vi "runStudy2_2USRP_1ChNCS_3.vi"() -> (2 "Resp Amp":dbl[](graph), 3 "Heart Amp":dbl[](graph), 4 "# queue 2":i32)   [LabVIEW 2016]
uses:
  <instrlib>/niUSRP/niUSRP Timestamp.ctl
  <vilib>/Utility/miscctls.llb/LVDateTimeRec.ctl
  <vilib>/sound2/lvsound2.llb/Sound File Position.ctl
  <vilib>/Analysis/3filter.llb/Filter Passband Type.ctl
  <vilib>/sound2/lvsound2.llb/Sampling Mode.ctl
  <instrlib>/niUSRP/niUSRP Configure Time Start Trigger.vi
  <vilib>/Platform/browser.llb/Open URL in Default Browser (string).vi
  <instrlib>/niUSRP/niUSRP Write Tx Data (CDB).vi
  <instrlib>/niUSRP/niUSRP Fetch Rx Data (CDB).vi
  <vilib>/Analysis/3filter.llb/Butterworth Filter (DBL).vi
  <vilib>/sound2/lvsound2.llb/Sound File Info (path).vi
  <vilib>/sound2/lvsound2.llb/Sound File Read Open.vi
  <vilib>/sound2/lvsound2.llb/Sound File Read (DBL).vi
  <vilib>/sound2/lvsound2.llb/Sound Output Write (DBL).vi
  <vilib>/Analysis/3filter.llb/Butterworth Filter (CDB).vi
  <vilib>/measure/NI_MABase.lvlib
  <vilib>/Analysis/NI_AALBase.lvlib
  <vilib>/Analysis/NI_AALPro.lvlib
panel:
  in  "SDR1\nInitPhase":i32
  in  "Flush Rx2":bool
  out "String 3":string
  out "element":dbl[][](array[numeric])
  out "appended array":dbl[][](array[numeric])
  in  "SDR2 Carrier \nfrequency (Hz)":dbl=1900000000.0
  out "String 2":string
  out "size(s)":i32[](array[numeric])
  in  "Tab Control 7":enum32{"Amp2 @50kHz", "Ph2 @50kHz"}(tab)
  out "Amp2 @50 kHz":dbl[](graph)
  out "Ph2 @50 kHz":dbl[](graph)
  in  "Tab Control 6":enum32{"Amp1 @500Hz", "Ph1 @500Hz"}(tab)
  out "Amp1 @500Hz":dbl[](graph)
  out "Ph1 @500Hz":dbl[](graph)
  out "String":string
  out "#queue 3":i32
  out "#queue 2":i32
  out "# Rx2DS_Queue":i32
  in  "FlushSDR2":bool
  out "error out 2":errorcluster
  in  "Tab Control 8":enum32{"Rx1", "Rx2"}(tab)
  out "IQ Graph":dbl[][](graph)
  out "IQ Graph 2":dbl[][](graph)
  in  "Tab Control 5":enum32{"Amp2 @500Hz", "Ph2 @500Hz"}(tab)
  out "Amp2 @500Hz":dbl[](graph)
  out "Ph2 @500Hz":dbl[](graph)
  in  "Tab Control 4":enum32{"Tx1", "Tx2"}(tab)
  out "Tx1 Waveform Graph":waveform(dbl)[](graph)
  out "Tx2 Waveform graph":waveform(dbl)[](graph)
  in  "Stop 2":bool
  out "Tx2 Waveform":cdb[](array[numeric])
  out "Read:Tx2 IQ Rate":dbl=5000000.0
  out "Read:Rx2 IQ Rate":dbl=5000000.0
  in  "Device2 Name":refnum<k15>="B200mini"
  in  "Tx2 Gain":dbl=26.0 format="%#_6f"
  in  "Rx2 Gain":dbl=20.0 format="%#_6f"
  in  "Routine 3,4":T1=2 items=["Absolute"=0, "Relative"=2]
  in  "(2b) Attn Test":T1=2 items=["Absolute"=0, "Relative"=2]
  in  "Routine 5":T1=2 items=["Absolute"=0, "Relative"=2]
  in  "OpenHTML":bool=TRUE
  in  "Play sound":u16(ring) items=["No sound", "Demo normal breathing", "Demo deep breathing", "Demo fast shallow breathing", "Demo breath hold", "Demo cough", "Demo abdomen movement", "Calibration", "Routine 1", "(2a) Calm music", "(2b) Stress test", "Routine 3/4", "Routine 5"]
  in  "Demo cough":T1=2 items=["Absolute"=0, "Relative"=2]
  in  "Demo breath-hold":T1=2 items=["Absolute"=0, "Relative"=2]
  in  "Demo abdomen":T1=2 items=["Absolute"=0, "Relative"=2]
  in  "Demo fast shallow":T1=2 items=["Absolute"=0, "Relative"=2]
  in  "Play/Stop":bool
  in  "Demo normal":T1=2 items=["Absolute"=0, "Relative"=2]
  in  "Demo deep":T1=2 items=["Absolute"=0, "Relative"=2]
  out "Next Task":string
  out "Calib 5":bool caption="Time has Elapsed"
  out "Calib 4":bool caption="Time has Elapsed"
  out "Calib 3":bool caption="Time has Elapsed"
  in  "Calibration":T1=2 items=["Absolute"=0, "Relative"=2]
  out "Calib 1":bool caption="Time has Elapsed"
  out "Current Task time":dbl(slide) scale=0.0..120.0
  in  "(2a) Calm Music":T1=2 items=["Absolute"=0, "Relative"=2]
  out "#2b":bool caption="Time has Elapsed"
  in  "Routine 1":T1=2 items=["Absolute"=0, "Relative"=2]
  in  "number of samples/ch":i32=5000
  out "#5":bool caption="Time has Elapsed"
  out "#2a":bool caption="Time has Elapsed"
  out "#4":bool caption="Time has Elapsed"
  out "#3":bool caption="Time has Elapsed"
  in  "Comments":string
  in  "Tab Control 3":enum32{"Amp Heart", "Ph Heart"}(tab)
  in  "fh 1":dbl=26.0 format="%0.2f"
  in  "fl 1":dbl=0.7 format="%0.4f"
  out "Heart Ph":dbl[](graph)
  in  "fl 3":dbl=0.7 format="%0.4f"
  in  "fh 3":dbl=26.0 format="%0.2f"
  in  "Tab Control 2":enum32{"Amp1 @50kHz", "Ph1 @50kHz"}(tab)
  out "Amp1 @50 kHz":dbl[](graph)
  out "Ph1 @50 kHz":dbl[](graph)
  in  "Tab Control":enum32{"Amp Resp", "Ph Resp"}(tab)
  in  "fl 2":dbl=15.0 format="%0.4f"
  out "Resp Ph":dbl[](graph)
  in  "fl 4":dbl=15.0 format="%0.4f"
  out "ArraySz":i32[](array[numeric])
  in  "Stop Test":bool
  out "#1":bool caption="Time has Elapsed"
  out "Elapsed Time (s)":dbl
  in  "Routine":u16(ring) items=["Not Running", "Test Run", "Routine1", "Routine2a", "Routine2b", "Routine3", "Routine4", "Routine5", "Calib1", "calib3", "Calib4", "Calib5"]
  out "Read:Tx IQ Rate":dbl=5000000.0
  out "Read:Rx IQ Rate":dbl=5000000.0
  out "date time rec":T2
  out "Total Routine Time":dbl(slide) scale=0.0..420.0
  out "Current Task":string
  in  "Case Number":string="0"
  out "CaseNum":i32=1
  out "Save":bool
  out "Flush":bool
  out "Buffer":bool
  out "Output":i32=1
  out "Ch2 Amplitude":dbl=0.5 step=0.05 format="%#.6g"
  out "Ch1 Amplitude":dbl=0.5 step=0.05 format="%#.6g"
  out "Dis Sampling Rate":dbl=500.0 format="%#_6p"
  in  "DownSamplingRatio 2":i32=100
  out "Sampling Rate":dbl=50000.0 format="%#_6p"
  out "aapp":dbl[][](array[numeric])
  out "IterationNum":i32=1009
  in  "DownSamplingRatio":i32=40
  out "# elements in queue":i32
  out "BW/2":dbl=1000.0
  out "# queue 1":i32
  in  "Dis1":bool=TRUE
  out "Tx1 Waveform":cdb[](array[numeric])
  in  "SDR1 Carrier\nfrequency [Hz]":dbl=1820000000.0 format="%#_6p"
  out "error out":errorcluster
  in  "Start Trigger Time":T3={"whole seconds"=1, "fractional seconds"=0.0}
  in  "Stop":bool
  in  "Channel 2\nTone Amplitude":dbl=0.5 step=0.05 format="%#.6g"
  in  "SDR2\nTone Frequency":dbl=51000.0 format="%#_6p"
  in  "Channel 1\nTone Amplitude":dbl=0.5 step=0.05 format="%#.6g"
  in  "SDR1 \nTone Frequency":dbl=51000.0 format="%#_6p"
  in  "Waveform Size":dbl=20000.0
  in  "Device1 Name":refnum<k15>="MyB200"
  in  "Tx1 Gain":dbl=25.0 format="%#_6f"
  in  "Tx IQ Rate":dbl=2000000.0 format="%#_6p"
  in  "Rx1 Gain 1":dbl=26.0 format="%#_6f"
  in  "Rx IQ Rate":dbl=2000000.0 format="%#_6p"
  # "User Instructions"
  # "User Information"
  # "Routine Selection"
  # "Demo \nSounds"
  # "First Tx-Rx: filtered to get heartbeat signal"
  # "Second Tx-Rx: filtered to get respiration signal"
  # "SDR1"
  # "SDR2"
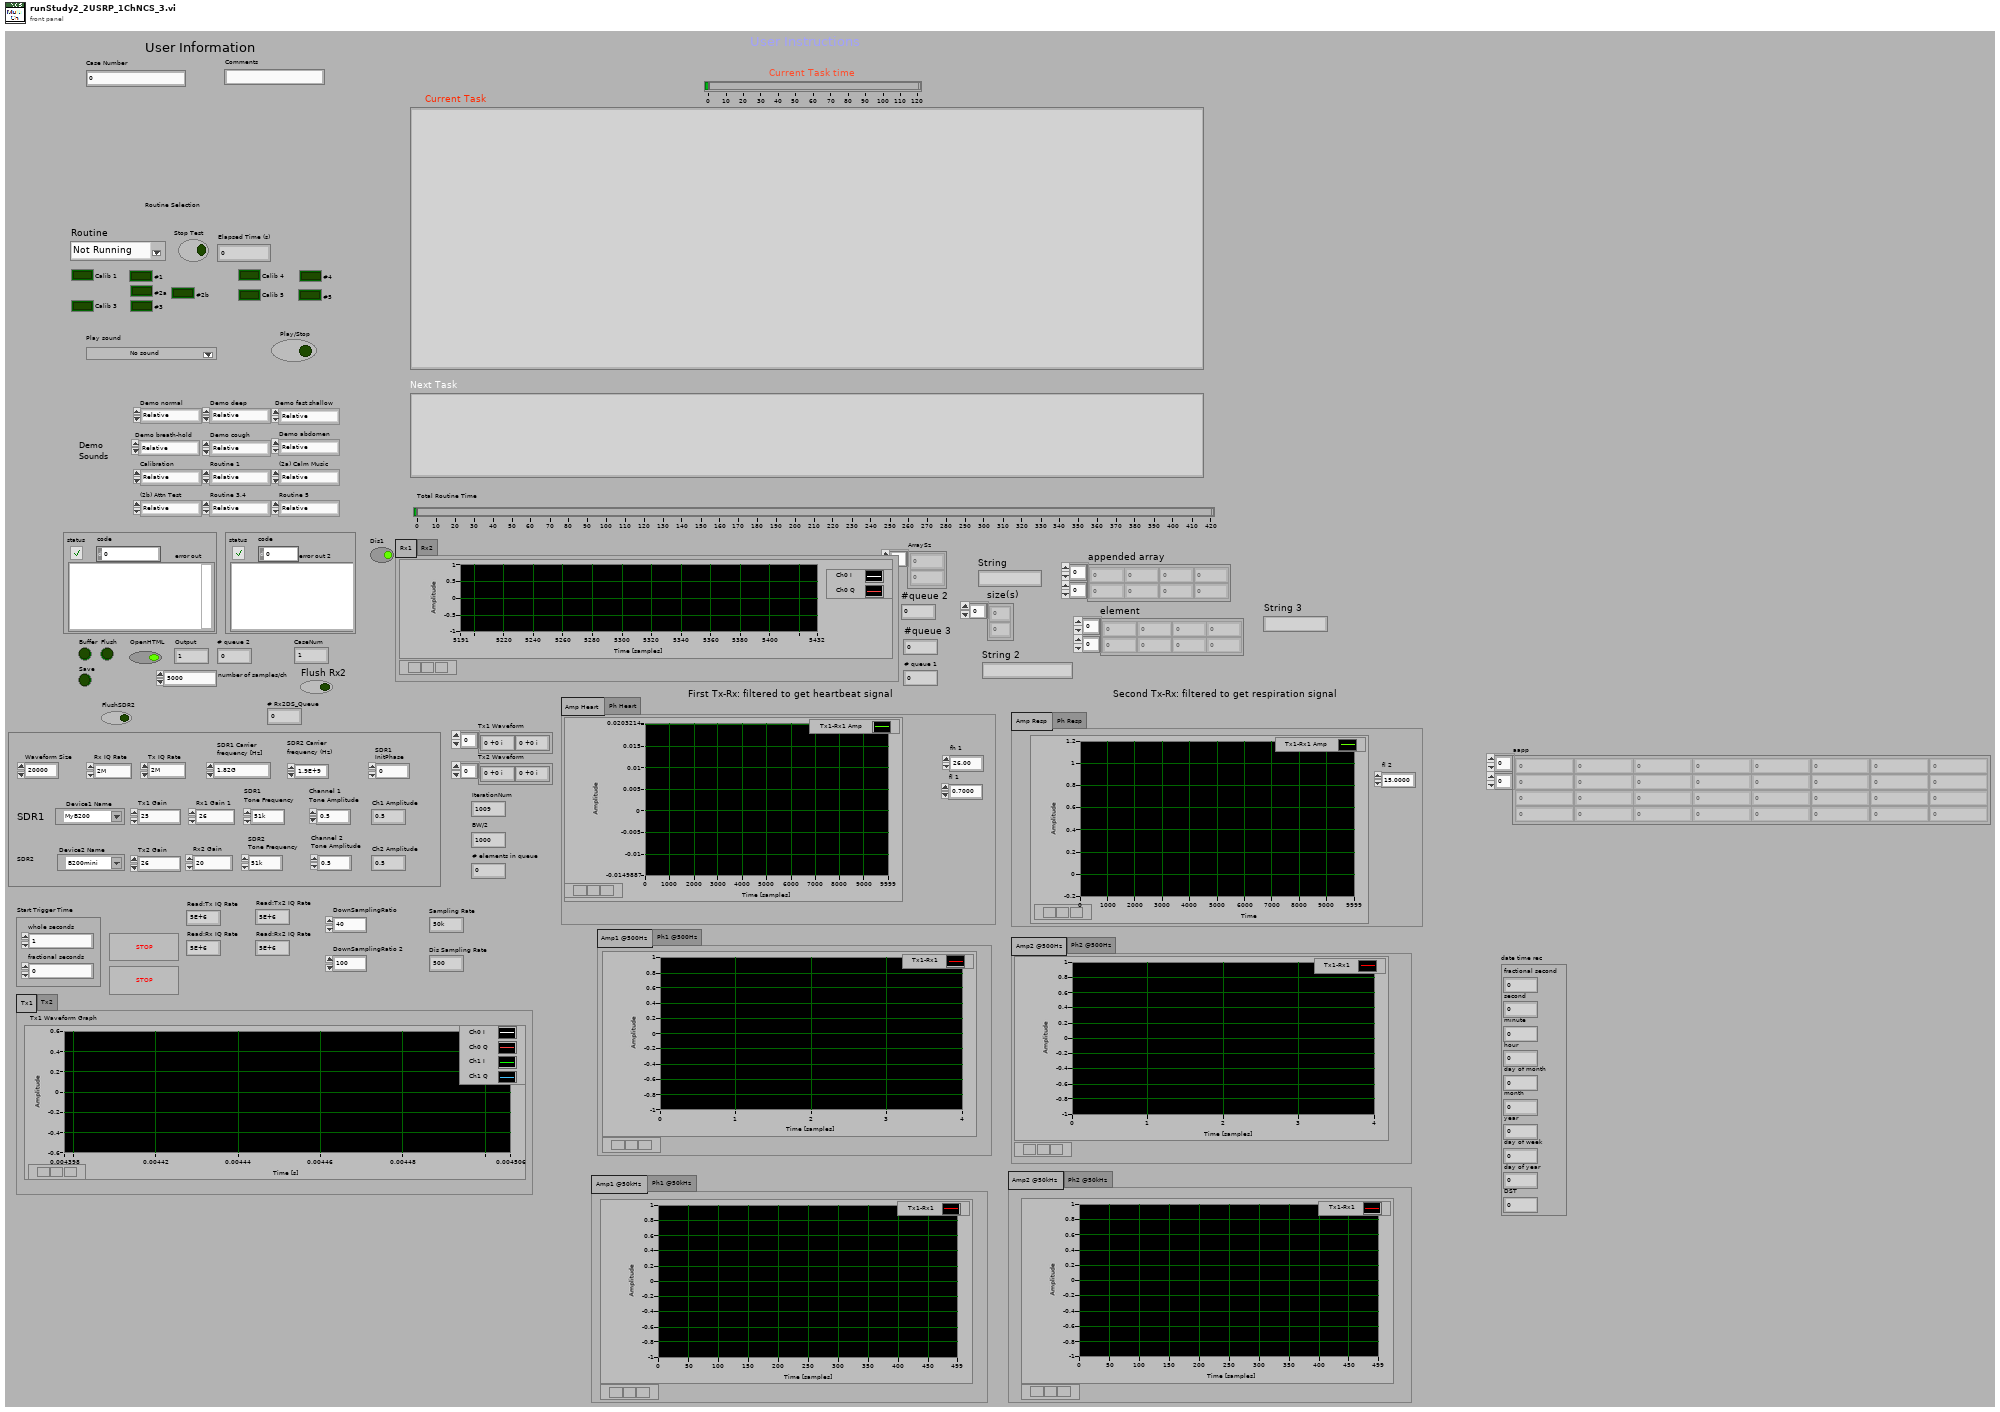
[diagram p1: front panel]
types:
  T1 = typedef "Sound File Position.ctl" = u16
  T2 = typedef "LVDateTimeRec.ctl" = cluster{"fractional second":dbl, "second":i32, "minute":i32, "hour":i32, "day of month":i32, "month":i32, "year":i32, "day of week":i32, "day of year":i32, "DST":i32}
  T3 = typedef "niUSRP Timestamp.ctl" = cluster{"whole seconds":u64, "fractional seconds":dbl}
  T4 = enum16{"Default", "Test", "Routine 1", "Routine 2a", "Routine 2b", "Routine 3", "Routine 4", "Routine 5", "Calib1", "Calib3", "Calib4", "Calib5"}
  T5 = typedef "Sampling Mode.ctl" = i32
  T6 = typedef "Sound Data Format.ctl" = cluster{"sample rate (S/s)":dbl, "number of channels":i32, "bits per sample":i32}
  T7 = typedef "Sound File Refnum.ctl" = refnum<file>
  T8 = typedef "Sound Output Task ID.ctl" = u32
  T9 = typedef "NI_AALBase.lvlib/Filter Passband Type.ctl" = enum32{"Lowpass", "Highpass", "Bandpass", "Bandstop"}
  T10 = enum16{"Default", "Test", "Routine 1", "Routine 2", "Routine 3"}
  T11 = enum16{"Default", "Test", "Routine 1", "Routine 2a", "Routine 2b", "Routine 3a", "Routine 3b", "Routine 4", "Routine 5", "Routine 6", "Routine 7", "Calib1", "Calib3", "Calib4", "Calib5", "Calib7"}
  T12 = enum16{"open", "open or create", "create or replace", "create", "open (read-only)"}
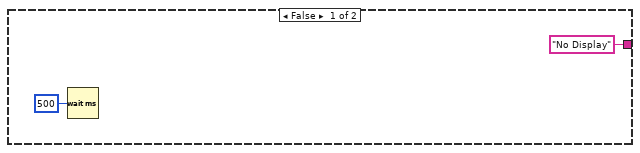
[diagram p2: hidden frame]
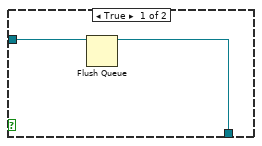
[diagram p3: hidden frame]
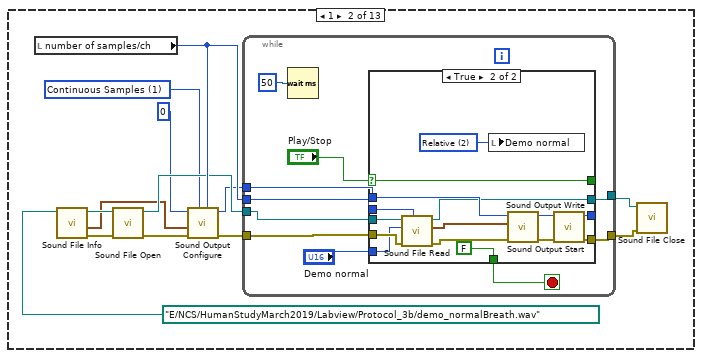
[diagram p5: hidden frame]
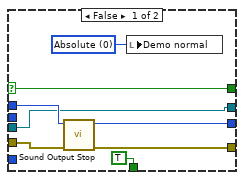
[diagram p6: hidden frame]
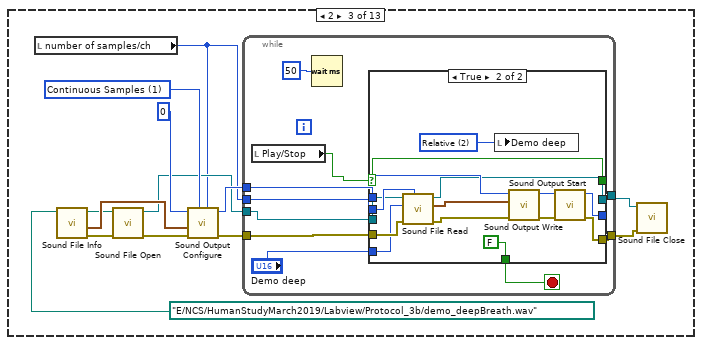
[diagram p7: hidden frame]
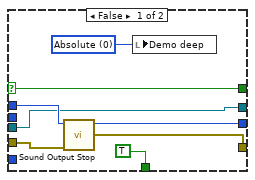
[diagram p8: hidden frame]
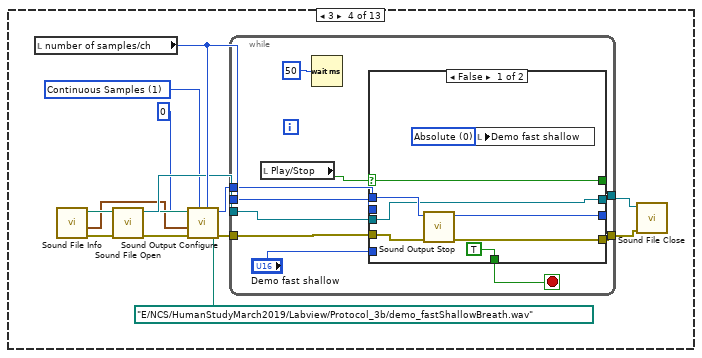
[diagram p9: hidden frame]
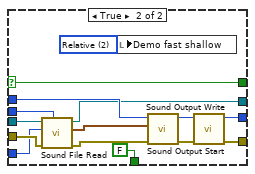
[diagram p10: hidden frame]
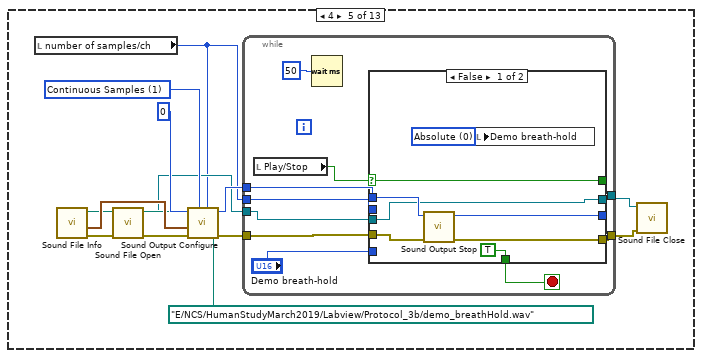
[diagram p11: hidden frame]
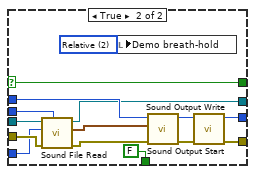
[diagram p12: hidden frame]
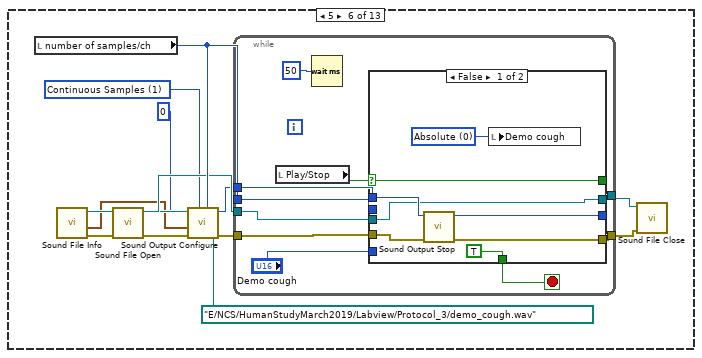
[diagram p13: hidden frame]
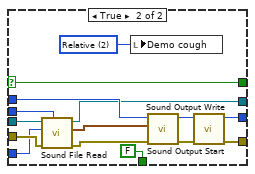
[diagram p14: hidden frame]
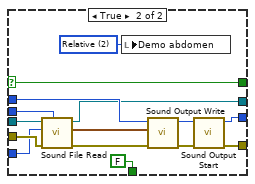
[diagram p15: hidden frame]
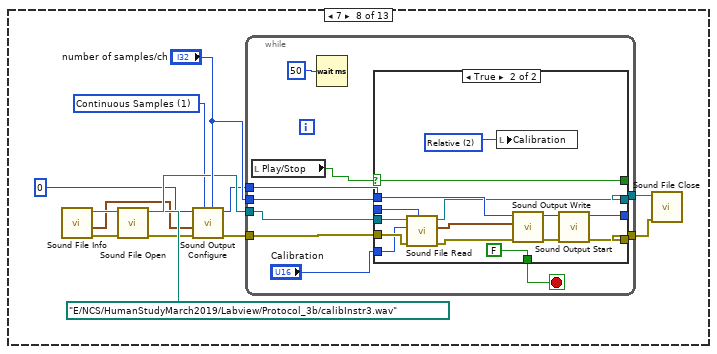
[diagram p16: hidden frame]
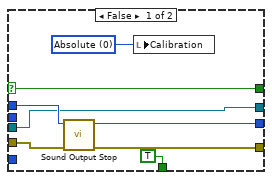
[diagram p17: hidden frame]
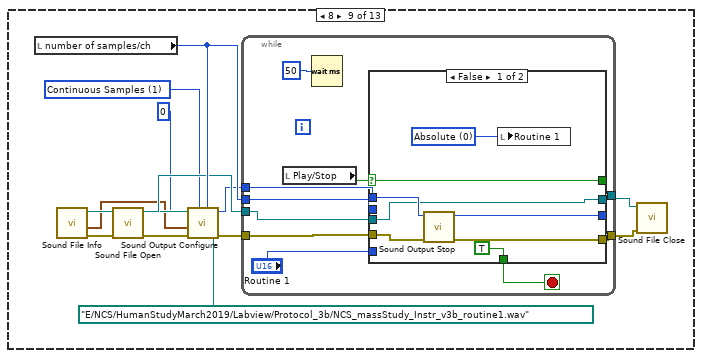
[diagram p18: hidden frame]
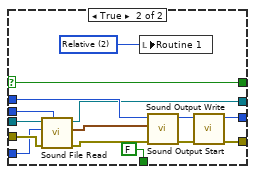
[diagram p19: hidden frame]
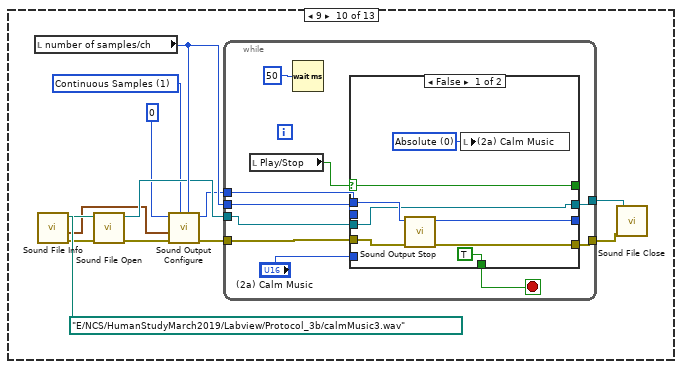
[diagram p20: hidden frame]
diagram:
  w29 = 1 items=["Now", "Next Timebase Edge"] ("apply timestamp")
  w37 = "RX2"  # Rx2 active antenna
  w95 = 0.0 ("element")
  w96 = 2000 ("dimension size")
  w103 = 4 ("dimension size")
  w130 = "RX2"  # Rx1 active antenna
  w164 = 1 items=["Now", "Next Timebase Edge"] ("apply timestamp")
  w78 = "TX1"  # Tx active antenna
  w85 = "0"  # Enabled Channels
  # "Tx2 Chain"
  # "Rx2 chain"
  # "Set the attributes \nspecific to channel 0."
  # "Set the attributes \nused by all Rx channels"
  # "Set the attributes \nspecific to Rx channel 0."
  # "Tx1 Chain"
  # "Rx1 chain"
  # "DownSamplingRatio"
  # "Set the attributes \nspecific to channel 0."
  # "Set the attributes \nused by both Rx channels"
  # "Set the attributes \nspecific to Rx channel 0."
  n1 = while {
    stop <- FALSE stop-if-true
    n2 = local read "Output"() -> (w174:i32)
    n3 = case shown="1" w174 {
      tunnel: [w179 "Channel 1\nTone Amplitude"] -> w176
      tunnel: [w179 "Channel 2\nTone Amplitude"] -> w175
      frame 0, Default {
        w179 = 0.0 ("Channel 1\nTone Amplitude")
      }
      frame 1 {
      }
    }
    "Ch1 Amplitude" <- w176
    "Ch2 Amplitude" <- w175
    n4 = Wait (ms)(milliseconds to wait=u32 50) -> ()  [unwired: 1 out]
  }
  n5 = local read "Device2 Name"() -> (w60:refnum<k15>)
  n6 = local read "Device1 Name"() -> (w169:refnum<k15>)
  n7 = call <instrlib>:"niUSRP Open Rx Session.vi"("device names"="Device2 Name") -> ("session handle out"=w59:refnum<k15>, "error out"=w58:errorcluster)  [unwired: 13 in]
  n8 = property class="niUSRP"(reference=w59, error in=w58, "Enabled Channels"=w85) -> (reference out=w57:refnum<k15>, error out=w56:errorcluster)
  n9 = call <instrlib>:"niUSRP Open Rx Session.vi"("device names"="Device1 Name") -> ("session handle out"=w163:refnum<k15>, "error out"=w162:errorcluster)  [unwired: 13 in]
  n10 = property class="niUSRP"(reference=w163, error in=w162, "Enabled Channels"=w85) -> (reference out=w161:refnum<k15>, error out=w160:errorcluster)
  n11 = call-poly <instrlib>:"niUSRP Configure Trigger.vi"("session handle"=w57, "start trigger time"="Start Trigger Time", "error in (no error)"=w56) -> ("session handle out"=w53:refnum<k15>, "error out"=w52:errorcluster)  [unwired: 11 in]
  n12 = call-poly <instrlib>:"niUSRP Configure Trigger.vi"("session handle"=w161, "start trigger time"="Start Trigger Time", "error in (no error)"=w160) -> ("session handle out"=w157:refnum<k15>, "error out"=w156:errorcluster)  [unwired: 11 in]
  n13 = property class="niUSRP"(reference=w53, error in=w52, "IQ Rate"="Rx IQ Rate") -> (reference out=w50:refnum<k15>, error out=w51:errorcluster)
  n14 = property class="niUSRP"(reference=w157, error in=w156, "IQ Rate"="Rx IQ Rate") -> (reference out=w154:refnum<k15>, error out=w155:errorcluster)
  n15 = property class="niUSRP" props=["Model"](reference=w50, error in=w51) -> (reference out=w48:refnum<k15>, error out=w49:errorcluster)  [unwired: 1 out]
  n16 = property class="niUSRP" props=["Model"](reference=w154, error in=w155) -> (reference out=w152:refnum<k15>, error out=w153:errorcluster)  [unwired: 1 out]
  n17 = property class="niUSRP"(reference=w48, error in=w49, "Carrier Frequency"="SDR2 Carrier \nfrequency (Hz)") -> (reference out=w42:refnum<k15>, error out=w41:errorcluster, "IQ Rate"=→"Read:Rx2 IQ Rate":dbl)
  n18 = property class="niUSRP"(reference=w152, error in=w153, "Carrier Frequency"="SDR1 Carrier\nfrequency [Hz]") -> (reference out=w135:refnum<k15>, error out=w134:errorcluster, "IQ Rate"=→"Read:Rx IQ Rate":dbl)
  n19 = property class="niUSRP"(reference=w42, error in=w41, "Active Channel"="0", "Gain"="Rx2 Gain", "Active Antenna"=w37) -> (reference out=w25:refnum<k15>, error out=w26:errorcluster)
  n20 = call <instrlib>:"niUSRP Open Tx Session.vi"("device names"=w60, "error in (no error)"=w26) -> ("session handle out"=w55:refnum<k15>, "error out"=w54:errorcluster)  [unwired: 12 in]
  n21 = property class="niUSRP"(reference=w55, error in=w54, "Enabled Channels"=w85) -> (reference out=w46:refnum<k15>, error out=w45:errorcluster)
  n22 = property class="niUSRP" props=["IQ Rate", "IQ Rate"](reference=w46, error in=w45, "IQ Rate"="Tx IQ Rate") -> (reference out=w35:refnum<k15>, error out=w34:errorcluster)  [unwired: 1 out]
  n23 = property class="niUSRP"(reference=w35, error in=w34, "Carrier Frequency"="SDR2 Carrier \nfrequency (Hz)") -> (reference out=w39:refnum<k15>, error out=w38:errorcluster, "IQ Rate"=w10:dbl)
  "Read:Tx2 IQ Rate" <- w10
  n24 = property class="niUSRP"(reference=w39, error in=w38, "Active Channel"="0", "Gain"="Tx2 Gain", "Active Antenna"=w78) -> (reference out=w33:refnum<k15>, error out=w32:errorcluster)
  n25 = property class="niUSRP"(reference=w135, error in=w134, "Active Channel"="0", "Gain"="Rx1 Gain 1", "Active Antenna"=w130) -> (reference out=w81:refnum<k15>, error out=w80:errorcluster)
  n26 = call <instrlib>:"niUSRP Open Tx Session.vi"("device names"=w169, "error in (no error)"=w80) -> ("session handle out"=w159:refnum<k15>, "error out"=w158:errorcluster)  [unwired: 12 in]
  n27 = property class="niUSRP"(reference=w159, error in=w158, "Enabled Channels"=w85) -> (reference out=w150:refnum<k15>, error out=w149:errorcluster)
  n28 = property class="niUSRP"(reference=w150, error in=w149, "IQ Rate"="Tx IQ Rate") -> (reference out=w87:refnum<k15>, error out=w86:errorcluster, "IQ Rate"=w148:dbl)
  n29 = property class="niUSRP"(reference=w87, error in=w86, "Carrier Frequency"="SDR1 Carrier\nfrequency [Hz]") -> (reference out=w132:refnum<k15>, error out=w131:errorcluster, "IQ Rate"=→"Read:Tx IQ Rate":dbl)
  n30 = property class="niUSRP"(reference=w132, error in=w131, "Active Channel"="0", "Gain"="Tx1 Gain", "Active Antenna"=w78) -> (reference out=w82:refnum<k15>, error out=w83:errorcluster)
  n31 = call <instrlib>:"niUSRP Commit.vi"("session handle"=w33, "error in (no error)"=w32) -> ("session handle out"=w7:refnum<k15>, "error out"=w24:errorcluster)  [unwired: 12 in]
  n32 = call <instrlib>:"niUSRP Commit.vi"("session handle"=w82, "error in (no error)"=w83) -> ("session handle out"=w171:refnum<k15>, "error out"=w172:errorcluster)  [unwired: 12 in]
  n33 = Merge Errors(w26, w24) -> (w27:errorcluster)
  n34 = call <instrlib>:"niUSRP Set Time.vi"("session handle"=w25, "apply timestamp"=w29, "timestamp"=T3 {"whole seconds"=0, "fractional seconds"=0.0}, "error in (no error)"=w27) -> ("session handle out"=w31:refnum<k15>, "error out"=w30:errorcluster)  [unwired: 10 in]
  n35 = call <instrlib>:"niUSRP Initiate.vi"("session handle"=w31, "error in (no error)"=w30) -> ("session handle out"=w11:refnum<k15>, "error out"=w1:errorcluster)  [unwired: 12 in]
  n36 = Merge Errors(w80, w172) -> (w100:errorcluster)
  n37 = local read "Waveform Size"() -> (w12:dbl)
  n38 = Initialize Array(cdb 0.0+0.0i ("element"), w12) -> (w14:cdb[])
  n39 = call <instrlib>:"niUSRP Set Time.vi"("session handle"=w81, "apply timestamp"=w164, "timestamp"=T3 {"whole seconds"=0, "fractional seconds"=0.0}, "error in (no error)"=w100) -> ("session handle out"=w166:refnum<k15>, "error out"=w165:errorcluster)  [unwired: 10 in]
  n40 = Obtain Queue(max queue size (-1, unlimited)=-1, name (unnamed)="Rx2Queue", element data type=w14) -> (queue out=w71:refnum<queue>)  [unwired: 2 in, 2 out]
  n41 = local read "Waveform Size"() -> (w90:dbl)
  n42 = call <instrlib>:"niUSRP Initiate.vi"("session handle"=w166, "error in (no error)"=w165) -> ("session handle out"=w173:refnum<k15>, "error out"=w88:errorcluster)  [unwired: 12 in]
  n43 = while {
    tunnel: w148 -> [w192]
    tunnel: w88 -> [w187]
    stop <- FALSE stop-if-true
    # "Generate I and Q waveforms."
    n44 = Wait (ms)(milliseconds to wait=u32 100) -> ()  [unwired: 1 out]
    n45 = local read "Ch1 Amplitude"() -> (w186:dbl)
    n46 = Bundle By Name(cluster=cluster{"Fs":dbl, "#s":dbl} {"Fs"=1000.0, "#s"=1000.0} ("sampling info"), "Fs"=w192, "#s"="Waveform Size") -> (w193:cluster{"Fs":dbl, "#s":dbl})
    n47 = Add(x=90.0 ("phase"), y="SDR1\nInitPhase") -> (x+y=w183:dbl)
    n48 = call <vilib>:"Sine Waveform.vi"("sampling info"=w193, "error in (no error)"=w187, "phase"=w183, "amplitude"=w186, "frequency"="SDR1 \nTone Frequency") -> ("error out"=w190:errorcluster, "signal out"=w197:waveform(dbl))  [unwired: 5 in]
    n49 = call <vilib>:"Sine Waveform.vi"("sampling info"=w193, "error in (no error)"=w187, "phase"="SDR1\nInitPhase", "amplitude"=w186, "frequency"="SDR1 \nTone Frequency") -> ("error out"=w191:errorcluster, "signal out"=w198:waveform(dbl))  [unwired: 5 in]
    n50 = Merge Errors(w190, w191) -> ()  [unwired: 1 out]
    n51 = Build Array(w197, w198) -> (→"Tx1 Waveform Graph":waveform(dbl)[])
    n52 = Unbundle By Name(w197) -> ("Y"=w196:dbl[])
    n53 = Unbundle By Name(w198) -> ("Y"=w195:dbl[])
    n54 = Re/Im To Complex(1:w195, 2:w196) -> (0:→"Tx1 Waveform":cdb[])
  }
  n55 = while {
    tunnel: w71 -> [w204]
    stop <- FALSE stop-if-true
    n56 = local read "Dis1"() -> (w203:bool)
    n57 = Wait (ms)(milliseconds to wait=u32 5) -> ()  [unwired: 1 out]
    n58 = case shown="True" w203 {
      tunnel: w204 -> [_ w211]
      tunnel: ["No Display" "Displaying Rx2 "] -> w202
      frame False {
        n59 = Wait (ms)(milliseconds to wait=u32 500) -> ()  [unwired: 1 out]
      }
      frame True {
        n60 = Preview Queue Element(queue=w211) -> (element=w213:cdb[])  [unwired: 2 in, 3 out]
        n61 = for {
          N: 1 -> [_]
          tunnel: w213 -> [w219]
          shift-right: [w216] -> w212
          shift-left: dbl[][] [] -> [w215]
          n62 = Complex To Re/Im(x + iy=w219) -> (x=w218:dbl[], y=w217:dbl[])
          n63 = Build Array (concatenate)(w215, w218, w217) -> (w216:dbl[][])
        }
        "IQ Graph 2" <- w212
      }
    }
    "String" <- w202
  }
  n64 = while {
    tunnel: w11 -> [w231]
    tunnel: w1 -> [w230]
    tunnel: [w226] -> w21
    tunnel: [w229] -> w18
    shift-right: [w222] -> _
    shift-left: w71 -> [w223]
    stop <- w225 stop-if-true
    # "Rx2"
    n65 = local read "Waveform Size"() -> (w224:dbl)
    n66 = call-poly <instrlib>:"niUSRP Fetch Rx Data (poly).vi"("session handle"=w231, "number of samples"=w224, "error in (no error)"=w230) -> ("session handle out"=w229:refnum<k15>, "data"=w220:cdb[], "timestamp"=w221:T3, "error out"=w226:errorcluster)  [unwired: 9 in]
    n67 = call <instrlib>:"niUSRP USRP Timestamp to LV Timestamp.vi"("USRP Timestamp"=w221) -> ()  [unwired: 13 in, 2 out]
    n68 = Enqueue Element(queue=w223, element=w220) -> (queue out=w222:refnum<queue>)  [unwired: 2 in, 2 out]
    n69 = Unbundle By Name(w226) -> ("status"=w228:bool)
    n70 = Or(x=w228, y="Stop 2") -> (x .or. y?=w225:bool)
  }
  n71 = while {
    tunnel: w10 -> [w241]
    tunnel: w1 -> [w232]
    stop <- FALSE stop-if-true
    # "Generate I and Q waveforms."
    n72 = local read "Waveform Size"() -> (w233:dbl)
    n73 = Wait (ms)(milliseconds to wait=u32 100) -> ()  [unwired: 1 out]
    n74 = Bundle By Name(cluster=cluster{"Fs":dbl, "#s":dbl} {"Fs"=1000.0, "#s"=1000.0} ("sampling info"), "Fs"=w241, "#s"=w233) -> (w242:cluster{"Fs":dbl, "#s":dbl})
    n75 = local read "Ch2 Amplitude"() -> (w236:dbl)
    n76 = call <vilib>:"Sine Waveform.vi"("sampling info"=w242, "error in (no error)"=w232, "phase"=90.0, "amplitude"=w236, "frequency"="SDR2\nTone Frequency") -> ("error out"=w239:errorcluster, "signal out"=w247:waveform(dbl))  [unwired: 5 in]
    n77 = call <vilib>:"Sine Waveform.vi"("sampling info"=w242, "error in (no error)"=w232, "amplitude"=w236, "frequency"="SDR2\nTone Frequency") -> ("error out"=w240:errorcluster, "signal out"=w248:waveform(dbl))  [unwired: 6 in]
    n78 = Merge Errors(w239, w240) -> ()  [unwired: 1 out]
    n79 = Build Array(w247, w248) -> (→"Tx2 Waveform graph":waveform(dbl)[])
    n80 = Unbundle By Name(w247) -> ("Y"=w246:dbl[])
    n81 = Unbundle By Name(w248) -> ("Y"=w245:dbl[])
    n82 = Re/Im To Complex(1:w245, 2:w246) -> (0:→"Tx2 Waveform":cdb[])
  }
  n83 = Initialize Array(cdb 0.0+0.0i ("element"), w90) -> (w127:cdb[])
  n84 = Obtain Queue(max queue size (-1, unlimited)=-1, name (unnamed)="Rx1Queue", element data type=w127) -> (queue out=w91:refnum<queue>)  [unwired: 2 in, 2 out]
  n85 = while {
    tunnel: w173 -> [w261]
    tunnel: w88 -> [w260]
    tunnel: [w256] -> w144
    tunnel: [w259] -> w141
    shift-right: [w252] -> _
    shift-left: w91 -> [w253]
    stop <- w255 stop-if-true
    # "Rx"
    n86 = local read "Waveform Size"() -> (w254:dbl)
    n87 = call-poly <instrlib>:"niUSRP Fetch Rx Data (poly).vi"("session handle"=w261, "number of samples"=w254, "error in (no error)"=w260) -> ("session handle out"=w259:refnum<k15>, "data"=w250:cdb[], "timestamp"=w251:T3, "error out"=w256:errorcluster)  [unwired: 9 in]
    n88 = call <instrlib>:"niUSRP USRP Timestamp to LV Timestamp.vi"("USRP Timestamp"=w251) -> ()  [unwired: 13 in, 2 out]
    n89 = Enqueue Element(queue=w253, element=w250) -> (queue out=w252:refnum<queue>)  [unwired: 2 in, 2 out]
    n90 = Unbundle By Name(w256) -> ("status"=w258:bool)
    n91 = Or(x=w258, y="Stop") -> (x .or. y?=w255:bool)
  }
  n92 = while {
    tunnel: w91 -> [w263]
    stop <- FALSE stop-if-true
    n93 = Wait (ms)(milliseconds to wait=u32 5) -> ()  [unwired: 1 out]
    n94 = case shown="True" "Dis1" {
      tunnel: w263 -> [_ w268]
      frame False {
        n95 = Wait (ms)(milliseconds to wait=u32 500) -> ()  [unwired: 1 out]
      }
      frame True {
        n96 = Preview Queue Element(queue=w268) -> (element=w270:cdb[])  [unwired: 2 in, 3 out]
        n97 = for {
          N: 1 -> [_]
          tunnel: w270 -> [w276]
          shift-right: [w273] -> w269
          shift-left: dbl[][] [] -> [w272]
          n98 = Complex To Re/Im(x + iy=w276) -> (x=w275:dbl[], y=w274:dbl[])
          n99 = Build Array (concatenate)(w272, w275, w274) -> (w273:dbl[][])
        }
        "IQ Graph" <- w269
      }
    }
  }
  n100 = while {
    tunnel: w171 -> [w284]
    tunnel: w88 -> [w283]
    tunnel: [w281] -> w146
    tunnel: [w279] -> w139
    stop <- w280 stop-if-true
    # "Tx on SDR1"
    n101 = local read "Tx1 Waveform"() -> (w277:cdb[])
    n102 = local read "Stop"() -> (w278:bool)
    n103 = call-poly <instrlib>:"niUSRP Write Tx Data (poly).vi"("session handle"=w284, "data"=w277, "end of data?"=w278, "error in (no error)"=w283) -> ("session handle out"=w279:refnum<k15>, "error out"=w281:errorcluster)  [unwired: 10 in]
    n104 = Unbundle By Name(w281) -> ("status"=w282:bool)
    n105 = Compound Arithmetic op=OR(w282, w278) -> (w280:bool)
  }
  n106 = while {
    tunnel: w7 -> [w292]
    tunnel: w1 -> [w291]
    tunnel: [w289] -> w5
    tunnel: [w287] -> w6
    stop <- w288 stop-if-true
    # "Tx on SDR2"
    n107 = local read "Tx2 Waveform"() -> (w285:cdb[])
    n108 = local read "Stop 2"() -> (w286:bool)
    n109 = call-poly <instrlib>:"niUSRP Write Tx Data (poly).vi"("session handle"=w292, "data"=w285, "end of data?"=w286, "error in (no error)"=w291) -> ("session handle out"=w287:refnum<k15>, "error out"=w289:errorcluster)  [unwired: 10 in]
    n110 = Unbundle By Name(w289) -> ("status"=w290:bool)
    n111 = Compound Arithmetic op=OR(w290, w286) -> (w288:bool)
  }
  n112 = flat-sequence {
    tunnel: [w294] -> w20
    tunnel: w21 -> [w294]
    tunnel: [w293] -> w19
    tunnel: w18 -> [w293]
    frame #0 {
      n113 = local write "Stop 2"(TRUE ("STOP")) -> ()
    }
  }
  n114 = call <instrlib>:"niUSRP Abort.vi"("session handle"=w19, "error in (no error)"=w20) -> ("session handle out"=w23:refnum<k15>, "error out"=w22:errorcluster)  [unwired: 12 in]
  n115 = flat-sequence {
    tunnel: [w297] -> w145
    tunnel: w146 -> [w297]
    tunnel: [w296] -> w140
    tunnel: w139 -> [w296]
    frame #0 {
      n116 = local write "Stop"(TRUE ("STOP")) -> ()
    }
  }
  n117 = call <instrlib>:"niUSRP Close Session.vi"("session handle"=w23, "error in (no error)"=w22) -> ("error out"=w17:errorcluster)  [unwired: 13 in]
  n118 = flat-sequence {
    tunnel: [w300] -> w143
    tunnel: w144 -> [w300]
    tunnel: [w299] -> w142
    tunnel: w141 -> [w299]
    frame #0 {
      n119 = local write "Stop"(TRUE ("STOP")) -> ()
    }
  }
  n120 = flat-sequence {
    tunnel: w17 -> [w304]
    tunnel: w2 -> [w303]
    tunnel: [w302] -> w75
    frame #0 {
      n121 = Merge Errors(w304, w303) -> (w302:errorcluster)
      n122 = local write "Stop 2"(FALSE ("STOP")) -> ()
    }
  }
  n123 = flat-sequence {
    tunnel: [w307] -> w3
    tunnel: w5 -> [w307]
    tunnel: [w306] -> w4
    tunnel: w6 -> [w306]
    frame #0 {
      n124 = local write "Stop 2"(TRUE ("STOP")) -> ()
    }
  }
  n125 = call <instrlib>:"niUSRP Abort.vi"("session handle"=w142, "error in (no error)"=w143) -> ("session handle out"=w168:refnum<k15>, "error out"=w167:errorcluster)  [unwired: 12 in]
  n126 = call <instrlib>:"niUSRP Close Session.vi"("session handle"=w168, "error in (no error)"=w167) -> ("error out"=w138:errorcluster)  [unwired: 13 in]
  n127 = while {
    stop <- FALSE stop-if-true
    n128 = Wait (ms)(milliseconds to wait=u32 50) -> ()  [unwired: 1 out]
    n129 = case shown="6" "Play sound" {
      frame 0, Default {
      }
      frame 1 {
        w312 = T5 1 items=["Finite Samples", "Continuous Samples"] ("sample mode")
        n130 = local read "number of samples/ch"() -> (w324:i32)
        n131 = call-poly <vilib>:"Sound File Info.vi"("path"=path "E:/NCS/HumanStudyMarch2019/Labview/Protocol_3b/demo_normalBreath.wav") -> ("error out"=w316:errorcluster, "sound format"=w315:T6, "path out"=w317:path)  [unwired: 7 in, 1 out]
        n132 = call-poly <vilib>:"Sound File Open.vi"("error in (no error)"=w316, "path"=w317) -> ("error out"=w313:errorcluster, "sound file refnum"=w321:T7)  [unwired: 8 in]
        n133 = call <vilib>:"Sound Output Configure.vi"("number of samples/ch"=w324, "sample mode"=w312, "error in (no error)"=w313, "sound format"=w315, "device ID"=u32 0) -> ("error out"=w322:errorcluster, "task ID"=w320:T8)  [unwired: 5 in]
        n134 = while {
          tunnel: w320 -> [w334]
          tunnel: [w333] -> w319
          tunnel: w321 -> [w328]
          tunnel: w322 -> [w327]
          tunnel: w324 -> [w329]
          tunnel: [w332] -> w323
          stop <- w325 stop-if-true
          n135 = Wait (ms)(milliseconds to wait=u32 50) -> ()  [unwired: 1 out]
          n136 = case shown="True" "Play/Stop" {
            selector: "Play/Stop" -> [w339 w357]
            tunnel: w334 -> [w342 w354]
            tunnel: [w340 w356] -> w333
            tunnel: [w341 w355] -> _
            tunnel: [w339 w357] -> _
            tunnel: [w337 w351] -> w332
            tunnel: w329 -> [_ w348]
            tunnel: w328 -> [w337 w347]
            tunnel: w327 -> [w338 w346]
            tunnel: "Demo normal" -> [_ w345]
            tunnel: [TRUE FALSE] -> w325
            frame False {
              w336 = T1 0 items=["Absolute"=0, "Relative"=2] ("position mode")
              n137 = call <vilib>:"Sound Output Stop.vi"("error in (no error)"=w338, "task ID"=w342) -> ("error out"=w340:errorcluster, "task ID out"=w341:T8)  [unwired: 8 in]
              n138 = local write "Demo normal"(w336) -> ()
            }
            frame True {
              w344 = T1 2 items=["Absolute"=0, "Relative"=2] ("position mode")
              n139 = call-poly <vilib>:"Sound File Read.vi"("number of samples/ch (-1: all)"=w348, "error in (no error)"=w346, "position mode"=w345, "sound file refnum"=w347) -> ("error out"=w350:errorcluster, "data"=w349:waveform(dbl)[], "sound file refnum out"=w351:T7)  [unwired: 3 in, 2 out]
              n140 = local write "Demo normal"(w344) -> ()
              n141 = call-poly <vilib>:"Sound Output Write.vi"("error in (no error)"=w350, "data"=w349, "task ID"=w354) -> ("error out"=w352:errorcluster, "task ID out"=w353:T8)  [unwired: 7 in]
              n142 = call <vilib>:"Sound Output Start.vi"("error in (no error)"=w352, "task ID"=w353) -> ("error out"=w356:errorcluster, "task ID out"=w355:T8)  [unwired: 8 in]
            }
          }
        }
        n143 = call <vilib>:"Sound File Close.vi"("error in (no error)"=w319, "sound file refnum"=w323) -> ()  [unwired: 9 in, 1 out]
      }
      frame 2 {
        w370 = T5 1 items=["Finite Samples", "Continuous Samples"] ("sample mode")
        n144 = local read "number of samples/ch"() -> (w359:i32)
        n145 = call-poly <vilib>:"Sound File Info.vi"("path"=path "E:/NCS/HumanStudyMarch2019/Labview/Protocol_3b/demo_deepBreath.wav") -> ("error out"=w366:errorcluster, "sound format"=w367:T6, "path out"=w365:path)  [unwired: 7 in, 1 out]
        n146 = call-poly <vilib>:"Sound File Open.vi"("error in (no error)"=w366, "path"=w365) -> ("error out"=w369:errorcluster, "sound file refnum"=w362:T7)  [unwired: 8 in]
        n147 = call <vilib>:"Sound Output Configure.vi"("number of samples/ch"=w359, "sample mode"=w370, "error in (no error)"=w369, "sound format"=w367, "device ID"=u32 0) -> ("error out"=w361:errorcluster, "task ID"=w363:T8)  [unwired: 5 in]
        n148 = while {
          tunnel: w363 -> [w380]
          tunnel: [w379] -> w364
          tunnel: w362 -> [w375]
          tunnel: w361 -> [w374]
          tunnel: w359 -> [w376]
          tunnel: [w378] -> w360
          stop <- w372 stop-if-true
          n149 = local read "Play/Stop"() -> (w371:bool)
          n150 = Wait (ms)(milliseconds to wait=u32 50) -> ()  [unwired: 1 out]
          n151 = case shown="True" w371 {
            selector: w371 -> [w385 w403]
            tunnel: w380 -> [w388 w400]
            tunnel: [w386 w402] -> w379
            tunnel: [w387 w401] -> _
            tunnel: [w385 w403] -> _
            tunnel: [w383 w397] -> w378
            tunnel: w376 -> [_ w394]
            tunnel: w375 -> [w383 w393]
            tunnel: w374 -> [w384 w392]
            tunnel: "Demo deep" -> [_ w391]
            tunnel: [TRUE FALSE] -> w372
            frame False {
              w382 = T1 0 items=["Absolute"=0, "Relative"=2] ("position mode")
              n152 = call <vilib>:"Sound Output Stop.vi"("error in (no error)"=w384, "task ID"=w388) -> ("error out"=w386:errorcluster, "task ID out"=w387:T8)  [unwired: 8 in]
              n153 = local write "Demo deep"(w382) -> ()
            }
            frame True {
              w390 = T1 2 items=["Absolute"=0, "Relative"=2] ("position mode")
              n154 = call-poly <vilib>:"Sound File Read.vi"("number of samples/ch (-1: all)"=w394, "error in (no error)"=w392, "position mode"=w391, "sound file refnum"=w393) -> ("error out"=w396:errorcluster, "data"=w395:waveform(dbl)[], "sound file refnum out"=w397:T7)  [unwired: 3 in, 2 out]
              n155 = local write "Demo deep"(w390) -> ()
              n156 = call-poly <vilib>:"Sound Output Write.vi"("error in (no error)"=w396, "data"=w395, "task ID"=w400) -> ("error out"=w398:errorcluster, "task ID out"=w399:T8)  [unwired: 7 in]
              n157 = call <vilib>:"Sound Output Start.vi"("error in (no error)"=w398, "task ID"=w399) -> ("error out"=w402:errorcluster, "task ID out"=w401:T8)  [unwired: 8 in]
            }
          }
        }
        n158 = call <vilib>:"Sound File Close.vi"("error in (no error)"=w364, "sound file refnum"=w360) -> ()  [unwired: 9 in, 1 out]
      }
      frame 3 {
        w404 = T5 1 items=["Finite Samples", "Continuous Samples"] ("sample mode")
        n159 = local read "number of samples/ch"() -> (w416:i32)
        n160 = call-poly <vilib>:"Sound File Info.vi"("path"=path "E:/NCS/HumanStudyMarch2019/Labview/Protocol_3b/demo_fastShallowBreath.wav") -> ("error out"=w408:errorcluster, "sound format"=w407:T6, "path out"=w409:path)  [unwired: 7 in, 1 out]
        n161 = call-poly <vilib>:"Sound File Open.vi"("error in (no error)"=w408, "path"=w409) -> ("error out"=w405:errorcluster, "sound file refnum"=w413:T7)  [unwired: 8 in]
        n162 = call <vilib>:"Sound Output Configure.vi"("number of samples/ch"=w416, "sample mode"=w404, "error in (no error)"=w405, "sound format"=w407, "device ID"=u32 0) -> ("error out"=w414:errorcluster, "task ID"=w412:T8)  [unwired: 5 in]
        n163 = while {
          tunnel: w412 -> [w426]
          tunnel: [w425] -> w411
          tunnel: w413 -> [w421]
          tunnel: w414 -> [w420]
          tunnel: w416 -> [w422]
          tunnel: [w424] -> w415
          stop <- w418 stop-if-true
          n164 = local read "Play/Stop"() -> (w417:bool)
          n165 = Wait (ms)(milliseconds to wait=u32 50) -> ()  [unwired: 1 out]
          n166 = case shown="False" w417 {
            selector: w417 -> [w431 w449]
            tunnel: w426 -> [w434 w446]
            tunnel: [w432 w448] -> w425
            tunnel: [w433 w447] -> _
            tunnel: [w431 w449] -> _
            tunnel: [w429 w443] -> w424
            tunnel: w422 -> [_ w440]
            tunnel: w421 -> [w429 w439]
            tunnel: w420 -> [w430 w438]
            tunnel: "Demo fast shallow" -> [_ w437]
            tunnel: [TRUE FALSE] -> w418
            frame False {
              w428 = T1 0 items=["Absolute"=0, "Relative"=2] ("position mode")
              n167 = call <vilib>:"Sound Output Stop.vi"("error in (no error)"=w430, "task ID"=w434) -> ("error out"=w432:errorcluster, "task ID out"=w433:T8)  [unwired: 8 in]
              n168 = local write "Demo fast shallow"(w428) -> ()
            }
            frame True {
              w436 = T1 2 items=["Absolute"=0, "Relative"=2] ("position mode")
              n169 = call-poly <vilib>:"Sound File Read.vi"("number of samples/ch (-1: all)"=w440, "error in (no error)"=w438, "position mode"=w437, "sound file refnum"=w439) -> ("error out"=w442:errorcluster, "data"=w441:waveform(dbl)[], "sound file refnum out"=w443:T7)  [unwired: 3 in, 2 out]
              n170 = local write "Demo fast shallow"(w436) -> ()
              n171 = call-poly <vilib>:"Sound Output Write.vi"("error in (no error)"=w442, "data"=w441, "task ID"=w446) -> ("error out"=w444:errorcluster, "task ID out"=w445:T8)  [unwired: 7 in]
              n172 = call <vilib>:"Sound Output Start.vi"("error in (no error)"=w444, "task ID"=w445) -> ("error out"=w448:errorcluster, "task ID out"=w447:T8)  [unwired: 8 in]
            }
          }
        }
        n173 = call <vilib>:"Sound File Close.vi"("error in (no error)"=w411, "sound file refnum"=w415) -> ()  [unwired: 9 in, 1 out]
      }
      frame 4 {
        w462 = T5 1 items=["Finite Samples", "Continuous Samples"] ("sample mode")
        n174 = local read "number of samples/ch"() -> (w450:i32)
        n175 = call-poly <vilib>:"Sound File Info.vi"("path"=path "E:/NCS/HumanStudyMarch2019/Labview/Protocol_3b/demo_breathHold.wav") -> ("error out"=w458:errorcluster, "sound format"=w459:T6, "path out"=w457:path)  [unwired: 7 in, 1 out]
        n176 = call-poly <vilib>:"Sound File Open.vi"("error in (no error)"=w458, "path"=w457) -> ("error out"=w461:errorcluster, "sound file refnum"=w453:T7)  [unwired: 8 in]
        n177 = call <vilib>:"Sound Output Configure.vi"("number of samples/ch"=w450, "sample mode"=w462, "error in (no error)"=w461, "sound format"=w459, "device ID"=u32 0) -> ("error out"=w452:errorcluster, "task ID"=w454:T8)  [unwired: 5 in]
        n178 = while {
          tunnel: w454 -> [w472]
          tunnel: [w471] -> w455
          tunnel: w453 -> [w467]
          tunnel: w452 -> [w466]
          tunnel: w450 -> [w468]
          tunnel: [w470] -> w451
          stop <- w464 stop-if-true
          n179 = local read "Play/Stop"() -> (w463:bool)
          n180 = Wait (ms)(milliseconds to wait=u32 50) -> ()  [unwired: 1 out]
          n181 = case shown="False" w463 {
            selector: w463 -> [w477 w495]
            tunnel: w472 -> [w480 w492]
            tunnel: [w478 w494] -> w471
            tunnel: [w479 w493] -> _
            tunnel: [w477 w495] -> _
            tunnel: [w475 w489] -> w470
            tunnel: w468 -> [_ w486]
            tunnel: w467 -> [w475 w485]
            tunnel: w466 -> [w476 w484]
            tunnel: "Demo breath-hold" -> [_ w483]
            tunnel: [TRUE FALSE] -> w464
            frame False {
              w474 = T1 0 items=["Absolute"=0, "Relative"=2] ("position mode")
              n182 = call <vilib>:"Sound Output Stop.vi"("error in (no error)"=w476, "task ID"=w480) -> ("error out"=w478:errorcluster, "task ID out"=w479:T8)  [unwired: 8 in]
              n183 = local write "Demo breath-hold"(w474) -> ()
            }
            frame True {
              w482 = T1 2 items=["Absolute"=0, "Relative"=2] ("position mode")
              n184 = call-poly <vilib>:"Sound File Read.vi"("number of samples/ch (-1: all)"=w486, "error in (no error)"=w484, "position mode"=w483, "sound file refnum"=w485) -> ("error out"=w488:errorcluster, "data"=w487:waveform(dbl)[], "sound file refnum out"=w489:T7)  [unwired: 3 in, 2 out]
              n185 = local write "Demo breath-hold"(w482) -> ()
              n186 = call-poly <vilib>:"Sound Output Write.vi"("error in (no error)"=w488, "data"=w487, "task ID"=w492) -> ("error out"=w490:errorcluster, "task ID out"=w491:T8)  [unwired: 7 in]
              n187 = call <vilib>:"Sound Output Start.vi"("error in (no error)"=w490, "task ID"=w491) -> ("error out"=w494:errorcluster, "task ID out"=w493:T8)  [unwired: 8 in]
            }
          }
        }
        n188 = call <vilib>:"Sound File Close.vi"("error in (no error)"=w455, "sound file refnum"=w451) -> ()  [unwired: 9 in, 1 out]
      }
      frame 5 {
        w496 = T5 1 items=["Finite Samples", "Continuous Samples"] ("sample mode")
        n189 = local read "number of samples/ch"() -> (w508:i32)
        n190 = call-poly <vilib>:"Sound File Info.vi"("path"=path "E:/NCS/HumanStudyMarch2019/Labview/Protocol_3/demo_cough.wav") -> ("error out"=w500:errorcluster, "sound format"=w499:T6, "path out"=w501:path)  [unwired: 7 in, 1 out]
        n191 = call-poly <vilib>:"Sound File Open.vi"("error in (no error)"=w500, "path"=w501) -> ("error out"=w497:errorcluster, "sound file refnum"=w505:T7)  [unwired: 8 in]
        n192 = call <vilib>:"Sound Output Configure.vi"("number of samples/ch"=w508, "sample mode"=w496, "error in (no error)"=w497, "sound format"=w499, "device ID"=u32 0) -> ("error out"=w506:errorcluster, "task ID"=w504:T8)  [unwired: 5 in]
        n193 = while {
          tunnel: w504 -> [w518]
          tunnel: [w517] -> w503
          tunnel: w505 -> [w513]
          tunnel: w506 -> [w512]
          tunnel: w508 -> [w514]
          tunnel: [w516] -> w507
          stop <- w510 stop-if-true
          n194 = local read "Play/Stop"() -> (w509:bool)
          n195 = Wait (ms)(milliseconds to wait=u32 50) -> ()  [unwired: 1 out]
          n196 = case shown="False" w509 {
            selector: w509 -> [w523 w541]
            tunnel: w518 -> [w526 w538]
            tunnel: [w524 w540] -> w517
            tunnel: [w525 w539] -> _
            tunnel: [w523 w541] -> _
            tunnel: [w521 w535] -> w516
            tunnel: w514 -> [_ w532]
            tunnel: w513 -> [w521 w531]
            tunnel: w512 -> [w522 w530]
            tunnel: "Demo cough" -> [_ w529]
            tunnel: [TRUE FALSE] -> w510
            frame False {
              w520 = T1 0 items=["Absolute"=0, "Relative"=2] ("position mode")
              n197 = call <vilib>:"Sound Output Stop.vi"("error in (no error)"=w522, "task ID"=w526) -> ("error out"=w524:errorcluster, "task ID out"=w525:T8)  [unwired: 8 in]
              n198 = local write "Demo cough"(w520) -> ()
            }
            frame True {
              w528 = T1 2 items=["Absolute"=0, "Relative"=2] ("position mode")
              n199 = call-poly <vilib>:"Sound File Read.vi"("number of samples/ch (-1: all)"=w532, "error in (no error)"=w530, "position mode"=w529, "sound file refnum"=w531) -> ("error out"=w534:errorcluster, "data"=w533:waveform(dbl)[], "sound file refnum out"=w535:T7)  [unwired: 3 in, 2 out]
              n200 = local write "Demo cough"(w528) -> ()
              n201 = call-poly <vilib>:"Sound Output Write.vi"("error in (no error)"=w534, "data"=w533, "task ID"=w538) -> ("error out"=w536:errorcluster, "task ID out"=w537:T8)  [unwired: 7 in]
              n202 = call <vilib>:"Sound Output Start.vi"("error in (no error)"=w536, "task ID"=w537) -> ("error out"=w540:errorcluster, "task ID out"=w539:T8)  [unwired: 8 in]
            }
          }
        }
        n203 = call <vilib>:"Sound File Close.vi"("error in (no error)"=w503, "sound file refnum"=w507) -> ()  [unwired: 9 in, 1 out]
      }
      frame 6 {
        w554 = T5 1 items=["Finite Samples", "Continuous Samples"] ("sample mode")
        n204 = local read "number of samples/ch"() -> (w542:i32)
        n205 = call-poly <vilib>:"Sound File Info.vi"("path"=path "E:/NCS/HumanStudyMarch2019/Labview/Protocol_3b/demo_abdBreathing.wav") -> ("error out"=w550:errorcluster, "sound format"=w551:T6, "path out"=w549:path)  [unwired: 7 in, 1 out]
        n206 = call-poly <vilib>:"Sound File Open.vi"("error in (no error)"=w550, "path"=w549) -> ("error out"=w553:errorcluster, "sound file refnum"=w545:T7)  [unwired: 8 in]
        n207 = call <vilib>:"Sound Output Configure.vi"("number of samples/ch"=w542, "sample mode"=w554, "error in (no error)"=w553, "sound format"=w551, "device ID"=u32 0) -> ("error out"=w544:errorcluster, "task ID"=w546:T8)  [unwired: 5 in]
        n208 = while {
          tunnel: w546 -> [w564]
          tunnel: [w563] -> w547
          tunnel: w545 -> [w559]
          tunnel: w544 -> [w558]
          tunnel: w542 -> [w560]
          tunnel: [w562] -> w543
          stop <- w555 stop-if-true
          n209 = local read "Play/Stop"() -> (w556:bool)
          n210 = Wait (ms)(milliseconds to wait=u32 50) -> ()  [unwired: 1 out]
          n211 = case shown="False" w556 {
            selector: w556 -> [w569 w587]
            tunnel: w564 -> [w572 w584]
            tunnel: [w570 w586] -> w563
            tunnel: [w571 w585] -> _
            tunnel: [w569 w587] -> _
            tunnel: [w567 w581] -> w562
            tunnel: w560 -> [_ w578]
            tunnel: w559 -> [w567 w577]
            tunnel: w558 -> [w568 w576]
            tunnel: "Demo abdomen" -> [_ w575]
            tunnel: [TRUE FALSE] -> w555
            frame False {
              w566 = T1 0 items=["Absolute"=0, "Relative"=2] ("position mode")
              n212 = call <vilib>:"Sound Output Stop.vi"("error in (no error)"=w568, "task ID"=w572) -> ("error out"=w570:errorcluster, "task ID out"=w571:T8)  [unwired: 8 in]
              n213 = local write "Demo abdomen"(w566) -> ()
            }
            frame True {
              w574 = T1 2 items=["Absolute"=0, "Relative"=2] ("position mode")
              n214 = call-poly <vilib>:"Sound File Read.vi"("number of samples/ch (-1: all)"=w578, "error in (no error)"=w576, "position mode"=w575, "sound file refnum"=w577) -> ("error out"=w580:errorcluster, "data"=w579:waveform(dbl)[], "sound file refnum out"=w581:T7)  [unwired: 3 in, 2 out]
              n215 = local write "Demo abdomen"(w574) -> ()
              n216 = call-poly <vilib>:"Sound Output Write.vi"("error in (no error)"=w580, "data"=w579, "task ID"=w584) -> ("error out"=w582:errorcluster, "task ID out"=w583:T8)  [unwired: 7 in]
              n217 = call <vilib>:"Sound Output Start.vi"("error in (no error)"=w582, "task ID"=w583) -> ("error out"=w586:errorcluster, "task ID out"=w585:T8)  [unwired: 8 in]
            }
          }
        }
        n218 = call <vilib>:"Sound File Close.vi"("error in (no error)"=w547, "sound file refnum"=w543) -> ()  [unwired: 9 in, 1 out]
      }
      frame 7 {
        w588 = T5 1 items=["Finite Samples", "Continuous Samples"] ("sample mode")
        n219 = call-poly <vilib>:"Sound File Info.vi"("path"=path "E:/NCS/HumanStudyMarch2019/Labview/Protocol_3b/calibInstr3.wav") -> ("error out"=w592:errorcluster, "sound format"=w591:T6, "path out"=w593:path)  [unwired: 7 in, 1 out]
        n220 = call-poly <vilib>:"Sound File Open.vi"("error in (no error)"=w592, "path"=w593) -> ("error out"=w589:errorcluster, "sound file refnum"=w597:T7)  [unwired: 8 in]
        n221 = call <vilib>:"Sound Output Configure.vi"("number of samples/ch"="number of samples/ch", "sample mode"=w588, "error in (no error)"=w589, "sound format"=w591, "device ID"=u32 0) -> ("error out"=w598:errorcluster, "task ID"=w596:T8)  [unwired: 5 in]
        n222 = while {
          tunnel: w596 -> [w610]
          tunnel: [w609] -> w595
          tunnel: w597 -> [w605]
          tunnel: w598 -> [w604]
          tunnel: "number of samples/ch" -> [w606]
          tunnel: [w608] -> w599
          stop <- w601 stop-if-true
          n223 = local read "Play/Stop"() -> (w602:bool)
          n224 = Wait (ms)(milliseconds to wait=u32 50) -> ()  [unwired: 1 out]
          n225 = case shown="True" w602 {
            selector: w602 -> [w615 w633]
            tunnel: w610 -> [w618 w630]
            tunnel: [w616 w632] -> w609
            tunnel: [w617 w631] -> _
            tunnel: [w615 w633] -> _
            tunnel: [w613 w627] -> w608
            tunnel: w606 -> [_ w624]
            tunnel: w605 -> [w613 w623]
            tunnel: w604 -> [w614 w622]
            tunnel: "Calibration" -> [_ w621]
            tunnel: [TRUE FALSE] -> w601
            frame False {
              w612 = T1 0 items=["Absolute"=0, "Relative"=2] ("position mode")
              n226 = call <vilib>:"Sound Output Stop.vi"("error in (no error)"=w614, "task ID"=w618) -> ("error out"=w616:errorcluster, "task ID out"=w617:T8)  [unwired: 8 in]
              n227 = local write "Calibration"(w612) -> ()
            }
            frame True {
              w620 = T1 2 items=["Absolute"=0, "Relative"=2] ("position mode")
              n228 = call-poly <vilib>:"Sound File Read.vi"("number of samples/ch (-1: all)"=w624, "error in (no error)"=w622, "position mode"=w621, "sound file refnum"=w623) -> ("error out"=w626:errorcluster, "data"=w625:waveform(dbl)[], "sound file refnum out"=w627:T7)  [unwired: 3 in, 2 out]
              n229 = local write "Calibration"(w620) -> ()
              n230 = call-poly <vilib>:"Sound Output Write.vi"("error in (no error)"=w626, "data"=w625, "task ID"=w630) -> ("error out"=w628:errorcluster, "task ID out"=w629:T8)  [unwired: 7 in]
              n231 = call <vilib>:"Sound Output Start.vi"("error in (no error)"=w628, "task ID"=w629) -> ("error out"=w632:errorcluster, "task ID out"=w631:T8)  [unwired: 8 in]
            }
          }
        }
        n232 = call <vilib>:"Sound File Close.vi"("error in (no error)"=w595, "sound file refnum"=w599) -> ()  [unwired: 9 in, 1 out]
      }
      frame 8 {
        w634 = T5 1 items=["Finite Samples", "Continuous Samples"] ("sample mode")
        n233 = local read "number of samples/ch"() -> (w646:i32)
        n234 = call-poly <vilib>:"Sound File Info.vi"("path"=path "E:/NCS/HumanStudyMarch2019/Labview/Protocol_3b/NCS_massStudy_Instr_v3b_routine1.wav") -> ("error out"=w638:errorcluster, "sound format"=w637:T6, "path out"=w639:path)  [unwired: 7 in, 1 out]
        n235 = call-poly <vilib>:"Sound File Open.vi"("error in (no error)"=w638, "path"=w639) -> ("error out"=w635:errorcluster, "sound file refnum"=w643:T7)  [unwired: 8 in]
        n236 = call <vilib>:"Sound Output Configure.vi"("number of samples/ch"=w646, "sample mode"=w634, "error in (no error)"=w635, "sound format"=w637, "device ID"=u32 0) -> ("error out"=w644:errorcluster, "task ID"=w642:T8)  [unwired: 5 in]
        n237 = while {
          tunnel: w642 -> [w656]
          tunnel: [w655] -> w641
          tunnel: w643 -> [w651]
          tunnel: w644 -> [w650]
          tunnel: w646 -> [w652]
          tunnel: [w654] -> w645
          stop <- w647 stop-if-true
          n238 = local read "Play/Stop"() -> (w648:bool)
          n239 = Wait (ms)(milliseconds to wait=u32 50) -> ()  [unwired: 1 out]
          n240 = case shown="False" w648 {
            selector: w648 -> [w661 w679]
            tunnel: w656 -> [w664 w676]
            tunnel: [w662 w678] -> w655
            tunnel: [w663 w677] -> _
            tunnel: [w661 w679] -> _
            tunnel: [w659 w673] -> w654
            tunnel: w652 -> [_ w670]
            tunnel: w651 -> [w659 w669]
            tunnel: w650 -> [w660 w668]
            tunnel: "Routine 1" -> [_ w667]
            tunnel: [TRUE FALSE] -> w647
            frame False {
              w658 = T1 0 items=["Absolute"=0, "Relative"=2] ("position mode")
              n241 = call <vilib>:"Sound Output Stop.vi"("error in (no error)"=w660, "task ID"=w664) -> ("error out"=w662:errorcluster, "task ID out"=w663:T8)  [unwired: 8 in]
              n242 = local write "Routine 1"(w658) -> ()
            }
            frame True {
              w666 = T1 2 items=["Absolute"=0, "Relative"=2] ("position mode")
              n243 = call-poly <vilib>:"Sound File Read.vi"("number of samples/ch (-1: all)"=w670, "error in (no error)"=w668, "position mode"=w667, "sound file refnum"=w669) -> ("error out"=w672:errorcluster, "data"=w671:waveform(dbl)[], "sound file refnum out"=w673:T7)  [unwired: 3 in, 2 out]
              n244 = local write "Routine 1"(w666) -> ()
              n245 = call-poly <vilib>:"Sound Output Write.vi"("error in (no error)"=w672, "data"=w671, "task ID"=w676) -> ("error out"=w674:errorcluster, "task ID out"=w675:T8)  [unwired: 7 in]
              n246 = call <vilib>:"Sound Output Start.vi"("error in (no error)"=w674, "task ID"=w675) -> ("error out"=w678:errorcluster, "task ID out"=w677:T8)  [unwired: 8 in]
            }
          }
        }
        n247 = call <vilib>:"Sound File Close.vi"("error in (no error)"=w641, "sound file refnum"=w645) -> ()  [unwired: 9 in, 1 out]
      }
      frame 9 {
        w680 = T5 1 items=["Finite Samples", "Continuous Samples"] ("sample mode")
        n248 = local read "number of samples/ch"() -> (w692:i32)
        n249 = call-poly <vilib>:"Sound File Info.vi"("path"=path "E:/NCS/HumanStudyMarch2019/Labview/Protocol_3b/calmMusic3.wav") -> ("error out"=w684:errorcluster, "sound format"=w683:T6, "path out"=w685:path)  [unwired: 7 in, 1 out]
        n250 = call-poly <vilib>:"Sound File Open.vi"("error in (no error)"=w684, "path"=w685) -> ("error out"=w681:errorcluster, "sound file refnum"=w689:T7)  [unwired: 8 in]
        n251 = call <vilib>:"Sound Output Configure.vi"("number of samples/ch"=w692, "sample mode"=w680, "error in (no error)"=w681, "sound format"=w683, "device ID"=u32 0) -> ("error out"=w690:errorcluster, "task ID"=w688:T8)  [unwired: 5 in]
        n252 = while {
          tunnel: w688 -> [w702]
          tunnel: [w701] -> w687
          tunnel: w689 -> [w697]
          tunnel: w690 -> [w696]
          tunnel: w692 -> [w698]
          tunnel: [w700] -> w691
          stop <- w693 stop-if-true
          n253 = local read "Play/Stop"() -> (w694:bool)
          n254 = Wait (ms)(milliseconds to wait=u32 50) -> ()  [unwired: 1 out]
          n255 = case shown="False" w694 {
            selector: w694 -> [w707 w725]
            tunnel: w702 -> [w710 w722]
            tunnel: [w708 w724] -> w701
            tunnel: [w709 w723] -> _
            tunnel: [w707 w725] -> _
            tunnel: [w705 w719] -> w700
            tunnel: w698 -> [_ w716]
            tunnel: w697 -> [w705 w715]
            tunnel: w696 -> [w706 w714]
            tunnel: "(2a) Calm Music" -> [_ w713]
            tunnel: [TRUE FALSE] -> w693
            frame False {
              w704 = T1 0 items=["Absolute"=0, "Relative"=2] ("position mode")
              n256 = call <vilib>:"Sound Output Stop.vi"("error in (no error)"=w706, "task ID"=w710) -> ("error out"=w708:errorcluster, "task ID out"=w709:T8)  [unwired: 8 in]
              n257 = local write "(2a) Calm Music"(w704) -> ()
            }
            frame True {
              w712 = T1 2 items=["Absolute"=0, "Relative"=2] ("position mode")
              n258 = call-poly <vilib>:"Sound File Read.vi"("number of samples/ch (-1: all)"=w716, "error in (no error)"=w714, "position mode"=w713, "sound file refnum"=w715) -> ("error out"=w718:errorcluster, "data"=w717:waveform(dbl)[], "sound file refnum out"=w719:T7)  [unwired: 3 in, 2 out]
              n259 = local write "(2a) Calm Music"(w712) -> ()
              n260 = call-poly <vilib>:"Sound Output Write.vi"("error in (no error)"=w718, "data"=w717, "task ID"=w722) -> ("error out"=w720:errorcluster, "task ID out"=w721:T8)  [unwired: 7 in]
              n261 = call <vilib>:"Sound Output Start.vi"("error in (no error)"=w720, "task ID"=w721) -> ("error out"=w724:errorcluster, "task ID out"=w723:T8)  [unwired: 8 in]
            }
          }
        }
        n262 = call <vilib>:"Sound File Close.vi"("error in (no error)"=w687, "sound file refnum"=w691) -> ()  [unwired: 9 in, 1 out]
      }
      frame 10 {
        w738 = T5 1 items=["Finite Samples", "Continuous Samples"] ("sample mode")
        n263 = local read "number of samples/ch"() -> (w726:i32)
        n264 = call-poly <vilib>:"Sound File Info.vi"("path"=path "E:/NCS/HumanStudyMarch2019/Labview/Protocol_3b/attentionTestInstr.wav") -> ("error out"=w734:errorcluster, "sound format"=w735:T6, "path out"=w733:path)  [unwired: 7 in, 1 out]
        n265 = call-poly <vilib>:"Sound File Open.vi"("error in (no error)"=w734, "path"=w733) -> ("error out"=w737:errorcluster, "sound file refnum"=w729:T7)  [unwired: 8 in]
        n266 = call <vilib>:"Sound Output Configure.vi"("number of samples/ch"=w726, "sample mode"=w738, "error in (no error)"=w737, "sound format"=w735, "device ID"=u32 0) -> ("error out"=w728:errorcluster, "task ID"=w730:T8)  [unwired: 5 in]
        n267 = while {
          tunnel: w730 -> [w748]
          tunnel: [w747] -> w731
          tunnel: w729 -> [w743]
          tunnel: w728 -> [w742]
          tunnel: w726 -> [w744]
          tunnel: [w746] -> w727
          stop <- w739 stop-if-true
          n268 = local read "Play/Stop"() -> (w740:bool)
          n269 = Wait (ms)(milliseconds to wait=u32 50) -> ()  [unwired: 1 out]
          n270 = case shown="False" w740 {
            selector: w740 -> [w753 w771]
            tunnel: w748 -> [w756 w768]
            tunnel: [w754 w770] -> w747
            tunnel: [w755 w769] -> _
            tunnel: [w753 w771] -> _
            tunnel: [w751 w765] -> w746
            tunnel: w744 -> [_ w762]
            tunnel: w743 -> [w751 w761]
            tunnel: w742 -> [w752 w760]
            tunnel: "(2b) Attn Test" -> [_ w759]
            tunnel: [TRUE FALSE] -> w739
            frame False {
              w750 = T1 0 items=["Absolute"=0, "Relative"=2] ("position mode")
              n271 = call <vilib>:"Sound Output Stop.vi"("error in (no error)"=w752, "task ID"=w756) -> ("error out"=w754:errorcluster, "task ID out"=w755:T8)  [unwired: 8 in]
              n272 = local write "(2b) Attn Test"(w750) -> ()
            }
            frame True {
              w758 = T1 2 items=["Absolute"=0, "Relative"=2] ("position mode")
              n273 = call-poly <vilib>:"Sound File Read.vi"("number of samples/ch (-1: all)"=w762, "error in (no error)"=w760, "position mode"=w759, "sound file refnum"=w761) -> ("error out"=w764:errorcluster, "data"=w763:waveform(dbl)[], "sound file refnum out"=w765:T7)  [unwired: 3 in, 2 out]
              n274 = local write "(2b) Attn Test"(w758) -> ()
              n275 = call-poly <vilib>:"Sound Output Write.vi"("error in (no error)"=w764, "data"=w763, "task ID"=w768) -> ("error out"=w766:errorcluster, "task ID out"=w767:T8)  [unwired: 7 in]
              n276 = call <vilib>:"Sound Output Start.vi"("error in (no error)"=w766, "task ID"=w767) -> ("error out"=w770:errorcluster, "task ID out"=w769:T8)  [unwired: 8 in]
            }
          }
        }
        n277 = call <vilib>:"Sound File Close.vi"("error in (no error)"=w731, "sound file refnum"=w727) -> ()  [unwired: 9 in, 1 out]
      }
      frame 11 {
        w784 = T5 1 items=["Finite Samples", "Continuous Samples"] ("sample mode")
        n278 = local read "number of samples/ch"() -> (w772:i32)
        n279 = call-poly <vilib>:"Sound File Info.vi"("path"=path "E:/NCS/HumanStudyMarch2019/Labview/Protocol_3b/NCS_massStudy_Instr_v3_routine3_4.wav") -> ("error out"=w780:errorcluster, "sound format"=w781:T6, "path out"=w779:path)  [unwired: 7 in, 1 out]
        n280 = call-poly <vilib>:"Sound File Open.vi"("error in (no error)"=w780, "path"=w779) -> ("error out"=w783:errorcluster, "sound file refnum"=w775:T7)  [unwired: 8 in]
        n281 = call <vilib>:"Sound Output Configure.vi"("number of samples/ch"=w772, "sample mode"=w784, "error in (no error)"=w783, "sound format"=w781, "device ID"=u32 0) -> ("error out"=w774:errorcluster, "task ID"=w776:T8)  [unwired: 5 in]
        n282 = while {
          tunnel: w776 -> [w794]
          tunnel: [w793] -> w777
          tunnel: w775 -> [w789]
          tunnel: w774 -> [w788]
          tunnel: w772 -> [w790]
          tunnel: [w792] -> w773
          stop <- w785 stop-if-true
          n283 = local read "Play/Stop"() -> (w786:bool)
          n284 = Wait (ms)(milliseconds to wait=u32 50) -> ()  [unwired: 1 out]
          n285 = case shown="False" w786 {
            selector: w786 -> [w799 w817]
            tunnel: w794 -> [w802 w814]
            tunnel: [w800 w816] -> w793
            tunnel: [w801 w815] -> _
            tunnel: [w799 w817] -> _
            tunnel: [w797 w811] -> w792
            tunnel: w790 -> [_ w808]
            tunnel: w789 -> [w797 w807]
            tunnel: w788 -> [w798 w806]
            tunnel: "Routine 3,4" -> [_ w805]
            tunnel: [TRUE FALSE] -> w785
            frame False {
              w796 = T1 0 items=["Absolute"=0, "Relative"=2] ("position mode")
              n286 = call <vilib>:"Sound Output Stop.vi"("error in (no error)"=w798, "task ID"=w802) -> ("error out"=w800:errorcluster, "task ID out"=w801:T8)  [unwired: 8 in]
              n287 = local write "Routine 3,4"(w796) -> ()
            }
            frame True {
              w804 = T1 2 items=["Absolute"=0, "Relative"=2] ("position mode")
              n288 = call-poly <vilib>:"Sound File Read.vi"("number of samples/ch (-1: all)"=w808, "error in (no error)"=w806, "position mode"=w805, "sound file refnum"=w807) -> ("error out"=w810:errorcluster, "data"=w809:waveform(dbl)[], "sound file refnum out"=w811:T7)  [unwired: 3 in, 2 out]
              n289 = local write "Routine 3,4"(w804) -> ()
              n290 = call-poly <vilib>:"Sound Output Write.vi"("error in (no error)"=w810, "data"=w809, "task ID"=w814) -> ("error out"=w812:errorcluster, "task ID out"=w813:T8)  [unwired: 7 in]
              n291 = call <vilib>:"Sound Output Start.vi"("error in (no error)"=w812, "task ID"=w813) -> ("error out"=w816:errorcluster, "task ID out"=w815:T8)  [unwired: 8 in]
            }
          }
        }
        n292 = call <vilib>:"Sound File Close.vi"("error in (no error)"=w777, "sound file refnum"=w773) -> ()  [unwired: 9 in, 1 out]
      }
      frame 12 {
        w819 = T5 1 items=["Finite Samples", "Continuous Samples"] ("sample mode")
        n293 = local read "number of samples/ch"() -> (w818:i32)
        n294 = call-poly <vilib>:"Sound File Info.vi"("path"=path "E:/NCS/HumanStudyMarch2019/Labview/Protocol_3/NCS_massStudy_Instr_v3_routine5.wav") -> ("error out"=w823:errorcluster, "sound format"=w822:T6, "path out"=w824:path)  [unwired: 7 in, 1 out]
        n295 = call-poly <vilib>:"Sound File Open.vi"("error in (no error)"=w823, "path"=w824) -> ("error out"=w820:errorcluster, "sound file refnum"=w828:T7)  [unwired: 8 in]
        n296 = call <vilib>:"Sound Output Configure.vi"("number of samples/ch"=w818, "sample mode"=w819, "error in (no error)"=w820, "sound format"=w822, "device ID"=u32 0) -> ("error out"=w829:errorcluster, "task ID"=w827:T8)  [unwired: 5 in]
        n297 = while {
          tunnel: w827 -> [w840]
          tunnel: [w839] -> w826
          tunnel: w828 -> [w835]
          tunnel: w829 -> [w834]
          tunnel: w818 -> [w836]
          tunnel: [w838] -> w830
          stop <- w831 stop-if-true
          n298 = local read "Play/Stop"() -> (w832:bool)
          n299 = Wait (ms)(milliseconds to wait=u32 50) -> ()  [unwired: 1 out]
          n300 = case shown="False" w832 {
            selector: w832 -> [w845 w863]
            tunnel: w840 -> [w848 w860]
            tunnel: [w846 w862] -> w839
            tunnel: [w847 w861] -> _
            tunnel: [w845 w863] -> _
            tunnel: [w843 w857] -> w838
            tunnel: w836 -> [_ w854]
            tunnel: w835 -> [w843 w853]
            tunnel: w834 -> [w844 w852]
            tunnel: "Routine 5" -> [_ w851]
            tunnel: [TRUE FALSE] -> w831
            frame False {
              w842 = T1 0 items=["Absolute"=0, "Relative"=2] ("position mode")
              n301 = call <vilib>:"Sound Output Stop.vi"("error in (no error)"=w844, "task ID"=w848) -> ("error out"=w846:errorcluster, "task ID out"=w847:T8)  [unwired: 8 in]
              n302 = local write "Routine 5"(w842) -> ()
            }
            frame True {
              w850 = T1 2 items=["Absolute"=0, "Relative"=2] ("position mode")
              n303 = call-poly <vilib>:"Sound File Read.vi"("number of samples/ch (-1: all)"=w854, "error in (no error)"=w852, "position mode"=w851, "sound file refnum"=w853) -> ("error out"=w856:errorcluster, "data"=w855:waveform(dbl)[], "sound file refnum out"=w857:T7)  [unwired: 3 in, 2 out]
              n304 = local write "Routine 5"(w850) -> ()
              n305 = call-poly <vilib>:"Sound Output Write.vi"("error in (no error)"=w856, "data"=w855, "task ID"=w860) -> ("error out"=w858:errorcluster, "task ID out"=w859:T8)  [unwired: 7 in]
              n306 = call <vilib>:"Sound Output Start.vi"("error in (no error)"=w858, "task ID"=w859) -> ("error out"=w862:errorcluster, "task ID out"=w861:T8)  [unwired: 8 in]
            }
          }
        }
        n307 = call <vilib>:"Sound File Close.vi"("error in (no error)"=w826, "sound file refnum"=w830) -> ()  [unwired: 9 in, 1 out]
      }
    }
  }
  n308 = call <instrlib>:"niUSRP Close Session.vi"("session handle"=w140, "error in (no error)"=w145) -> ("error out"=w137:errorcluster)  [unwired: 13 in]
  n309 = flat-sequence {
    tunnel: w138 -> [w866]
    tunnel: w137 -> [w865]
    tunnel: [w864] -> w76
    frame #0 {
      n310 = Merge Errors(w866, w865) -> (w864:errorcluster)
      n311 = local write "Stop"(FALSE ("STOP")) -> ()
    }
  }
  n312 = call <instrlib>:"niUSRP Close Session.vi"("session handle"=w4, "error in (no error)"=w3) -> ("error out"=w2:errorcluster)  [unwired: 13 in]
  n313 = local read "Rx IQ Rate"() -> (w107:dbl)
  n314 = Divide(x=2000.0, y=2.0) -> (x/y=→"BW/2":dbl)
  n315 = local read "Waveform Size"() -> (w119:dbl)
  n316 = Divide(x=w107, y="DownSamplingRatio") -> (x/y=→"Sampling Rate":dbl)
  n317 = Divide(x=w119, y="DownSamplingRatio") -> (x/y=w102:dbl)
  n318 = Initialize Array(0.0 ("element"), w103, w102) -> (w120:dbl[][])
  n319 = Initialize Array(0.0 ("element"), w103, w102) -> (w109:dbl[][])
  n320 = Obtain Queue "Display Queue"(name (unnamed)="DispQueue", element data type=w120) -> (queue out=w89:refnum<queue>)  [unwired: 3 in, 2 out]
  n321 = Obtain Queue "Saving Queue"(name (unnamed)="SaveBuffer", element data type=w109) -> (queue out=w108:refnum<queue>)  [unwired: 3 in, 2 out]
  n322 = local read "Rx IQ Rate"() -> (w72:dbl)
  n323 = local read "SDR1 \nTone Frequency"() -> (w97:dbl)
  n324 = local read "DownSamplingRatio"() -> (w65:i32)
  n325 = local read "Waveform Size"() -> (w74:dbl)
  n326 = local read "Waveform Size"() -> (w66:dbl)
  n327 = Divide(x=w66, y=w65) -> (x/y=w64:dbl)
  n328 = local read "SDR2\nTone Frequency"() -> (w73:dbl)
  n329 = Initialize Array(0.0 ("element"), 2 ("dimension size"), w64) -> (w69:dbl[][])
  n330 = Obtain Queue(max queue size (-1, unlimited)=-1, name (unnamed)="Rx2DS_Queue", element data type=w69) -> (queue out=w62:refnum<queue>)  [unwired: 2 in, 2 out]
  n331 = while {
    tunnel: w91 -> [w912]
    tunnel: w108 -> [w901]
    tunnel: w74 -> [w896]
    tunnel: w97 -> [w883]
    tunnel: w72 -> [w895]
    tunnel: w89 -> [w882]
    tunnel: w62 -> [w875]
    stop <- FALSE stop-if-true
    # "The order is changed to amp1 - amp2 - ph1 - ph2"
    # "Downsampling the NCS signal"
    # "Getting the amplitude and phase from I and Q"
    # "Rx 1 - Tx 1"
    # "Tx1 to Rx1 QueInd_0"
    # "100 times"
    n332 = call "NCS_IQ_OneTx.vi"("Coerced IQ rate"=w895, "Waveform Size"=w896, "Channel 0\nTone Frequency"=w883, "Channel 0\nTone Amplitude"=1) -> ("IQ waveform array"=w873:cdb[])  [unwired: 4 in, 2 out]
    n333 = Dequeue Element(queue=w912) -> (element=w881:cdb[])  [unwired: 2 in, 3 out]
    n334 = Get Queue Status(queue=w912) -> (# elements in queue=→"# queue 1":i32)  [unwired: 2 in, 7 out]
    n335 = local read "SDR1 \nTone Frequency"() -> (w909:dbl)
    n336 = local read "BW/2"() -> (w904:dbl)
    n337 = local read "Rx IQ Rate"() -> (w900:dbl)
    n338 = Get Queue Status(queue=w875) -> (queue out=w874:refnum<queue>, # elements in queue=→"# Rx2DS_Queue":i32)  [unwired: 2 in, 6 out]
    n339 = case shown="True" "Flush Rx2" {
      tunnel: [w919 w922] -> w871
      tunnel: [w917 w922] -> w870
      tunnel: w874 -> [w916 w927]
      tunnel: ["Dequeing Rx2" "Flushing Rx2"] -> w869
      frame False {
        n340 = Dequeue Element(queue=w916) -> (element=w915:dbl[][])  [unwired: 2 in, 3 out]
        "element" <- w915
        n341 = Index Array(array=w915, index (row)=0 ("index")) -> (element=w919:dbl[])  [unwired: 1 in]
        n342 = Index Array(array=w915, index (row)=1) -> (element=w917:dbl[])  [unwired: 1 in]
      }
      frame True {
        n343 = Flush Queue(queue=w927) -> ()  [unwired: 1 in, 3 out]
        n344 = local read "DownSamplingRatio"() -> (w924:i32)
        n345 = local read "Waveform Size"() -> (w925:dbl)
        n346 = Divide(x=w925, y=w924) -> (x/y=w923:dbl)
        n347 = Initialize Array(0.0, w923) -> (w922:dbl[])
      }
    }
    "String 3" <- w869
    n348 = Subtract(x=w909, y=w904) -> (x-y=w910:dbl)
    n349 = Add(x=w909, y=w904) -> (x+y=w911:dbl)
    n350 = Complex To Polar(r * e^(i*theta)=w873) -> (theta=w892:dbl[])  [unwired: 1 out]
    n351 = call-poly <vilib>:"Butterworth Filter.vi"("init/cont (init:F)"=TRUE, "order"=2, "filter type"=Filter_Passband_Type."Bandpass", "low cutoff freq: fl"=w910, "high cutoff freq: fh"=w911, "sampling freq: fs"=w900, "X"=w881) -> ("Filtered X"=w906:cdb[])  [unwired: 1 in, 1 out]
    n352 = Complex To Polar(r * e^(i*theta)=w906) -> (r=w903:dbl[], theta=w891:dbl[])
    n353 = Subtract(x=w891, y=w892) -> (x-y=w894:dbl[])
    n354 = call <vilib>:"Unwrap Phase.vi"("phase unit"=1 ("y"), "Phase"=w894) -> ("Unwrapped Phase"=w889:dbl[])  [unwired: 8 in, 1 out]
    n355 = local read "DownSamplingRatio"() -> (w885:i32)
    n356 = local read "Waveform Size"() -> (w899:dbl)
    n357 = Divide(x=w899, y=w885) -> (x/y=w888:dbl)
    n358 = Reshape Array(w903, w888, w885) -> (w890:dbl[][])
    n359 = Reshape Array(w889, w888, w885) -> (w887:dbl[][])
    n360 = for {
      tunnel: w890 -> [w940] mode=indexing
      tunnel: [w939] -> w902 mode=indexing
      tunnel: w887 -> [w938] mode=indexing
      tunnel: [w937] -> w886 mode=indexing
      n361 = Add Array Elements(numeric array=w940) -> (sum=w939:dbl)
      n362 = Add Array Elements(numeric array=w938) -> (sum=w937:dbl)
    }
    n363 = Divide(x=w902, y=w885) -> (x/y=w879:dbl[])
    n364 = Divide(x=w886, y=w885) -> (x/y=w878:dbl[])
    n365 = Build Array(w879, w871, w878, w870) -> (w880:dbl[][])
    n366 = disable-structure shown="Enabled" {
      disable-tunnel: w879 -> [w931 _]
      disable-tunnel: w878 -> [w930 _]
      disable-tunnel: w871 -> [w929 _]
      disable-tunnel: w870 -> [w928 _]
      frame Enabled {
        "Amp1 @50 kHz" <- w931
        "Ph1 @50 kHz" <- w930
        "Ph2 @50 kHz" <- w928
        "Amp2 @50 kHz" <- w929
      }
      frame Disabled {
      }
    }
    n367 = Array Size(array=w880) -> (size(s)=→"ArraySz":i32[])
    n368 = local read "Flush"() -> (w897:bool)
    n369 = local read "Buffer"() -> (w898:bool)
    n370 = Enqueue Element(queue=w882, element=w880) -> ()  [unwired: 2 in, 3 out]
    n371 = case shown="True" w898 {
      tunnel: w901 -> [w933 w936]
      tunnel: w880 -> [_ w935]
      tunnel: w897 -> [w932 _]
      frame False {
        n372 = case shown="False" w932 {
          tunnel: w933 -> [_ w934]
          frame False {
          }
          frame True {
            n373 = Flush Queue(queue=w934) -> ()  [unwired: 1 in, 3 out]
          }
        }
      }
      frame True {
        n374 = Enqueue Element(queue=w936, element=w935) -> ()  [unwired: 2 in, 3 out]
      }
    }
  }
  n375 = while {
    tunnel: w74 -> [w956]
    tunnel: w73 -> [w954]
    tunnel: w72 -> [w953]
    tunnel: w71 -> [w947]
    shift-right: [w945] -> _
    shift-left: w62 -> [w950]
    stop <- FALSE stop-if-true
    # "Rx 2 - Tx 2"
    # "Tx2 to Rx2 QueInd_0"
    # "100 times"
    n376 = call "NCS_IQ_OneTx.vi"("Coerced IQ rate"=w953, "Waveform Size"=w956, "Channel 0\nTone Frequency"=w954, "Channel 0\nTone Amplitude"=1) -> ("IQ waveform array"=w944:cdb[])  [unwired: 4 in, 2 out]
    n377 = Get Queue Status(queue=w947) -> (# elements in queue=→"#queue 3":i32)  [unwired: 2 in, 7 out]
    n378 = Dequeue Element(queue=w947) -> (element=w979:cdb[])  [unwired: 2 in, 3 out]
    n379 = local read "SDR2\nTone Frequency"() -> (w959:dbl)
    n380 = local read "BW/2"() -> (w964:dbl)
    n381 = local read "Rx IQ Rate"() -> (w967:dbl)
    n382 = Subtract(x=w959, y=w964) -> (x-y=w958:dbl)
    n383 = Add(x=w959, y=w964) -> (x+y=w957:dbl)
    n384 = Complex To Polar(r * e^(i*theta)=w944) -> (theta=w971:dbl[])  [unwired: 1 out]
    n385 = call-poly <vilib>:"Butterworth Filter.vi"("init/cont (init:F)"=TRUE, "order"=2, "filter type"=Filter_Passband_Type."Bandpass", "low cutoff freq: fl"=w958, "high cutoff freq: fh"=w957, "sampling freq: fs"=w967, "X"=w979) -> ("Filtered X"=w962:cdb[])  [unwired: 1 in, 1 out]
    n386 = Complex To Polar(r * e^(i*theta)=w962) -> (r=w965:dbl[], theta=w972:dbl[])
    n387 = Subtract(x=w972, y=w971) -> (x-y=w969:dbl[])
    n388 = call <vilib>:"Unwrap Phase.vi"("phase unit"=1 ("y"), "Phase"=w969) -> ("Unwrapped Phase"=w974:dbl[])  [unwired: 8 in, 1 out]
    n389 = local read "DownSamplingRatio"() -> (w978:i32)
    n390 = local read "Waveform Size"() -> (w968:dbl)
    n391 = Divide(x=w968, y=w978) -> (x/y=w975:dbl)
    n392 = Reshape Array(w965, w975, w978) -> (w973:dbl[][])
    n393 = Reshape Array(w974, w975, w978) -> (w976:dbl[][])
    n394 = for {
      tunnel: w973 -> [w989] mode=indexing
      tunnel: [w988] -> w966 mode=indexing
      tunnel: w976 -> [w987] mode=indexing
      tunnel: [w986] -> w977 mode=indexing
      n395 = Add Array Elements(numeric array=w989) -> (sum=w988:dbl)
      n396 = Add Array Elements(numeric array=w987) -> (sum=w986:dbl)
    }
    n397 = Divide(x=w966, y=w978) -> (x/y=w949:dbl[])
    n398 = Divide(x=w977, y=w978) -> (x/y=w948:dbl[])
    n399 = Build Array(w949, w948) -> (w943:dbl[][])
    "appended array" <- w943
    n400 = Array Size(array=w943) -> (size(s)=→"size(s)":i32[])
    n401 = case shown="False" "FlushSDR2" {
      tunnel: w950 -> [w981 w984]
      tunnel: w943 -> [_ w985]
      tunnel: [w980 w982] -> w945
      frame True {
        n402 = Flush Queue(queue=w981) -> (queue out=w980:refnum<queue>)  [unwired: 1 in, 2 out]
      }
      frame False {
        n403 = Get Queue Status(queue=w984) -> (# elements in queue=→"#queue 2":i32)  [unwired: 2 in, 7 out]
        n404 = Enqueue Element(queue=w984, element=w985) -> (queue out=w982:refnum<queue>)  [unwired: 2 in, 2 out]
      }
    }
    "String 2" <- "Reading Rx2data"
  }
  n405 = while {
    shift-right: [w997] -> _
    shift-left: T4."Default" -> [w998]
    stop <- FALSE stop-if-true
    n406 = case shown="4" w998 {
      tunnel: ["Routine" w1015 w1038 w1123 w1148 w1185 w1272 w1360 w1446 w1515 w1584 w1653] -> w997
      tunnel: [0 1 2 3 4 5 6 7 8 9 10 11] -> w996
      tunnel: [w1002 w1013 w1032 w1117 w1142 w1176 w1263 w1349 w1437 w1506 w1575 w1644] -> w994
      tunnel: [w1005 w1020 w1028 "Relaxation phase.." "Perform the online attention test." w1174 w1262 w1350 w1436 w1505 w1574 w1643] -> w995
      tunnel: [w1003 w1021 w1033 w1120 w1145 w1181 w1268 w1356 w1442 w1511 w1580 w1649] -> w993
      tunnel: [w1002 w1013 w1029 w1117 w1142 w1175 w1261 w1351 w1435 w1504 w1573 w1642] -> w992
      tunnel: ["" "" w1026 "" "" w1173 w1260 w1348 w1434 w1503 w1572 w1641] -> w990
      frame 0, Default {
        w1005 = "Wait for instructions."  # Default
        w1002 = 0.0
        # "Waiting - intermediate state"
        n407 = Seconds To Date/Time(time stamp (now)=0.0) -> (date time rec=w1003:T2)  [unwired: 1 in]
        "Output" <- 0 ("Output")
        "Buffer" <- FALSE
        "Flush" <- FALSE ("Flush")
        "Save" <- FALSE ("Save")
      }
      frame 1 {
        w1013 = 0.0
        w1020 = "This is Test run. \nPress STOP TEST to exit and return to default."  # Default
        # "Test"
        n408 = Seconds To Date/Time(time stamp (now)=0.0) -> (date time rec=w1021:T2)  [unwired: 1 in]
        n409 = local write "Output"(1) -> ()
        n410 = local write "Buffer"(FALSE ("Buffer")) -> ()
        n411 = local write "Flush"(FALSE ("Flush")) -> ()
        n412 = local write "Save"(FALSE ("Save")) -> ()
        n413 = case shown="True" "Stop Test" {
          tunnel: [T10."Test" w1025] -> w1015
          frame False {
          }
          frame True {
            w1025 = T11."Default"
            n414 = local write "Routine"(w1025) -> ()
          }
        }
      }
      frame 2 {
        w1035 = 380.0  # Routine Time
        # "Routine 1"
        n415 = property on="Total Routine Time" class="Slide (strict)"("Scale.Maximum"=w1035) -> ()  [unwired: 2 in, 2 out]
        n416 = call "Elapsed Time5"("Time Target (s)"=w1035, "Auto Reset"=FALSE) -> ("Get Start Time (s)"=w1034:dbl, "Elapsed Time (s)"=w1032:dbl, "Time has Elapsed"=w1036:bool)  [unwired: 10 in, 5 out]
        "#1" <- w1036
        n417 = Seconds To Date/Time(time stamp (now)=w1034) -> (date time rec=w1033:T2)  [unwired: 1 in]
        n418 = Not(x=w1036) -> (.not. x?=w1039:bool)
        n419 = script code="t = [0,120,124,130,134,140,144,150,154,160,164,170,174,...\n       180,180.75,181.5,182.25,183,183.75,184.5,185.25,186,186.75,187.5,188.25,189,189.75,190.5,191.25,192,...\n       192.75,193.5,194.25,195,195.75,196.5,197.25,198,198.75,199.5,200.25,201,201.75,202.5,203.25,204,204.75,205.5,...\n       206.25,207,207.75,208.5,209.25,210,...\n        240,260,280,300,...\n        320,330,333,337,347,350,354,364,367,371,380];\n\nevent = [0,1,2,1,2,1,2,1,2,1,2,1,2,...\n               3,4,3,4,3,4,3,4,3,4,3,4,3,4,3,4,3,4,3,4,3,4,3,4,3,4,3,4,3,4,3,4,3,4,3,4,3,4,3,4,0,...\n               7,0,7,0,...\n               0,12,13,0,12,13,0,12,13,0,14];\n\nfor i = 2:length(t)\n    if ((x>=t(i-1)) &&  (x<t(i)))\n        y = event(i-1);\n        yNext = event(i);\n        dt = t(i) - t(i-1);\n        break;\n    end\nend"("x"=w1032) -> ("y"=w1027:dbl, "dt"=w1030:dbl, "yNext"=w1031:dbl)  [unwired: 1 in, 1 out]
        n420 = case shown="False" w1039 {
          tunnel: [w1098 w1110] -> w1038
          frame False {
            n421 = flat-sequence {
              tunnel: [w1106] -> w1098
              frame #0 {
                n422 = local write "Buffer"(FALSE ("Buffer")) -> ()
                n423 = local write "Play/Stop"(FALSE ("Play/Stop")) -> ()
              }
              frame #1 {
                n424 = local write "Output"(0 ("Output")) -> ()
                n425 = local write "Save"(TRUE ("Save")) -> ()
              }
              frame #2 {
                n426 = Wait (ms)(milliseconds to wait=u32 500) -> ()  [unwired: 1 out]
              }
              frame #3 {
                n427 = local write "Flush"(TRUE ("Flush")) -> ()
              }
              frame #4 {
                w1105 = u16 0 items=["No sound", "Demo deep breathing", "Demo fast shallow breathing", "Demo slow shallow breathing", "Demo breath hold", "Demo cough/ laugh", "Demo abdomen movement", "Calibration", "Routine 1", "Routine 3", "Routine 4/5/7", "Calm music"] ("Play sound")
                w1106 = u16 0 items=["Default"] ("Protocol")
                n428 = local write "Flush"(FALSE ("Flush")) -> ()
                n429 = local write "Save"(FALSE ("Save")) -> ()
                n430 = local write "Play sound"(w1105) -> ()
                n431 = local write "Routine"(w1106) -> ()
              }
            }
          }
          frame True {
            w1109 = u16 8 items=["No sound", "Demo normal breathing", "Demo deep breathing", "Demo fast shallow breathing", "Demo breath hold", "Demo cough", "Demo abdomen movement", "Calibration", "Routine 1", "(2a)Calm music", "(2b)Stress test", "Routine 3/4", "Routine 5", ""] ("Play sound")
            n432 = local write "Play sound"(w1109) -> ()
            n433 = flat-sequence {
              tunnel: [T4."Routine 1"] -> w1110
              frame #0 {
                n434 = local write "Output"(1 ("Open")) -> ()
                n435 = local write "Play/Stop"(TRUE ("Play/Stop")) -> ()
              }
              frame #1 {
                n436 = local write "Buffer"(TRUE ("Buffer")) -> ()
              }
              frame #2 {
              }
            }
          }
        }
        n437 = case shown="0, Default" w1027 {
          tunnel: ["\nPerform normal breathing. " "Inhale a slow deep breath." "\nExhale slowly." "Quick inhale.\n\n\n\nIf you cannot sustain for long, resume normal breathing." "\nQuick exhale.\n\n\nIf you cannot sustain for long, resume normal breathing." "Slow shallow inhale.\n\n\n\nIf you cannot sustain for long, resume normal breathing." "\nSlow exhale.\n\n\nIf you cannot sustain for long, resume normal breathing." "Exhale the current breath  and HOLD.\n\n\nIf you cannot sustain for long, resume normal breathing." "Perform voluntary coughing \n" "Perform voluntary laugh\n\n" "Read aloud the following text in between the lines:\n-----------------------------------------------------------------------\nFour score and seven years ago our fathers brought forth on this continent, a new nation, conceived in Liberty, and dedicated to the proposition that all men are created equal… That this nation, under God, shall have a new birth of freedom-and that government of the people, by the people, for the people, shall not perish from the earth.\n\n-----------------------------------------------------------------------\nWhen finished, take a deep breath and open mouth say \"Ah\" (like doctor checking your throat).\nPerform normal breathing until next instruction." "Exhale current breath and HOLD. Push abdomen inwards." "Relax abdomen back to normal and keep holding breath."] -> w1028
          frame 0, Default {
          }
          frame 1 {
          }
          frame 2 {
          }
          frame 3 {
          }
          frame 4 {
          }
          frame 5 {
          }
          frame 6 {
          }
          frame 7 {
          }
          frame 8 {
          }
          frame 9 {
          }
          frame 10 {
          }
          frame 12 {
          }
          frame 13 {
          }
        }
        n438 = case shown="0, Default" w1031 {
          tunnel: ["\nPerform normal breathing." "Inhale a slow deep breath." "\nExhale slowly." "Quick inhale.\n\n\n\nIf you cannot sustain for long, resume normal breathing." "\nQuick exhale.\n\n\nIf you cannot sustain for long, resume normal breathing." "Slow shallow inhale.\n\n\n\nIf you cannot sustain for long, resume normal breathing." "\nSlow exhale.\n\n\nIf you cannot sustain for long, resume normal breathing." "Exhale the current breath  and HOLD.\n\n\nIf you cannot sustain for long, resume normal breathing." "Perform voluntary coughing \n" "Perform voluntary laugh\n\n" "Read aloud the following text in between the lines:\n-----------------------------------------------------------------------\nFour score and seven years ago our fathers brought forth on this continent, a new nation, conceived in Liberty, and dedicated to the proposition that all men are created equal… That this nation, under God, shall have a new birth of freedom-and that government of the people, by the people, for the people, shall not perish from the earth.\n\n-----------------------------------------------------------------------\nWhen finished, take a deep breath and open mouth say \"Ah\" (like doctor checking your throat).\nPerform normal breathing until next instruction." "Exhale current breath and HOLD. Push abdomen inwards." "Relax abdomen back to normal and keep holding breath." "Wait for next routine!"] -> w1026
          frame 0, Default {
          }
          frame 1 {
          }
          frame 2 {
          }
          frame 3 {
          }
          frame 4 {
          }
          frame 5 {
          }
          frame 6 {
          }
          frame 7 {
          }
          frame 8 {
          }
          frame 9 {
          }
          frame 10 {
          }
          frame 12 {
          }
          frame 13 {
          }
          frame 14 {
          }
        }
        n439 = case shown="2" w1027 {
          tunnel: w1030 -> [w1043 w1045 w1047 w1049 w1051 w1053 w1055 w1057 w1059 w1061 w1063 w1065 w1067 w1070]
          tunnel: [w1042 w1044 w1046 w1048 w1050 w1052 w1054 w1056 w1058 w1060 w1062 w1064 w1066 w1069] -> w1029
          frame 1 {
            n440 = property on="Current Task time" class="Slide (strict)"("Scale.Maximum"=w1043) -> ()  [unwired: 2 in, 2 out]
            n441 = call "Elapsed Time11"("Time Target (s)"=w1043) -> ("Elapsed Time (s)"=w1042:dbl)  [unwired: 11 in, 7 out]
            n442 = property on="Current Task time" class="Slide (strict)"("Scale.Minimum"=0.0 ("Scale.Range:Minimum")) -> ()  [unwired: 2 in, 2 out]
          }
          frame 2 {
            n443 = property on="Current Task time" class="Slide (strict)"("Scale.Maximum"=w1045) -> ()  [unwired: 2 in, 2 out]
            n444 = call "Elapsed Time12"("Time Target (s)"=w1045) -> ("Elapsed Time (s)"=w1044:dbl)  [unwired: 11 in, 7 out]
          }
          frame 3 {
            n445 = property on="Current Task time" class="Slide (strict)"("Scale.Maximum"=w1047) -> ()  [unwired: 2 in, 2 out]
            n446 = call "Elapsed Time13"("Time Target (s)"=w1047) -> ("Elapsed Time (s)"=w1046:dbl)  [unwired: 11 in, 7 out]
          }
          frame 4 {
            n447 = property on="Current Task time" class="Slide (strict)"("Scale.Maximum"=w1049) -> ()  [unwired: 2 in, 2 out]
            n448 = call "Elapsed Time14"("Time Target (s)"=w1049) -> ("Elapsed Time (s)"=w1048:dbl)  [unwired: 11 in, 7 out]
          }
          frame 5 {
            n449 = property on="Current Task time" class="Slide (strict)"("Scale.Maximum"=w1051) -> ()  [unwired: 2 in, 2 out]
            n450 = call "Elapsed Time15"("Time Target (s)"=w1051) -> ("Elapsed Time (s)"=w1050:dbl)  [unwired: 11 in, 7 out]
          }
          frame 6 {
            n451 = property on="Current Task time" class="Slide (strict)"("Scale.Maximum"=w1053) -> ()  [unwired: 2 in, 2 out]
            n452 = call "Elapsed Time16"("Time Target (s)"=w1053) -> ("Elapsed Time (s)"=w1052:dbl)  [unwired: 11 in, 7 out]
          }
          frame 7 {
            n453 = property on="Current Task time" class="Slide (strict)"("Scale.Maximum"=w1055) -> ()  [unwired: 2 in, 2 out]
            n454 = call "Elapsed Time17"("Time Target (s)"=w1055) -> ("Elapsed Time (s)"=w1054:dbl)  [unwired: 11 in, 7 out]
          }
          frame 8 {
            n455 = property on="Current Task time" class="Slide (strict)"("Scale.Maximum"=w1057) -> ()  [unwired: 2 in, 2 out]
            n456 = call "Elapsed Time18"("Time Target (s)"=w1057) -> ("Elapsed Time (s)"=w1056:dbl)  [unwired: 11 in, 7 out]
          }
          frame 9 {
            n457 = property on="Current Task time" class="Slide (strict)"("Scale.Maximum"=w1059) -> ()  [unwired: 2 in, 2 out]
            n458 = call "Elapsed Time19"("Time Target (s)"=w1059) -> ("Elapsed Time (s)"=w1058:dbl)  [unwired: 11 in, 7 out]
          }
          frame 10 {
            n459 = property on="Current Task time" class="Slide (strict)"("Scale.Maximum"=w1061) -> ()  [unwired: 2 in, 2 out]
            n460 = call "Elapsed Time20"("Time Target (s)"=w1061) -> ("Elapsed Time (s)"=w1060:dbl)  [unwired: 11 in, 7 out]
          }
          frame 11 {
            n461 = property on="Current Task time" class="Slide (strict)"("Scale.Maximum"=w1063) -> ()  [unwired: 2 in, 2 out]
            n462 = call "Elapsed Time21"("Time Target (s)"=w1063) -> ("Elapsed Time (s)"=w1062:dbl)  [unwired: 11 in, 7 out]
          }
          frame 12 {
            n463 = property on="Current Task time" class="Slide (strict)"("Scale.Maximum"=w1065) -> ()  [unwired: 2 in, 2 out]
            n464 = call "Elapsed Time22"("Time Target (s)"=w1065) -> ("Elapsed Time (s)"=w1064:dbl)  [unwired: 11 in, 7 out]
          }
          frame 13 {
            n465 = property on="Current Task time" class="Slide (strict)"("Scale.Maximum"=w1067) -> ()  [unwired: 2 in, 2 out]
            n466 = call "Elapsed Time23"("Time Target (s)"=w1067) -> ("Elapsed Time (s)"=w1066:dbl)  [unwired: 11 in, 7 out]
          }
          frame 0, Default {
            n467 = property on="Current Task time" class="Slide (strict)"("Scale.Maximum"=w1070) -> ()  [unwired: 2 in, 2 out]
            n468 = call "Elapsed Time24"("Time Target (s)"=w1070) -> ("Elapsed Time (s)"=w1069:dbl)  [unwired: 11 in, 7 out]
            n469 = property on="Current Task time" class="Slide (strict)"("Scale.Minimum"=0.0 ("Scale.Range:Minimum")) -> ()  [unwired: 2 in, 2 out]
          }
        }
      }
      frame 3 {
        w1116 = 300.0  # Routine Time
        # "Routine 2a: Attention test - relaxing music"
        n470 = property on="Total Routine Time" class="Slide (strict)"("Scale.Maximum"=w1116) -> ()  [unwired: 2 in, 2 out]
        n471 = property on="Current Task time" class="Slide (strict)"("Scale.Maximum"=w1116) -> ()  [unwired: 2 in, 2 out]
        n472 = call "Elapsed Time7"("Time Target (s)"=w1116, "Auto Reset"=FALSE ("Timer Reset")) -> ("Get Start Time (s)"=w1119:dbl, "Elapsed Time (s)"=w1117:dbl, "Time has Elapsed"=w1121:bool)  [unwired: 10 in, 5 out]
        "#2a" <- w1121
        n473 = Seconds To Date/Time(time stamp (now)=w1119) -> (date time rec=w1120:T2)  [unwired: 1 in]
        n474 = Not(x=w1121) -> (.not. x?=w1124:bool)
        n475 = case shown="False" w1124 {
          tunnel: [w1126 w1135] -> w1123
          frame False {
            n476 = flat-sequence {
              tunnel: [w1132] -> w1126
              frame #0 {
                n477 = local write "Buffer"(FALSE ("Buffer")) -> ()
              }
              frame #1 {
                n478 = local write "Output"(0 ("Output")) -> ()
                n479 = local write "Save"(TRUE ("Save")) -> ()
              }
              frame #2 {
                n480 = Wait (ms)(milliseconds to wait=u32 500) -> ()  [unwired: 1 out]
              }
              frame #3 {
                n481 = local write "Flush"(TRUE ("Flush")) -> ()
              }
              frame #4 {
                w1132 = enum16{"Default"}."Default"
                n482 = local write "Flush"(FALSE ("Flush")) -> ()
                n483 = local write "Save"(FALSE ("Save")) -> ()
                n484 = local write "Routine"(w1132) -> ()
              }
            }
          }
          frame True {
            n485 = flat-sequence {
              tunnel: [T4."Routine 2a"] -> w1135
              frame #0 {
                n486 = local write "Output"(1 ("Open")) -> ()
                n487 = local write "Play/Stop"(TRUE ("PlayMusic")) -> ()
              }
              frame #1 {
                n488 = local write "Buffer"(TRUE ("Buffer")) -> ()
              }
              frame #2 {
              }
            }
          }
        }
      }
      frame 4 {
        w1141 = 400.0  # Routine Time
        # "Routine 2b: Attention test"
        n489 = property on="Total Routine Time" class="Slide (strict)"("Scale.Maximum"=w1141) -> ()  [unwired: 2 in, 2 out]
        n490 = property on="Current Task time" class="Slide (strict)"("Scale.Maximum"=w1141) -> ()  [unwired: 2 in, 2 out]
        n491 = call "Elapsed Time9"("Time Target (s)"=w1141, "Auto Reset"=FALSE ("Timer Reset")) -> ("Get Start Time (s)"=w1144:dbl, "Elapsed Time (s)"=w1142:dbl, "Time has Elapsed"=w1146:bool)  [unwired: 10 in, 5 out]
        "#2b" <- w1146
        n492 = Seconds To Date/Time(time stamp (now)=w1144) -> (date time rec=w1145:T2)  [unwired: 1 in]
        n493 = Not(x=w1146) -> (.not. x?=w1149:bool)
        n494 = case shown="True" w1149 {
          tunnel: [w1151 w1163] -> w1148
          frame False {
            n495 = flat-sequence {
              tunnel: [w1158] -> w1151
              frame #0 {
                n496 = local write "Buffer"(FALSE ("Buffer")) -> ()
                n497 = local write "Play/Stop"(FALSE ("Play/Stop")) -> ()
              }
              frame #1 {
                n498 = local write "Output"(0 ("Output")) -> ()
                n499 = local write "Save"(TRUE ("Save")) -> ()
              }
              frame #2 {
                n500 = Wait (ms)(milliseconds to wait=u32 500) -> ()  [unwired: 1 out]
              }
              frame #3 {
                n501 = local write "Flush"(TRUE ("Flush")) -> ()
              }
              frame #4 {
                w1158 = enum16{"Default"}."Default"
                n502 = local write "Flush"(FALSE ("Flush")) -> ()
                n503 = local write "Save"(FALSE ("Save")) -> ()
                n504 = local write "Routine"(w1158) -> ()
              }
            }
          }
          frame True {
            w1161 = u16 10 items=["No sound", "Demo normal breathing", "Demo deep breathing", "Demo fast shallow breathing", "Demo breath hold", "Demo cough", "Demo abdomen movement", "Calibration", "Routine 1", "(2a)Calm music", "(2b)Stress test", "Routine 3/4", "Routine 5", ""] ("Play sound")
            n505 = local write "Play sound"(w1161) -> ()
            n506 = flat-sequence {
              tunnel: "OpenHTML" -> [w1165]
              tunnel: [T4."Routine 2b"] -> w1163
              frame #0 {
                n507 = And(x=TRUE, y=w1165) -> (x .and. y?=w1167:bool)
                n508 = case shown="True" w1167 {
                  frame False {
                  }
                  frame True {
                    n509 = local write "OpenHTML"(FALSE ("OpenHTML")) -> ()
                    n510 = call-poly <vilib>:"Open URL in Default Browser.vi"("URL"="\"E:\\NCS\\HumanStudyMarch2019\\StressTest\\mackworth\\vigilanceTest.html\"") -> ()  [unwired: 5 in, 2 out]
                  }
                }
                n511 = local write "Play/Stop"(TRUE ("Play/Stop")) -> ()
                n512 = local write "Output"(1 ("Open")) -> ()
              }
              frame #1 {
                n513 = local write "Buffer"(TRUE ("Buffer")) -> ()
              }
              frame #2 {
              }
            }
          }
        }
      }
      frame 5 {
        w1182 = 320.0  # Routine Time
        # "Routine 3: Lying on bed in supine"
        n514 = property on="Total Routine Time" class="Slide (strict)"("Scale.Maximum"=w1182) -> ()  [unwired: 2 in, 2 out]
        n515 = call "Elapsed Time"("Time Target (s)"=w1182, "Auto Reset"=FALSE ("Timer Reset")) -> ("Get Start Time (s)"=w1180:dbl, "Elapsed Time (s)"=w1176:dbl, "Time has Elapsed"=w1183:bool)  [unwired: 10 in, 5 out]
        "#3" <- w1183
        n516 = Seconds To Date/Time(time stamp (now)=w1180) -> (date time rec=w1181:T2)  [unwired: 1 in]
        n517 = Not(x=w1183) -> (.not. x?=w1186:bool)
        n518 = script code="t = [0,120,124,130,134,140,144,150,154,160,164,170,174,...\n       180,180.75,181.5,182.25,183,183.75,184.5,185.25,186,186.75,187.5,188.25,189,189.75,190.5,191.25,192,...\n       192.75,193.5,194.25,195,195.75,196.5,197.25,198,198.75,199.5,200.25,201,201.75,202.5,203.25,204,204.75,205.5,...\n       206.25,207,207.75,208.5,209.25,210,...\n        240,260,280,300,...\n        320];\n\nevent = [0,1,2,1,2,1,2,1,2,1,2,1,2,...\n               3,4,3,4,3,4,3,4,3,4,3,4,3,4,3,4,3,4,3,4,3,4,3,4,3,4,3,4,3,4,3,4,3,4,3,4,3,4,3,4,0,...\n               7,0,7,0,...\n               14];\n\nfor i = 2:length(t)\n    if ((x>=t(i-1)) &&  (x<t(i)))\n        y = event(i-1);\n        yNext = event(i);\n        dt = t(i) - t(i-1);\n        break;\n    end\nend"("x"=w1176) -> ("y"=w1177:dbl, "dt"=w1178:dbl, "yNext"=w1179:dbl)  [unwired: 1 in, 1 out]
        n519 = case shown="True" w1186 {
          tunnel: [w1243 w1255] -> w1185
          frame False {
            n520 = flat-sequence {
              tunnel: [w1251] -> w1243
              frame #0 {
                n521 = local write "Buffer"(FALSE ("Buffer")) -> ()
                n522 = local write "Play/Stop"(FALSE ("PlayInstr")) -> ()
              }
              frame #1 {
                n523 = local write "Output"(0 ("Output")) -> ()
                n524 = local write "Save"(TRUE ("Save")) -> ()
              }
              frame #2 {
                n525 = Wait (ms)(milliseconds to wait=u32 500) -> ()  [unwired: 1 out]
              }
              frame #3 {
                n526 = local write "Flush"(TRUE ("Flush")) -> ()
              }
              frame #4 {
                w1250 = u16 0 items=["No sound", "Demo deep breathing", "Demo fast shallow breathing", "Demo slow shallow breathing", "Demo breath hold", "Demo cough/ laugh", "Demo abdomen movement", "Calibration", "Routine 1", "Routine 3", "Routine 4/5/7", "Calm music"] ("Play sound")
                w1251 = enum16{"Default"}."Default"
                n527 = local write "Flush"(FALSE ("Flush")) -> ()
                n528 = local write "Save"(FALSE ("Save")) -> ()
                n529 = local write "Play sound"(w1250) -> ()
                n530 = local write "Routine"(w1251) -> ()
              }
            }
          }
          frame True {
            w1254 = u16 11 items=["No sound", "Demo normal breathing", "Demo deep breathing", "Demo fast shallow breathing", "Demo breath hold", "Demo cough", "Demo abdomen movement", "Calibration", "Routine 1", "(2a)Calm music", "(2b)Stress test", "Routine 3/4", "Routine 5", ""] ("Play sound")
            n531 = local write "Play sound"(w1254) -> ()
            n532 = flat-sequence {
              tunnel: [T4."Routine 3"] -> w1255
              frame #0 {
                n533 = local write "Output"(1 ("Open")) -> ()
                n534 = local write "Play/Stop"(TRUE ("PlayInstruction")) -> ()
              }
              frame #1 {
                n535 = local write "Buffer"(TRUE ("Buffer")) -> ()
              }
              frame #2 {
              }
            }
          }
        }
        n536 = case shown="0, Default" w1177 {
          tunnel: ["\nPerform normal breathing." "Inhale a slow deep breath." "\nExhale slowly." "Quick inhale.\n\n\n\nIf you cannot sustain for long, resume normal breathing." "\nQuick exhale.\n\n\nIf you cannot sustain for long, resume normal breathing." "Slow shallow inhale.\n\n\n\nIf you cannot sustain for long, resume normal breathing." "\nSlow exhale.\n\n\nIf you cannot sustain for long, resume normal breathing." "Exhale the current breath  and HOLD.\n\n\nIf you cannot sustain for long, resume normal breathing." "Perform voluntary coughing \n" "Perform voluntary laugh\n\n" "Read aloud the following text in between the lines:\n-----------------------------------------------------------------------\nFour score and seven years ago our fathers brought forth on this continent, a new nation, conceived in Liberty, and dedicated to the proposition that all men are created equal… That this nation, under God, shall have a new birth of freedom-and that government of the people, by the people, for the people, shall not perish from the earth.\n\n-----------------------------------------------------------------------\nWhen finished, take a deep breath and open mouth say \"Ah\" (like doctor checking your throat).\nPerform normal breathing until next instruction." "Exhale current breath and HOLD. Push abdomen inwards." "Relax abdomen back to normal and keep holding breath."] -> w1174
          frame 0, Default {
          }
          frame 1 {
          }
          frame 2 {
          }
          frame 3 {
          }
          frame 4 {
          }
          frame 5 {
          }
          frame 6 {
          }
          frame 7 {
          }
          frame 8 {
          }
          frame 9 {
          }
          frame 10 {
          }
          frame 12 {
          }
          frame 13 {
          }
        }
        n537 = case shown="14" w1179 {
          tunnel: ["\nPerform normal breathing." "Inhale a slow deep breath." "\nExhale slowly." "Quick inhale.\n\n\n\nIf you cannot sustain for long, resume normal breathing." "\nQuick exhale.\n\n\nIf you cannot sustain for long, resume normal breathing." "Slow shallow inhale.\n\n\n\nIf you cannot sustain for long, resume normal breathing." "\nSlow exhale.\n\n\nIf you cannot sustain for long, resume normal breathing." "Exhale the current breath  and HOLD.\n\n\nIf you cannot sustain for long, resume normal breathing." "Perform voluntary coughing \n" "Perform voluntary laugh\n\n" "Read aloud the following text in between the lines:\n-----------------------------------------------------------------------\nFour score and seven years ago our fathers brought forth on this continent, a new nation, conceived in Liberty, and dedicated to the proposition that all men are created equal… That this nation, under God, shall have a new birth of freedom-and that government of the people, by the people, for the people, shall not perish from the earth.\n\n-----------------------------------------------------------------------\nWhen finished, take a deep breath and open mouth say \"Ah\" (like doctor checking your throat).\nPerform normal breathing until next instruction." "Exhale current breath and HOLD. Push abdomen inwards." "Relax abdomen back to normal and keep holding breath." "Wait for next routine!"] -> w1173
          frame 0, Default {
          }
          frame 1 {
          }
          frame 2 {
          }
          frame 3 {
          }
          frame 4 {
          }
          frame 5 {
          }
          frame 6 {
          }
          frame 7 {
          }
          frame 8 {
          }
          frame 9 {
          }
          frame 10 {
          }
          frame 12 {
          }
          frame 13 {
          }
          frame 14 {
          }
        }
        n538 = case shown="5" w1177 {
          tunnel: w1178 -> [w1189 w1191 w1193 w1195 w1197 w1199 w1201 w1203 w1205 w1207 w1209 w1211 w1213 w1215]
          tunnel: [w1188 w1190 w1192 w1194 w1196 w1198 w1200 w1202 w1204 w1206 w1208 w1210 w1212 w1214] -> w1175
          frame 1 {
            n539 = property on="Current Task time" class="Slide (strict)"("Scale.Maximum"=w1189) -> ()  [unwired: 2 in, 2 out]
            n540 = call "Elapsed Time34"("Time Target (s)"=w1189) -> ("Elapsed Time (s)"=w1188:dbl)  [unwired: 11 in, 7 out]
          }
          frame 2 {
            n541 = property on="Current Task time" class="Slide (strict)"("Scale.Maximum"=w1191) -> ()  [unwired: 2 in, 2 out]
            n542 = call "Elapsed Time35"("Time Target (s)"=w1191) -> ("Elapsed Time (s)"=w1190:dbl)  [unwired: 11 in, 7 out]
          }
          frame 3 {
            n543 = property on="Current Task time" class="Slide (strict)"("Scale.Maximum"=w1193) -> ()  [unwired: 2 in, 2 out]
            n544 = call "Elapsed Time36"("Time Target (s)"=w1193) -> ("Elapsed Time (s)"=w1192:dbl)  [unwired: 11 in, 7 out]
          }
          frame 4 {
            n545 = property on="Current Task time" class="Slide (strict)"("Scale.Maximum"=w1195) -> ()  [unwired: 2 in, 2 out]
            n546 = call "Elapsed Time37"("Time Target (s)"=w1195) -> ("Elapsed Time (s)"=w1194:dbl)  [unwired: 11 in, 7 out]
          }
          frame 5 {
            n547 = property on="Current Task time" class="Slide (strict)"("Scale.Maximum"=w1197) -> ()  [unwired: 2 in, 2 out]
            n548 = call "Elapsed Time38"("Time Target (s)"=w1197) -> ("Elapsed Time (s)"=w1196:dbl)  [unwired: 11 in, 7 out]
          }
          frame 6 {
            n549 = property on="Current Task time" class="Slide (strict)"("Scale.Maximum"=w1199) -> ()  [unwired: 2 in, 2 out]
            n550 = call "Elapsed Time39"("Time Target (s)"=w1199) -> ("Elapsed Time (s)"=w1198:dbl)  [unwired: 11 in, 7 out]
          }
          frame 7 {
            n551 = property on="Current Task time" class="Slide (strict)"("Scale.Maximum"=w1201) -> ()  [unwired: 2 in, 2 out]
            n552 = call "Elapsed Time40"("Time Target (s)"=w1201) -> ("Elapsed Time (s)"=w1200:dbl)  [unwired: 11 in, 7 out]
          }
          frame 8 {
            n553 = property on="Current Task time" class="Slide (strict)"("Scale.Maximum"=w1203) -> ()  [unwired: 2 in, 2 out]
            n554 = call "Elapsed Time41"("Time Target (s)"=w1203) -> ("Elapsed Time (s)"=w1202:dbl)  [unwired: 11 in, 7 out]
          }
          frame 9 {
            n555 = property on="Current Task time" class="Slide (strict)"("Scale.Maximum"=w1205) -> ()  [unwired: 2 in, 2 out]
            n556 = call "Elapsed Time42"("Time Target (s)"=w1205) -> ("Elapsed Time (s)"=w1204:dbl)  [unwired: 11 in, 7 out]
          }
          frame 10 {
            n557 = property on="Current Task time" class="Slide (strict)"("Scale.Maximum"=w1207) -> ()  [unwired: 2 in, 2 out]
            n558 = call "Elapsed Time43"("Time Target (s)"=w1207) -> ("Elapsed Time (s)"=w1206:dbl)  [unwired: 11 in, 7 out]
          }
          frame 11 {
            n559 = property on="Current Task time" class="Slide (strict)"("Scale.Maximum"=w1209) -> ()  [unwired: 2 in, 2 out]
            n560 = call "Elapsed Time44"("Time Target (s)"=w1209) -> ("Elapsed Time (s)"=w1208:dbl)  [unwired: 11 in, 7 out]
          }
          frame 12 {
            n561 = property on="Current Task time" class="Slide (strict)"("Scale.Maximum"=w1211) -> ()  [unwired: 2 in, 2 out]
            n562 = call "Elapsed Time45"("Time Target (s)"=w1211) -> ("Elapsed Time (s)"=w1210:dbl)  [unwired: 11 in, 7 out]
          }
          frame 13 {
            n563 = property on="Current Task time" class="Slide (strict)"("Scale.Maximum"=w1213) -> ()  [unwired: 2 in, 2 out]
            n564 = call "Elapsed Time122"("Time Target (s)"=w1213) -> ("Elapsed Time (s)"=w1212:dbl)  [unwired: 11 in, 7 out]
          }
          frame 0, Default {
            n565 = property on="Current Task time" class="Slide (strict)"("Scale.Maximum"=w1215) -> ()  [unwired: 2 in, 2 out]
            n566 = call "Elapsed Time123"("Time Target (s)"=w1215) -> ("Elapsed Time (s)"=w1214:dbl)  [unwired: 11 in, 7 out]
          }
        }
      }
      frame 6 {
        w1269 = 320.0  # Routine Time
        # "Routine 4: Lying on bed turned"
        n567 = property on="Total Routine Time" class="Slide (strict)"("Scale.Maximum"=w1269) -> ()  [unwired: 2 in, 2 out]
        n568 = call "Elapsed Time2"("Time Target (s)"=w1269, "Auto Reset"=FALSE ("Timer Reset")) -> ("Get Start Time (s)"=w1267:dbl, "Elapsed Time (s)"=w1263:dbl, "Time has Elapsed"=w1270:bool)  [unwired: 10 in, 5 out]
        "#4" <- w1270
        n569 = Seconds To Date/Time(time stamp (now)=w1267) -> (date time rec=w1268:T2)  [unwired: 1 in]
        n570 = Not(x=w1270) -> (.not. x?=w1273:bool)
        n571 = script code="t = [0,120,124,130,134,140,144,150,154,160,164,170,174,...\n       180,180.75,181.5,182.25,183,183.75,184.5,185.25,186,186.75,187.5,188.25,189,189.75,190.5,191.25,192,...\n       192.75,193.5,194.25,195,195.75,196.5,197.25,198,198.75,199.5,200.25,201,201.75,202.5,203.25,204,204.75,205.5,...\n       206.25,207,207.75,208.5,209.25,210,...\n        240,260,280,300,...\n        320];\n\nevent = [0,1,2,1,2,1,2,1,2,1,2,1,2,...\n               3,4,3,4,3,4,3,4,3,4,3,4,3,4,3,4,3,4,3,4,3,4,3,4,3,4,3,4,3,4,3,4,3,4,3,4,3,4,3,4,0,...\n               7,0,7,0,...\n               14];\n\nfor i = 2:length(t)\n    if ((x>=t(i-1)) &&  (x<t(i)))\n        y = event(i-1);\n        yNext = event(i);\n        dt = t(i) - t(i-1);\n        break;\n    end\nend"("x"=w1263) -> ("y"=w1264:dbl, "dt"=w1265:dbl, "yNext"=w1266:dbl)  [unwired: 1 in, 1 out]
        n572 = case shown="True" w1273 {
          tunnel: [w1330 w1342] -> w1272
          frame False {
            n573 = flat-sequence {
              tunnel: [w1338] -> w1330
              frame #0 {
                n574 = local write "Buffer"(FALSE ("Buffer")) -> ()
                n575 = local write "Play/Stop"(FALSE ("PlayInstruction")) -> ()
              }
              frame #1 {
                n576 = local write "Output"(0 ("Output")) -> ()
                n577 = local write "Save"(TRUE ("Save")) -> ()
              }
              frame #2 {
                n578 = Wait (ms)(milliseconds to wait=u32 500) -> ()  [unwired: 1 out]
              }
              frame #3 {
                n579 = local write "Flush"(TRUE ("Flush")) -> ()
              }
              frame #4 {
                w1337 = u16 0 items=["No sound", "Demo deep breathing", "Demo fast shallow breathing", "Demo slow shallow breathing", "Demo breath hold", "Demo cough/ laugh", "Demo abdomen movement", "Calibration", "Routine 1", "Routine 3", "Routine 4/5/7", "Calm music"] ("Play sound")
                w1338 = enum16{"Default"}."Default"
                n580 = local write "Flush"(FALSE ("Flush")) -> ()
                n581 = local write "Save"(FALSE ("Save")) -> ()
                n582 = local write "Play sound"(w1337) -> ()
                n583 = local write "Routine"(w1338) -> ()
              }
            }
          }
          frame True {
            w1341 = u16 11 items=["No sound", "Demo normal breathing", "Demo deep breathing", "Demo fast shallow breathing", "Demo breath hold", "Demo cough", "Demo abdomen movement", "Calibration", "Routine 1", "(2a)Calm music", "(2b)Stress test", "Routine 3/4", "Routine 5", ""] ("Play sound")
            n584 = local write "Play sound"(w1341) -> ()
            n585 = flat-sequence {
              tunnel: [T4."Routine 4"] -> w1342
              frame #0 {
                n586 = local write "Output"(1 ("Open")) -> ()
                n587 = local write "Play/Stop"(TRUE ("PlayInstruction")) -> ()
              }
              frame #1 {
                n588 = local write "Buffer"(TRUE ("Buffer")) -> ()
              }
              frame #2 {
              }
            }
          }
        }
        n589 = case shown="0, Default" w1264 {
          tunnel: ["\nPerform normal breathing." "Inhale a slow deep breath." "\nExhale slowly." "Quick inhale.\n\n\n\nIf you cannot sustain for long, resume normal breathing." "\nQuick exhale.\n\n\nIf you cannot sustain for long, resume normal breathing." "Slow shallow inhale.\n\n\n\nIf you cannot sustain for long, resume normal breathing." "\nSlow exhale.\n\n\nIf you cannot sustain for long, resume normal breathing." "Exhale the current breath  and HOLD.\n\n\nIf you cannot sustain for long, resume normal breathing." "Perform voluntary coughing \n" "Perform voluntary laugh\n\n" "Read aloud the following text in between the lines:\n-----------------------------------------------------------------------\nFour score and seven years ago our fathers brought forth on this continent, a new nation, conceived in Liberty, and dedicated to the proposition that all men are created equal… That this nation, under God, shall have a new birth of freedom-and that government of the people, by the people, for the people, shall not perish from the earth.\n\n-----------------------------------------------------------------------\nWhen finished, take a deep breath and open mouth say \"Ah\" (like doctor checking your throat).\nPerform normal breathing until next instruction." "Exhale current breath and HOLD. Push abdomen inwards." "Relax abdomen back to normal and keep holding breath."] -> w1262
          frame 0, Default {
          }
          frame 1 {
          }
          frame 2 {
          }
          frame 3 {
          }
          frame 4 {
          }
          frame 5 {
          }
          frame 6 {
          }
          frame 7 {
          }
          frame 8 {
          }
          frame 9 {
          }
          frame 10 {
          }
          frame 12 {
          }
          frame 13 {
          }
        }
        n590 = case shown="14" w1266 {
          tunnel: ["\nPerform normal breathing." "Inhale a slow deep breath." "\nExhale slowly." "Quick inhale.\n\n\n\nIf you cannot sustain for long, resume normal breathing." "\nQuick exhale.\n\n\nIf you cannot sustain for long, resume normal breathing." "Slow shallow inhale.\n\n\n\nIf you cannot sustain for long, resume normal breathing." "\nSlow exhale.\n\n\nIf you cannot sustain for long, resume normal breathing." "Exhale the current breath  and HOLD.\n\n\nIf you cannot sustain for long, resume normal breathing." "Perform voluntary coughing \n" "Perform voluntary laugh\n\n" "Read aloud the following text in between the lines:\n-----------------------------------------------------------------------\nFour score and ...\n-----------------------------------------------------------------------\nWhen finished, take a deep breath and open mouth say \"Ah\" (like doctor checking your throat).\nPerform normal breathing until next instruction." "Exhale current breath and HOLD. Push abdomen inwards." "Relax abdomen back to normal and keep holding breath." "Wait for next routine!"] -> w1260
          frame 0, Default {
          }
          frame 1 {
          }
          frame 2 {
          }
          frame 3 {
          }
          frame 4 {
          }
          frame 5 {
          }
          frame 6 {
          }
          frame 7 {
          }
          frame 8 {
          }
          frame 9 {
          }
          frame 10 {
          }
          frame 12 {
          }
          frame 13 {
          }
          frame 14 {
          }
        }
        n591 = case shown="0, Default" w1264 {
          tunnel: w1265 -> [w1276 w1278 w1280 w1282 w1284 w1286 w1288 w1290 w1292 w1294 w1296 w1298 w1300 w1302]
          tunnel: [w1275 w1277 w1279 w1281 w1283 w1285 w1287 w1289 w1291 w1293 w1295 w1297 w1299 w1301] -> w1261
          frame 1 {
            n592 = property on="Current Task time" class="Slide (strict)"("Scale.Maximum"=w1276) -> ()  [unwired: 2 in, 2 out]
            n593 = call "Elapsed Time46"("Time Target (s)"=w1276) -> ("Elapsed Time (s)"=w1275:dbl)  [unwired: 11 in, 7 out]
          }
          frame 2 {
            n594 = property on="Current Task time" class="Slide (strict)"("Scale.Maximum"=w1278) -> ()  [unwired: 2 in, 2 out]
            n595 = call "Elapsed Time47"("Time Target (s)"=w1278) -> ("Elapsed Time (s)"=w1277:dbl)  [unwired: 11 in, 7 out]
          }
          frame 3 {
            n596 = property on="Current Task time" class="Slide (strict)"("Scale.Maximum"=w1280) -> ()  [unwired: 2 in, 2 out]
            n597 = call "Elapsed Time48"("Time Target (s)"=w1280) -> ("Elapsed Time (s)"=w1279:dbl)  [unwired: 11 in, 7 out]
          }
          frame 4 {
            n598 = property on="Current Task time" class="Slide (strict)"("Scale.Maximum"=w1282) -> ()  [unwired: 2 in, 2 out]
            n599 = call "Elapsed Time49"("Time Target (s)"=w1282) -> ("Elapsed Time (s)"=w1281:dbl)  [unwired: 11 in, 7 out]
          }
          frame 5 {
            n600 = property on="Current Task time" class="Slide (strict)"("Scale.Maximum"=w1284) -> ()  [unwired: 2 in, 2 out]
            n601 = call "Elapsed Time50"("Time Target (s)"=w1284) -> ("Elapsed Time (s)"=w1283:dbl)  [unwired: 11 in, 7 out]
          }
          frame 6 {
            n602 = property on="Current Task time" class="Slide (strict)"("Scale.Maximum"=w1286) -> ()  [unwired: 2 in, 2 out]
            n603 = call "Elapsed Time51"("Time Target (s)"=w1286) -> ("Elapsed Time (s)"=w1285:dbl)  [unwired: 11 in, 7 out]
          }
          frame 7 {
            n604 = property on="Current Task time" class="Slide (strict)"("Scale.Maximum"=w1288) -> ()  [unwired: 2 in, 2 out]
            n605 = call "Elapsed Time52"("Time Target (s)"=w1288) -> ("Elapsed Time (s)"=w1287:dbl)  [unwired: 11 in, 7 out]
          }
          frame 8 {
            n606 = property on="Current Task time" class="Slide (strict)"("Scale.Maximum"=w1290) -> ()  [unwired: 2 in, 2 out]
            n607 = call "Elapsed Time53"("Time Target (s)"=w1290) -> ("Elapsed Time (s)"=w1289:dbl)  [unwired: 11 in, 7 out]
          }
          frame 9 {
            n608 = property on="Current Task time" class="Slide (strict)"("Scale.Maximum"=w1292) -> ()  [unwired: 2 in, 2 out]
            n609 = call "Elapsed Time54"("Time Target (s)"=w1292) -> ("Elapsed Time (s)"=w1291:dbl)  [unwired: 11 in, 7 out]
          }
          frame 10 {
            n610 = property on="Current Task time" class="Slide (strict)"("Scale.Maximum"=w1294) -> ()  [unwired: 2 in, 2 out]
            n611 = call "Elapsed Time55"("Time Target (s)"=w1294) -> ("Elapsed Time (s)"=w1293:dbl)  [unwired: 11 in, 7 out]
          }
          frame 11 {
            n612 = property on="Current Task time" class="Slide (strict)"("Scale.Maximum"=w1296) -> ()  [unwired: 2 in, 2 out]
            n613 = call "Elapsed Time56"("Time Target (s)"=w1296) -> ("Elapsed Time (s)"=w1295:dbl)  [unwired: 11 in, 7 out]
          }
          frame 12 {
            n614 = property on="Current Task time" class="Slide (strict)"("Scale.Maximum"=w1298) -> ()  [unwired: 2 in, 2 out]
            n615 = call "Elapsed Time57"("Time Target (s)"=w1298) -> ("Elapsed Time (s)"=w1297:dbl)  [unwired: 11 in, 7 out]
          }
          frame 13 {
            n616 = property on="Current Task time" class="Slide (strict)"("Scale.Maximum"=w1300) -> ()  [unwired: 2 in, 2 out]
            n617 = call "Elapsed Time124"("Time Target (s)"=w1300) -> ("Elapsed Time (s)"=w1299:dbl)  [unwired: 11 in, 7 out]
          }
          frame 0, Default {
            n618 = property on="Current Task time" class="Slide (strict)"("Scale.Maximum"=w1302) -> ()  [unwired: 2 in, 2 out]
            n619 = call "Elapsed Time125"("Time Target (s)"=w1302) -> ("Elapsed Time (s)"=w1301:dbl)  [unwired: 11 in, 7 out]
          }
        }
      }
      frame 7 {
        w1357 = 240.0  # Routine Time
        # "Routine 5: In car seat"
        n620 = property on="Total Routine Time" class="Slide (strict)"("Scale.Maximum"=w1357) -> ()  [unwired: 2 in, 2 out]
        n621 = call "Elapsed Time8"("Time Target (s)"=w1357, "Reset"=FALSE) -> ("Get Start Time (s)"=w1355:dbl, "Elapsed Time (s)"=w1349:dbl, "Time has Elapsed"=w1358:bool)  [unwired: 10 in, 5 out]
        "#5" <- w1358
        n622 = Seconds To Date/Time(time stamp (now)=w1355) -> (date time rec=w1356:T2)  [unwired: 1 in]
        n623 = Not(x=w1358) -> (.not. x?=w1361:bool)
        n624 = script code="t = [0,120,124,130,134,140,144,150,154,160,164,170,174,...\n       180,180.75,181.5,182.25,183,183.75,184.5,185.25,186,186.75,187.5,188.25,189,189.75,190.5,191.25,192,...\n       192.75,193.5,194.25,195,195.75,196.5,197.25,198,198.75,199.5,200.25,201,201.75,202.5,203.25,204,204.75,205.5,...\n       206.25,207,207.75,208.5,209.25,210,...\n        240];\n\nevent = [0,1,2,1,2,1,2,1,2,1,2,1,2,...\n               3,4,3,4,3,4,3,4,3,4,3,4,3,4,3,4,3,4,3,4,3,4,3,4,3,4,3,4,3,4,3,4,3,4,3,4,3,4,3,4,0,...\n               14];\n\nfor i = 2:length(t)\n    if ((x>=t(i-1)) &&  (x<t(i)))\n        y = event(i-1);\n        yNext = event(i);\n        dt = t(i) - t(i-1);\n        break;\n    end\nend"("x"=w1349) -> ("y"=w1352:dbl, "dt"=w1353:dbl, "yNext"=w1354:dbl)  [unwired: 1 in, 1 out]
        n625 = case shown="True" w1361 {
          tunnel: [w1417 w1429] -> w1360
          frame False {
            n626 = flat-sequence {
              tunnel: [w1425] -> w1417
              frame #0 {
                n627 = local write "Buffer"(FALSE ("Buffer")) -> ()
                n628 = local write "Play/Stop"(FALSE ("PlayInstr")) -> ()
              }
              frame #1 {
                n629 = local write "Output"(0 ("Output")) -> ()
                n630 = local write "Save"(TRUE ("Save")) -> ()
              }
              frame #2 {
                n631 = Wait (ms)(milliseconds to wait=u32 500) -> ()  [unwired: 1 out]
              }
              frame #3 {
                n632 = local write "Flush"(TRUE ("Flush")) -> ()
              }
              frame #4 {
                w1424 = u16 0 items=["No sound", "Demo deep breathing", "Demo fast shallow breathing", "Demo slow shallow breathing", "Demo breath hold", "Demo cough/ laugh", "Demo abdomen movement", "Calibration", "Routine 1", "Routine 3", "Routine 4/5/7", "Calm music"] ("Play sound")
                w1425 = enum16{"Default"}."Default"
                n633 = local write "Flush"(FALSE ("Flush")) -> ()
                n634 = local write "Save"(FALSE ("Save")) -> ()
                n635 = local write "Play sound"(w1424) -> ()
                n636 = local write "Routine"(w1425) -> ()
              }
            }
          }
          frame True {
            w1428 = u16 12 items=["No sound", "Demo normal breathing", "Demo deep breathing", "Demo fast shallow breathing", "Demo breath hold", "Demo cough", "Demo abdomen movement", "Calibration", "Routine 1", "(2a)Calm music", "(2b)Stress test", "Routine 3/4", "Routine 5"] ("Play sound")
            n637 = local write "Play sound"(w1428) -> ()
            n638 = flat-sequence {
              tunnel: [T4."Routine 5"] -> w1429
              frame #0 {
                n639 = local write "Output"(1 ("Open")) -> ()
                n640 = local write "Play/Stop"(TRUE ("PlayInstr")) -> ()
              }
              frame #1 {
                n641 = local write "Buffer"(TRUE ("Buffer")) -> ()
              }
              frame #2 {
              }
            }
          }
        }
        n642 = case shown="0, Default" w1352 {
          tunnel: ["\nPerform normal breathing." "Inhale a slow deep breath." "\nExhale slowly." "Quick inhale.\n\n\n\nIf you cannot sustain for long, resume normal breathing." "\nQuick exhale.\n\n\nIf you cannot sustain for long, resume normal breathing." "Slow shallow inhale.\n\n\n\nIf you cannot sustain for long, resume normal breathing." "\nSlow exhale.\n\n\nIf you cannot sustain for long, resume normal breathing." "Exhale the current breath  and HOLD.\n\n\nIf you cannot sustain for long, resume normal breathing." "Perform voluntary coughing \n" "Perform voluntary laugh\n\n" "Read aloud the following text in between the lines:\n-----------------------------------------------------------------------\nFour score and seven years ago our fathers brought forth on this continent, a new nation, conceived in Liberty, and dedicated to the proposition that all men are created equal… That this nation, under God, shall have a new birth of freedom-and that government of the people, by the people, for the people, shall not perish from the earth.\n\n-----------------------------------------------------------------------\nWhen finished, take a deep breath and open mouth say \"Ah\" (like doctor checking your throat).\nPerform normal breathing until next instruction." "Exhale current breath and HOLD. Push abdomen inwards." "Relax abdomen back to normal and keep holding breath."] -> w1350
          frame 0, Default {
          }
          frame 1 {
          }
          frame 2 {
          }
          frame 3 {
          }
          frame 4 {
          }
          frame 5 {
          }
          frame 6 {
          }
          frame 7 {
          }
          frame 8 {
          }
          frame 9 {
          }
          frame 10 {
          }
          frame 12 {
          }
          frame 13 {
          }
        }
        n643 = case shown="0, Default" w1354 {
          tunnel: ["\nPerform normal breathing." "Inhale a slow deep breath." "\nExhale slowly." "Quick inhale.\n\n\n\nIf you cannot sustain for long, resume normal breathing." "\nQuick exhale.\n\n\nIf you cannot sustain for long, resume normal breathing." "Slow shallow inhale.\n\n\n\nIf you cannot sustain for long, resume normal breathing." "\nSlow exhale.\n\n\nIf you cannot sustain for long, resume normal breathing." "Exhale the current breath  and HOLD.\n\n\nIf you cannot sustain for long, resume normal breathing." "Perform voluntary coughing \n" "Perform voluntary laugh\n\n" "Read aloud the following text in between the lines:\n-----------------------------------------------------------------------\nFour score and ...\n-----------------------------------------------------------------------\nWhen finished, take a deep breath and open mouth say \"Ah\" (like doctor checking your throat).\nPerform normal breathing until next instruction." "Exhale current breath and HOLD. Push abdomen inwards." "Relax abdomen back to normal and keep holding breath." "Study Completed!"] -> w1348
          frame 0, Default {
          }
          frame 1 {
          }
          frame 2 {
          }
          frame 3 {
          }
          frame 4 {
          }
          frame 5 {
          }
          frame 6 {
          }
          frame 7 {
          }
          frame 8 {
          }
          frame 9 {
          }
          frame 10 {
          }
          frame 12 {
          }
          frame 13 {
          }
          frame 14 {
          }
        }
        n644 = case shown="0, Default" w1352 {
          tunnel: w1353 -> [w1363 w1365 w1367 w1369 w1371 w1373 w1375 w1377 w1379 w1381 w1383 w1385 w1387 w1389]
          tunnel: [w1362 w1364 w1366 w1368 w1370 w1372 w1374 w1376 w1378 w1380 w1382 w1384 w1386 w1388] -> w1351
          frame 1 {
            n645 = property on="Current Task time" class="Slide (strict)"("Scale.Maximum"=w1363) -> ()  [unwired: 2 in, 2 out]
            n646 = call "Elapsed Time58"("Time Target (s)"=w1363) -> ("Elapsed Time (s)"=w1362:dbl)  [unwired: 11 in, 7 out]
          }
          frame 2 {
            n647 = property on="Current Task time" class="Slide (strict)"("Scale.Maximum"=w1365) -> ()  [unwired: 2 in, 2 out]
            n648 = call "Elapsed Time59"("Time Target (s)"=w1365) -> ("Elapsed Time (s)"=w1364:dbl)  [unwired: 11 in, 7 out]
          }
          frame 3 {
            n649 = property on="Current Task time" class="Slide (strict)"("Scale.Maximum"=w1367) -> ()  [unwired: 2 in, 2 out]
            n650 = call "Elapsed Time60"("Time Target (s)"=w1367) -> ("Elapsed Time (s)"=w1366:dbl)  [unwired: 11 in, 7 out]
          }
          frame 4 {
            n651 = property on="Current Task time" class="Slide (strict)"("Scale.Maximum"=w1369) -> ()  [unwired: 2 in, 2 out]
            n652 = call "Elapsed Time61"("Time Target (s)"=w1369) -> ("Elapsed Time (s)"=w1368:dbl)  [unwired: 11 in, 7 out]
          }
          frame 5 {
            n653 = property on="Current Task time" class="Slide (strict)"("Scale.Maximum"=w1371) -> ()  [unwired: 2 in, 2 out]
            n654 = call "Elapsed Time62"("Time Target (s)"=w1371) -> ("Elapsed Time (s)"=w1370:dbl)  [unwired: 11 in, 7 out]
          }
          frame 6 {
            n655 = property on="Current Task time" class="Slide (strict)"("Scale.Maximum"=w1373) -> ()  [unwired: 2 in, 2 out]
            n656 = call "Elapsed Time63"("Time Target (s)"=w1373) -> ("Elapsed Time (s)"=w1372:dbl)  [unwired: 11 in, 7 out]
          }
          frame 7 {
            n657 = property on="Current Task time" class="Slide (strict)"("Scale.Maximum"=w1375) -> ()  [unwired: 2 in, 2 out]
            n658 = call "Elapsed Time64"("Time Target (s)"=w1375) -> ("Elapsed Time (s)"=w1374:dbl)  [unwired: 11 in, 7 out]
          }
          frame 8 {
            n659 = property on="Current Task time" class="Slide (strict)"("Scale.Maximum"=w1377) -> ()  [unwired: 2 in, 2 out]
            n660 = call "Elapsed Time65"("Time Target (s)"=w1377) -> ("Elapsed Time (s)"=w1376:dbl)  [unwired: 11 in, 7 out]
          }
          frame 9 {
            n661 = property on="Current Task time" class="Slide (strict)"("Scale.Maximum"=w1379) -> ()  [unwired: 2 in, 2 out]
            n662 = call "Elapsed Time66"("Time Target (s)"=w1379) -> ("Elapsed Time (s)"=w1378:dbl)  [unwired: 11 in, 7 out]
          }
          frame 10 {
            n663 = property on="Current Task time" class="Slide (strict)"("Scale.Maximum"=w1381) -> ()  [unwired: 2 in, 2 out]
            n664 = call "Elapsed Time67"("Time Target (s)"=w1381) -> ("Elapsed Time (s)"=w1380:dbl)  [unwired: 11 in, 7 out]
          }
          frame 11 {
            n665 = property on="Current Task time" class="Slide (strict)"("Scale.Maximum"=w1383) -> ()  [unwired: 2 in, 2 out]
            n666 = call "Elapsed Time68"("Time Target (s)"=w1383) -> ("Elapsed Time (s)"=w1382:dbl)  [unwired: 11 in, 7 out]
          }
          frame 12 {
            n667 = property on="Current Task time" class="Slide (strict)"("Scale.Maximum"=w1385) -> ()  [unwired: 2 in, 2 out]
            n668 = call "Elapsed Time69"("Time Target (s)"=w1385) -> ("Elapsed Time (s)"=w1384:dbl)  [unwired: 11 in, 7 out]
          }
          frame 13 {
            n669 = property on="Current Task time" class="Slide (strict)"("Scale.Maximum"=w1387) -> ()  [unwired: 2 in, 2 out]
            n670 = call "Elapsed Time126"("Time Target (s)"=w1387) -> ("Elapsed Time (s)"=w1386:dbl)  [unwired: 11 in, 7 out]
          }
          frame 0, Default {
            n671 = property on="Current Task time" class="Slide (strict)"("Scale.Maximum"=w1389) -> ()  [unwired: 2 in, 2 out]
            n672 = call "Elapsed Time127"("Time Target (s)"=w1389) -> ("Elapsed Time (s)"=w1388:dbl)  [unwired: 11 in, 7 out]
          }
        }
      }
      frame 8 {
        w1443 = 35.0  # Routine Time
        # "Calibration Routine 1"
        n673 = property on="Total Routine Time" class="Slide (strict)"("Scale.Maximum"=w1443) -> ()  [unwired: 2 in, 2 out]
        n674 = call "Elapsed Time71"("Time Target (s)"=w1443, "Auto Reset"=FALSE ("Timer Reset")) -> ("Get Start Time (s)"=w1441:dbl, "Elapsed Time (s)"=w1437:dbl, "Time has Elapsed"=w1444:bool)  [unwired: 10 in, 5 out]
        "Calib 1" <- w1444
        n675 = Seconds To Date/Time(time stamp (now)=w1441) -> (date time rec=w1442:T2)  [unwired: 1 in]
        n676 = Not(x=w1444) -> (.not. x?=w1447:bool)
        n677 = script code="t = [0,20,23,27.5,30.5,35];\n\nevent = [0,1,2,1,2,14];\n\nfor i = 2:length(t)\n    if ((x>=t(i-1)) &&  (x<t(i)))\n        y = event(i-1);\n        yNext = event(i);\n        dt = t(i) - t(i-1);\n        break;\n    end\nend"("x"=w1437) -> ("y"=w1438:dbl, "dt"=w1439:dbl, "yNext"=w1440:dbl)  [unwired: 1 in, 1 out]
        n678 = case shown="True" w1447 {
          tunnel: [w1486 w1498] -> w1446
          frame False {
            n679 = flat-sequence {
              tunnel: [w1494] -> w1486
              frame #0 {
                n680 = local write "Buffer"(FALSE ("Buffer")) -> ()
                n681 = local write "Play/Stop"(FALSE ("Play\nCalibration")) -> ()
              }
              frame #1 {
                n682 = local write "Output"(0 ("Output")) -> ()
                n683 = local write "Save"(TRUE ("Save")) -> ()
              }
              frame #2 {
                n684 = Wait (ms)(milliseconds to wait=u32 500) -> ()  [unwired: 1 out]
              }
              frame #3 {
                n685 = local write "Flush"(TRUE ("Flush")) -> ()
              }
              frame #4 {
                w1493 = u16 0 items=["No sound", "Demo deep breathing", "Demo fast shallow breathing", "Demo slow shallow breathing", "Demo breath hold", "Demo cough/ laugh", "Demo abdomen movement", "Calibration", "Routine 1", "Routine 3", "Routine 4/5/7", "Calm music"] ("Play sound")
                w1494 = enum16{"Default"}."Default"
                n686 = local write "Flush"(FALSE ("Flush")) -> ()
                n687 = local write "Save"(FALSE ("Save")) -> ()
                n688 = local write "Routine"(w1494) -> ()
                n689 = local write "Play sound"(w1493) -> ()
              }
            }
          }
          frame True {
            w1497 = u16 7 items=["No sound", "Demo normal breathing", "Demo deep breathing", "Demo fast shallow breathing", "Demo breath hold", "Demo cough", "Demo abdomen movement", "Calibration", "Routine 1", "(2a)Calm music", "(2b)Stress test", "Routine 3/4", "Routine 5", ""] ("Play sound")
            n690 = local write "Play sound"(w1497) -> ()
            n691 = flat-sequence {
              tunnel: [T4."Calib1"] -> w1498
              frame #0 {
                n692 = local write "Play/Stop"(TRUE ("Play\nCalibration")) -> ()
                n693 = local write "Output"(1 ("Open")) -> ()
              }
              frame #1 {
                n694 = local write "Buffer"(TRUE ("Buffer")) -> ()
              }
              frame #2 {
              }
            }
          }
        }
        n695 = case shown="0, Default" w1438 {
          tunnel: ["\nPerform normal breathing." "Inhale a slow deep breath." "\nExhale slowly." "Quick inhale.\n\n\n\nIf you cannot sustain for long, resume normal breathing." "\nQuick exhale.\n\n\nIf you cannot sustain for long, resume normal breathing." "Slow shallow inhale.\n\n\n\nIf you cannot sustain for long, resume normal breathing." "\nSlow exhale.\n\n\nIf you cannot sustain for long, resume normal breathing." "Exhale the current breath  and HOLD.\n\n\nIf you cannot sustain for long, resume normal breathing." "Perform voluntary coughing \n" "Perform voluntary laugh\n\n" "Read aloud the following text in between the lines:\n-----------------------------------------------------------------------\nFour score and seven years ago our fathers brought forth on this continent, a new nation, conceived in Liberty, and dedicated to the proposition that all men are created equal… That this nation, under God, shall have a new birth of freedom-and that government of the people, by the people, for the people, shall not perish from the earth.\n\n-----------------------------------------------------------------------\nWhen finished, take a deep breath and open mouth say \"Ah\" (like doctor checking your throat).\nPerform normal breathing until next instruction." "Exhale current breath and HOLD. Push abdomen inwards." "Relax abdomen back to normal and keep holding breath."] -> w1436
          frame 0, Default {
          }
          frame 1 {
          }
          frame 2 {
          }
          frame 3 {
          }
          frame 4 {
          }
          frame 5 {
          }
          frame 6 {
          }
          frame 7 {
          }
          frame 8 {
          }
          frame 9 {
          }
          frame 10 {
          }
          frame 12 {
          }
          frame 13 {
          }
        }
        n696 = case shown="14" w1440 {
          tunnel: ["\nPerform normal breathing." "Inhale a slow deep breath." "\nExhale slowly." "Quick inhale.\n\n\n\nIf you cannot sustain for long, resume normal breathing." "\nQuick exhale.\n\n\nIf you cannot sustain for long, resume normal breathing." "Slow shallow inhale.\n\n\n\nIf you cannot sustain for long, resume normal breathing." "\nSlow exhale.\n\n\nIf you cannot sustain for long, resume normal breathing." "Exhale the current breath  and HOLD.\n\n\nIf you cannot sustain for long, resume normal breathing." "Perform voluntary coughing \n" "Perform voluntary laugh\n\n" "Read aloud the following text in between the lines:\n-----------------------------------------------------------------------\nFour score and ...\n-----------------------------------------------------------------------\nWhen finished, take a deep breath and open mouth say \"Ah\" (like doctor checking your throat).\nPerform normal breathing until next instruction." "Exhale current breath and HOLD. Push abdomen inwards." "Relax abdomen back to normal and keep holding breath." "Wait for next routine. Please do not move."] -> w1434
          frame 0, Default {
          }
          frame 1 {
          }
          frame 2 {
          }
          frame 3 {
          }
          frame 4 {
          }
          frame 5 {
          }
          frame 6 {
          }
          frame 7 {
          }
          frame 8 {
          }
          frame 9 {
          }
          frame 10 {
          }
          frame 12 {
          }
          frame 13 {
          }
          frame 14 {
          }
        }
        n697 = case shown="0, Default" w1438 {
          tunnel: w1439 -> [w1450 w1452 w1454 w1456 w1458]
          tunnel: [w1449 w1451 w1453 w1455 w1457] -> w1435
          frame 1 {
            n698 = property on="Current Task time" class="Slide (strict)"("Scale.Maximum"=w1450) -> ()  [unwired: 2 in, 2 out]
            n699 = call "Elapsed Time72"("Time Target (s)"=w1450) -> ("Elapsed Time (s)"=w1449:dbl)  [unwired: 11 in, 7 out]
          }
          frame 2 {
            n700 = property on="Current Task time" class="Slide (strict)"("Scale.Maximum"=w1452) -> ()  [unwired: 2 in, 2 out]
            n701 = call "Elapsed Time73"("Time Target (s)"=w1452) -> ("Elapsed Time (s)"=w1451:dbl)  [unwired: 11 in, 7 out]
          }
          frame 3 {
            n702 = property on="Current Task time" class="Slide (strict)"("Scale.Maximum"=w1454) -> ()  [unwired: 2 in, 2 out]
            n703 = call "Elapsed Time74"("Time Target (s)"=w1454) -> ("Elapsed Time (s)"=w1453:dbl)  [unwired: 11 in, 7 out]
          }
          frame 4 {
            n704 = property on="Current Task time" class="Slide (strict)"("Scale.Maximum"=w1456) -> ()  [unwired: 2 in, 2 out]
            n705 = call "Elapsed Time75"("Time Target (s)"=w1456) -> ("Elapsed Time (s)"=w1455:dbl)  [unwired: 11 in, 7 out]
          }
          frame 0, Default {
            n706 = property on="Current Task time" class="Slide (strict)"("Scale.Maximum"=w1458) -> ()  [unwired: 2 in, 2 out]
            n707 = call "Elapsed Time134"("Time Target (s)"=w1458) -> ("Elapsed Time (s)"=w1457:dbl)  [unwired: 11 in, 7 out]
          }
        }
      }
      frame 9 {
        w1512 = 35.0  # Routine Time
        # "Calibration Routine 3"
        n708 = property on="Total Routine Time" class="Slide (strict)"("Scale.Maximum"=w1512) -> ()  [unwired: 2 in, 2 out]
        n709 = call "Elapsed Time76"("Time Target (s)"=w1512, "Auto Reset"=FALSE ("Timer Reset")) -> ("Get Start Time (s)"=w1510:dbl, "Elapsed Time (s)"=w1506:dbl, "Time has Elapsed"=w1513:bool)  [unwired: 10 in, 5 out]
        "Calib 3" <- w1513
        n710 = Seconds To Date/Time(time stamp (now)=w1510) -> (date time rec=w1511:T2)  [unwired: 1 in]
        n711 = Not(x=w1513) -> (.not. x?=w1516:bool)
        n712 = script code="t = [0,20,23,27.5,30.5,35];\n\nevent = [0,1,2,1,2,14];\n\nfor i = 2:length(t)\n    if ((x>=t(i-1)) &&  (x<t(i)))\n        y = event(i-1);\n        yNext = event(i);\n        dt = t(i) - t(i-1);\n        break;\n    end\nend"("x"=w1506) -> ("y"=w1507:dbl, "dt"=w1508:dbl, "yNext"=w1509:dbl)  [unwired: 1 in, 1 out]
        n713 = case shown="True" w1516 {
          tunnel: [w1555 w1567] -> w1515
          frame False {
            n714 = flat-sequence {
              tunnel: [w1563] -> w1555
              frame #0 {
                n715 = local write "Buffer"(FALSE ("Buffer")) -> ()
                n716 = local write "Play/Stop"(FALSE ("Play\nCalibration")) -> ()
              }
              frame #1 {
                n717 = local write "Output"(0 ("Output")) -> ()
                n718 = local write "Save"(TRUE ("Save")) -> ()
              }
              frame #2 {
                n719 = Wait (ms)(milliseconds to wait=u32 500) -> ()  [unwired: 1 out]
              }
              frame #3 {
                n720 = local write "Flush"(TRUE ("Flush")) -> ()
              }
              frame #4 {
                w1562 = u16 0 items=["No sound", "Demo deep breathing", "Demo fast shallow breathing", "Demo slow shallow breathing", "Demo breath hold", "Demo cough/ laugh", "Demo abdomen movement", "Calibration", "Routine 1", "Routine 3", "Routine 4/5/7", "Calm music"] ("Play sound")
                w1563 = enum16{"Default"}."Default"
                n721 = local write "Flush"(FALSE ("Flush")) -> ()
                n722 = local write "Save"(FALSE ("Save")) -> ()
                n723 = local write "Routine"(w1563) -> ()
                n724 = local write "Play sound"(w1562) -> ()
              }
            }
          }
          frame True {
            w1566 = u16 7 items=["No sound", "Demo normal breathing", "Demo deep breathing", "Demo fast shallow breathing", "Demo breath hold", "Demo cough", "Demo abdomen movement", "Calibration", "Routine 1", "(2a)Calm music", "(2b)Stress test", "Routine 3/4", "Routine 5", ""] ("Play sound")
            n725 = local write "Play sound"(w1566) -> ()
            n726 = flat-sequence {
              tunnel: [T4."Calib3"] -> w1567
              frame #0 {
                n727 = local write "Output"(1 ("Open")) -> ()
                n728 = local write "Play/Stop"(TRUE ("Play\nCalibration")) -> ()
              }
              frame #1 {
                n729 = local write "Buffer"(TRUE ("Buffer")) -> ()
              }
              frame #2 {
              }
            }
          }
        }
        n730 = case shown="0, Default" w1507 {
          tunnel: ["\nPerform normal breathing." "Inhale a slow deep breath." "\nExhale slowly." "Quick inhale.\n\n\n\nIf you cannot sustain for long, resume normal breathing." "\nQuick exhale.\n\n\nIf you cannot sustain for long, resume normal breathing." "Slow shallow inhale.\n\n\n\nIf you cannot sustain for long, resume normal breathing." "\nSlow exhale.\n\n\nIf you cannot sustain for long, resume normal breathing." "Exhale the current breath  and HOLD.\n\n\nIf you cannot sustain for long, resume normal breathing." "Perform voluntary coughing \n" "Perform voluntary laugh\n\n" "Read aloud the following text in between the lines:\n-----------------------------------------------------------------------\nFour score and seven years ago our fathers brought forth on this continent, a new nation, conceived in Liberty, and dedicated to the proposition that all men are created equal… That this nation, under God, shall have a new birth of freedom-and that government of the people, by the people, for the people, shall not perish from the earth.\n\n-----------------------------------------------------------------------\nWhen finished, take a deep breath and open mouth say \"Ah\" (like doctor checking your throat).\nPerform normal breathing until next instruction." "Exhale current breath and HOLD. Push abdomen inwards." "Relax abdomen back to normal and keep holding breath."] -> w1505
          frame 0, Default {
          }
          frame 1 {
          }
          frame 2 {
          }
          frame 3 {
          }
          frame 4 {
          }
          frame 5 {
          }
          frame 6 {
          }
          frame 7 {
          }
          frame 8 {
          }
          frame 9 {
          }
          frame 10 {
          }
          frame 12 {
          }
          frame 13 {
          }
        }
        n731 = case shown="14" w1509 {
          tunnel: ["\nPerform normal breathing." "Inhale a slow deep breath." "\nExhale slowly." "Quick inhale.\n\n\n\nIf you cannot sustain for long, resume normal breathing." "\nQuick exhale.\n\n\nIf you cannot sustain for long, resume normal breathing." "Slow shallow inhale.\n\n\n\nIf you cannot sustain for long, resume normal breathing." "\nSlow exhale.\n\n\nIf you cannot sustain for long, resume normal breathing." "Exhale the current breath  and HOLD.\n\n\nIf you cannot sustain for long, resume normal breathing." "Perform voluntary coughing \n" "Perform voluntary laugh\n\n" "Read aloud the following text in between the lines:\n-----------------------------------------------------------------------\nFour score and ...\n-----------------------------------------------------------------------\nWhen finished, take a deep breath and open mouth say \"Ah\" (like doctor checking your throat).\nPerform normal breathing until next instruction." "Exhale current breath and HOLD. Push abdomen inwards." "Relax abdomen back to normal and keep holding breath." "Wait for next routine. Please do not move."] -> w1503
          frame 0, Default {
          }
          frame 1 {
          }
          frame 2 {
          }
          frame 3 {
          }
          frame 4 {
          }
          frame 5 {
          }
          frame 6 {
          }
          frame 7 {
          }
          frame 8 {
          }
          frame 9 {
          }
          frame 10 {
          }
          frame 12 {
          }
          frame 13 {
          }
          frame 14 {
          }
        }
        n732 = case shown="0, Default" w1507 {
          tunnel: w1508 -> [w1519 w1521 w1523 w1525 w1527]
          tunnel: [w1518 w1520 w1522 w1524 w1526] -> w1504
          frame 1 {
            n733 = property on="Current Task time" class="Slide (strict)"("Scale.Maximum"=w1519) -> ()  [unwired: 2 in, 2 out]
            n734 = call "Elapsed Time77"("Time Target (s)"=w1519) -> ("Elapsed Time (s)"=w1518:dbl)  [unwired: 11 in, 7 out]
          }
          frame 2 {
            n735 = property on="Current Task time" class="Slide (strict)"("Scale.Maximum"=w1521) -> ()  [unwired: 2 in, 2 out]
            n736 = call "Elapsed Time78"("Time Target (s)"=w1521) -> ("Elapsed Time (s)"=w1520:dbl)  [unwired: 11 in, 7 out]
          }
          frame 3 {
            n737 = property on="Current Task time" class="Slide (strict)"("Scale.Maximum"=w1523) -> ()  [unwired: 2 in, 2 out]
            n738 = call "Elapsed Time79"("Time Target (s)"=w1523) -> ("Elapsed Time (s)"=w1522:dbl)  [unwired: 11 in, 7 out]
          }
          frame 4 {
            n739 = property on="Current Task time" class="Slide (strict)"("Scale.Maximum"=w1525) -> ()  [unwired: 2 in, 2 out]
            n740 = call "Elapsed Time80"("Time Target (s)"=w1525) -> ("Elapsed Time (s)"=w1524:dbl)  [unwired: 11 in, 7 out]
          }
          frame 0, Default {
            n741 = property on="Current Task time" class="Slide (strict)"("Scale.Maximum"=w1527) -> ()  [unwired: 2 in, 2 out]
            n742 = call "Elapsed Time81"("Time Target (s)"=w1527) -> ("Elapsed Time (s)"=w1526:dbl)  [unwired: 11 in, 7 out]
          }
        }
      }
      frame 10 {
        w1581 = 35.0  # Routine Time
        # "Calibration 4"
        n743 = property on="Total Routine Time" class="Slide (strict)"("Scale.Maximum"=w1581) -> ()  [unwired: 2 in, 2 out]
        n744 = call "Elapsed Time82"("Time Target (s)"=w1581, "Auto Reset"=FALSE ("Timer Reset")) -> ("Get Start Time (s)"=w1579:dbl, "Elapsed Time (s)"=w1575:dbl, "Time has Elapsed"=w1582:bool)  [unwired: 10 in, 5 out]
        "Calib 4" <- w1582
        n745 = Seconds To Date/Time(time stamp (now)=w1579) -> (date time rec=w1580:T2)  [unwired: 1 in]
        n746 = Not(x=w1582) -> (.not. x?=w1585:bool)
        n747 = script code="t = [0,20,23,27.5,30.5,35];\n\nevent = [0,1,2,1,2,14];\n\nfor i = 2:length(t)\n    if ((x>=t(i-1)) &&  (x<t(i)))\n        y = event(i-1);\n        yNext = event(i);\n        dt = t(i) - t(i-1);\n        break;\n    end\nend"("x"=w1575) -> ("y"=w1576:dbl, "dt"=w1577:dbl, "yNext"=w1578:dbl)  [unwired: 1 in, 1 out]
        n748 = case shown="True" w1585 {
          tunnel: [w1624 w1636] -> w1584
          frame False {
            n749 = flat-sequence {
              tunnel: [w1632] -> w1624
              frame #0 {
                n750 = local write "Buffer"(FALSE ("Buffer")) -> ()
                n751 = local write "Play/Stop"(FALSE ("Play\nCalibration")) -> ()
              }
              frame #1 {
                n752 = local write "Output"(0 ("Output")) -> ()
                n753 = local write "Save"(TRUE ("Save")) -> ()
              }
              frame #2 {
                n754 = Wait (ms)(milliseconds to wait=u32 500) -> ()  [unwired: 1 out]
              }
              frame #3 {
                n755 = local write "Flush"(TRUE ("Flush")) -> ()
              }
              frame #4 {
                w1631 = u16 0 items=["No sound", "Demo deep breathing", "Demo fast shallow breathing", "Demo slow shallow breathing", "Demo breath hold", "Demo cough/ laugh", "Demo abdomen movement", "Calibration", "Routine 1", "Routine 3", "Routine 4/5/7", "Calm music"] ("Play sound")
                w1632 = enum16{"Default", ""}."Default"
                n756 = local write "Flush"(FALSE ("Flush")) -> ()
                n757 = local write "Save"(FALSE ("Save")) -> ()
                n758 = local write "Routine"(w1632) -> ()
                n759 = local write "Play sound"(w1631) -> ()
              }
            }
          }
          frame True {
            w1635 = u16 7 items=["No sound", "Demo normal breathing", "Demo deep breathing", "Demo fast shallow breathing", "Demo breath hold", "Demo cough", "Demo abdomen movement", "Calibration", "Routine 1", "(2a)Calm music", "(2b)Stress test", "Routine 3/4", "Routine 5", ""] ("Play sound")
            n760 = local write "Play sound"(w1635) -> ()
            n761 = flat-sequence {
              tunnel: [T4."Calib4"] -> w1636
              frame #0 {
                n762 = local write "Output"(1 ("Open")) -> ()
                n763 = local write "Play/Stop"(TRUE ("Play\nCalibration")) -> ()
              }
              frame #1 {
                n764 = local write "Buffer"(TRUE ("Buffer")) -> ()
              }
              frame #2 {
              }
            }
          }
        }
        n765 = case shown="0, Default" w1576 {
          tunnel: ["\nPerform normal breathing." "Inhale a slow deep breath." "\nExhale slowly." "Quick inhale.\n\n\n\nIf you cannot sustain for long, resume normal breathing." "\nQuick exhale.\n\n\nIf you cannot sustain for long, resume normal breathing." "Slow shallow inhale.\n\n\n\nIf you cannot sustain for long, resume normal breathing." "\nSlow exhale.\n\n\nIf you cannot sustain for long, resume normal breathing." "Exhale the current breath  and HOLD.\n\n\nIf you cannot sustain for long, resume normal breathing." "Perform voluntary coughing \n" "Perform voluntary laugh\n\n" "Read aloud the following text in between the lines:\n-----------------------------------------------------------------------\nFour score and seven years ago our fathers brought forth on this continent, a new nation, conceived in Liberty, and dedicated to the proposition that all men are created equal… That this nation, under God, shall have a new birth of freedom-and that government of the people, by the people, for the people, shall not perish from the earth.\n\n-----------------------------------------------------------------------\nWhen finished, take a deep breath and open mouth say \"Ah\" (like doctor checking your throat).\nPerform normal breathing until next instruction." "Exhale current breath and HOLD. Push abdomen inwards." "Relax abdomen back to normal and keep holding breath."] -> w1574
          frame 0, Default {
          }
          frame 1 {
          }
          frame 2 {
          }
          frame 3 {
          }
          frame 4 {
          }
          frame 5 {
          }
          frame 6 {
          }
          frame 7 {
          }
          frame 8 {
          }
          frame 9 {
          }
          frame 10 {
          }
          frame 12 {
          }
          frame 13 {
          }
        }
        n766 = case shown="14" w1578 {
          tunnel: ["\nPerform normal breathing." "Inhale a slow deep breath." "\nExhale slowly." "Quick inhale.\n\n\n\nIf you cannot sustain for long, resume normal breathing." "\nQuick exhale.\n\n\nIf you cannot sustain for long, resume normal breathing." "Slow shallow inhale.\n\n\n\nIf you cannot sustain for long, resume normal breathing." "\nSlow exhale.\n\n\nIf you cannot sustain for long, resume normal breathing." "Exhale the current breath  and HOLD.\n\n\nIf you cannot sustain for long, resume normal breathing." "Perform voluntary coughing \n" "Perform voluntary laugh\n\n" "Read aloud the following text in between the lines:\n-----------------------------------------------------------------------\nFour score and ...\n-----------------------------------------------------------------------\nWhen finished, take a deep breath and open mouth say \"Ah\" (like doctor checking your throat).\nPerform normal breathing until next instruction." "Exhale current breath and HOLD. Push abdomen inwards." "Relax abdomen back to normal and keep holding breath." "Wait for next routine. Please do not move."] -> w1572
          frame 0, Default {
          }
          frame 1 {
          }
          frame 2 {
          }
          frame 3 {
          }
          frame 4 {
          }
          frame 5 {
          }
          frame 6 {
          }
          frame 7 {
          }
          frame 8 {
          }
          frame 9 {
          }
          frame 10 {
          }
          frame 12 {
          }
          frame 13 {
          }
          frame 14 {
          }
        }
        n767 = case shown="0, Default" w1576 {
          tunnel: w1577 -> [w1588 w1590 w1592 w1594 w1596]
          tunnel: [w1587 w1589 w1591 w1593 w1595] -> w1573
          frame 1 {
            n768 = property on="Current Task time" class="Slide (strict)"("Scale.Maximum"=w1588) -> ()  [unwired: 2 in, 2 out]
            n769 = call "Elapsed Time83"("Time Target (s)"=w1588) -> ("Elapsed Time (s)"=w1587:dbl)  [unwired: 11 in, 7 out]
          }
          frame 2 {
            n770 = property on="Current Task time" class="Slide (strict)"("Scale.Maximum"=w1590) -> ()  [unwired: 2 in, 2 out]
            n771 = call "Elapsed Time84"("Time Target (s)"=w1590) -> ("Elapsed Time (s)"=w1589:dbl)  [unwired: 11 in, 7 out]
          }
          frame 3 {
            n772 = property on="Current Task time" class="Slide (strict)"("Scale.Maximum"=w1592) -> ()  [unwired: 2 in, 2 out]
            n773 = call "Elapsed Time85"("Time Target (s)"=w1592) -> ("Elapsed Time (s)"=w1591:dbl)  [unwired: 11 in, 7 out]
          }
          frame 4 {
            n774 = property on="Current Task time" class="Slide (strict)"("Scale.Maximum"=w1594) -> ()  [unwired: 2 in, 2 out]
            n775 = call "Elapsed Time86"("Time Target (s)"=w1594) -> ("Elapsed Time (s)"=w1593:dbl)  [unwired: 11 in, 7 out]
          }
          frame 0, Default {
            n776 = property on="Current Task time" class="Slide (strict)"("Scale.Maximum"=w1596) -> ()  [unwired: 2 in, 2 out]
            n777 = call "Elapsed Time87"("Time Target (s)"=w1596) -> ("Elapsed Time (s)"=w1595:dbl)  [unwired: 11 in, 7 out]
          }
        }
      }
      frame 11 {
        w1650 = 35.0  # Routine Time
        # "Calibration Routine 5"
        n778 = property on="Total Routine Time" class="Slide (strict)"("Scale.Maximum"=w1650) -> ()  [unwired: 2 in, 2 out]
        n779 = call "Elapsed Time88"("Time Target (s)"=w1650, "Auto Reset"=FALSE ("Timer Reset")) -> ("Get Start Time (s)"=w1648:dbl, "Elapsed Time (s)"=w1644:dbl, "Time has Elapsed"=w1651:bool)  [unwired: 10 in, 5 out]
        "Calib 5" <- w1651
        n780 = Seconds To Date/Time(time stamp (now)=w1648) -> (date time rec=w1649:T2)  [unwired: 1 in]
        n781 = Not(x=w1651) -> (.not. x?=w1654:bool)
        n782 = script code="t = [0,20,23,27.5,30.5,35];\n\nevent = [0,1,2,1,2,14];\n\nfor i = 2:length(t)\n    if ((x>=t(i-1)) &&  (x<t(i)))\n        y = event(i-1);\n        yNext = event(i);\n        dt = t(i) - t(i-1);\n        break;\n    end\nend"("x"=w1644) -> ("y"=w1645:dbl, "dt"=w1646:dbl, "yNext"=w1647:dbl)  [unwired: 1 in, 1 out]
        n783 = case shown="True" w1654 {
          tunnel: [w1693 w1705] -> w1653
          frame False {
            n784 = flat-sequence {
              tunnel: [w1701] -> w1693
              frame #0 {
                n785 = local write "Buffer"(FALSE ("Buffer")) -> ()
                n786 = local write "Play/Stop"(FALSE ("Play\nCalibration")) -> ()
              }
              frame #1 {
                n787 = local write "Output"(0 ("Output")) -> ()
                n788 = local write "Save"(TRUE ("Save")) -> ()
              }
              frame #2 {
                n789 = Wait (ms)(milliseconds to wait=u32 500) -> ()  [unwired: 1 out]
              }
              frame #3 {
                n790 = local write "Flush"(TRUE ("Flush")) -> ()
              }
              frame #4 {
                w1700 = u16 0 items=["No sound", "Demo deep breathing", "Demo fast shallow breathing", "Demo slow shallow breathing", "Demo breath hold", "Demo cough/ laugh", "Demo abdomen movement", "Calibration", "Routine 1", "Routine 3", "Routine 4/5/7", "Calm music"] ("Play sound")
                w1701 = enum16{"Default"}."Default"
                n791 = local write "Flush"(FALSE ("Flush")) -> ()
                n792 = local write "Save"(FALSE ("Save")) -> ()
                n793 = local write "Play sound"(w1700) -> ()
                n794 = local write "Routine"(w1701) -> ()
              }
            }
          }
          frame True {
            w1704 = u16 7 items=["No sound", "Demo normal breathing", "Demo deep breathing", "Demo fast shallow breathing", "Demo breath hold", "Demo cough", "Demo abdomen movement", "Calibration", "Routine 1", "(2a)Calm music", "(2b)Stress test", "Routine 3/4", "Routine 5", ""] ("Play sound")
            n795 = local write "Play sound"(w1704) -> ()
            n796 = flat-sequence {
              tunnel: [T4."Calib4"] -> w1705
              frame #0 {
                n797 = local write "Output"(1 ("Open")) -> ()
                n798 = local write "Play/Stop"(TRUE ("Play\nCalibration")) -> ()
              }
              frame #1 {
                n799 = local write "Buffer"(TRUE ("Buffer")) -> ()
              }
              frame #2 {
              }
            }
          }
        }
        n800 = case shown="0, Default" w1645 {
          tunnel: ["\nPerform normal breathing." "Inhale a slow deep breath." "\nExhale slowly." "Quick inhale.\n\n\n\nIf you cannot sustain for long, resume normal breathing." "\nQuick exhale.\n\n\nIf you cannot sustain for long, resume normal breathing." "Slow shallow inhale.\n\n\n\nIf you cannot sustain for long, resume normal breathing." "\nSlow exhale.\n\n\nIf you cannot sustain for long, resume normal breathing." "Exhale the current breath  and HOLD.\n\n\nIf you cannot sustain for long, resume normal breathing." "Perform voluntary coughing \n" "Perform voluntary laugh\n\n" "Read aloud the following text in between the lines:\n-----------------------------------------------------------------------\nFour score and seven years ago our fathers brought forth on this continent, a new nation, conceived in Liberty, and dedicated to the proposition that all men are created equal… That this nation, under God, shall have a new birth of freedom-and that government of the people, by the people, for the people, shall not perish from the earth.\n\n-----------------------------------------------------------------------\nWhen finished, take a deep breath and open mouth say \"Ah\" (like doctor checking your throat).\nPerform normal breathing until next instruction." "Exhale current breath and HOLD. Push abdomen inwards." "Relax abdomen back to normal and keep holding breath."] -> w1643
          frame 0, Default {
          }
          frame 1 {
          }
          frame 2 {
          }
          frame 3 {
          }
          frame 4 {
          }
          frame 5 {
          }
          frame 6 {
          }
          frame 7 {
          }
          frame 8 {
          }
          frame 9 {
          }
          frame 10 {
          }
          frame 12 {
          }
          frame 13 {
          }
        }
        n801 = case shown="14" w1647 {
          tunnel: ["\nPerform normal breathing." "Inhale a slow deep breath." "\nExhale slowly." "Quick inhale.\n\n\n\nIf you cannot sustain for long, resume normal breathing." "\nQuick exhale.\n\n\nIf you cannot sustain for long, resume normal breathing." "Slow shallow inhale.\n\n\n\nIf you cannot sustain for long, resume normal breathing." "\nSlow exhale.\n\n\nIf you cannot sustain for long, resume normal breathing." "Exhale the current breath  and HOLD.\n\n\nIf you cannot sustain for long, resume normal breathing." "Perform voluntary coughing \n" "Perform voluntary laugh\n\n" "Read aloud the following text in between the lines:\n-----------------------------------------------------------------------\nFour score and ...\n-----------------------------------------------------------------------\nWhen finished, take a deep breath and open mouth say \"Ah\" (like doctor checking your throat).\nPerform normal breathing until next instruction." "Exhale current breath and HOLD. Push abdomen inwards." "Relax abdomen back to normal and keep holding breath." "Wait for next routine. Please do not move."] -> w1641
          frame 0, Default {
          }
          frame 1 {
          }
          frame 2 {
          }
          frame 3 {
          }
          frame 4 {
          }
          frame 5 {
          }
          frame 6 {
          }
          frame 7 {
          }
          frame 8 {
          }
          frame 9 {
          }
          frame 10 {
          }
          frame 12 {
          }
          frame 13 {
          }
          frame 14 {
          }
        }
        n802 = case shown="0, Default" w1645 {
          tunnel: w1646 -> [w1657 w1659 w1661 w1663 w1665]
          tunnel: [w1656 w1658 w1660 w1662 w1664] -> w1642
          frame 1 {
            n803 = property on="Current Task time" class="Slide (strict)"("Scale.Maximum"=w1657) -> ()  [unwired: 2 in, 2 out]
            n804 = call "Elapsed Time89"("Time Target (s)"=w1657) -> ("Elapsed Time (s)"=w1656:dbl)  [unwired: 11 in, 7 out]
          }
          frame 2 {
            n805 = property on="Current Task time" class="Slide (strict)"("Scale.Maximum"=w1659) -> ()  [unwired: 2 in, 2 out]
            n806 = call "Elapsed Time90"("Time Target (s)"=w1659) -> ("Elapsed Time (s)"=w1658:dbl)  [unwired: 11 in, 7 out]
          }
          frame 3 {
            n807 = property on="Current Task time" class="Slide (strict)"("Scale.Maximum"=w1661) -> ()  [unwired: 2 in, 2 out]
            n808 = call "Elapsed Time91"("Time Target (s)"=w1661) -> ("Elapsed Time (s)"=w1660:dbl)  [unwired: 11 in, 7 out]
          }
          frame 4 {
            n809 = property on="Current Task time" class="Slide (strict)"("Scale.Maximum"=w1663) -> ()  [unwired: 2 in, 2 out]
            n810 = call "Elapsed Time92"("Time Target (s)"=w1663) -> ("Elapsed Time (s)"=w1662:dbl)  [unwired: 11 in, 7 out]
          }
          frame 0, Default {
            n811 = property on="Current Task time" class="Slide (strict)"("Scale.Maximum"=w1665) -> ()  [unwired: 2 in, 2 out]
            n812 = call "Elapsed Time93"("Time Target (s)"=w1665) -> ("Elapsed Time (s)"=w1664:dbl)  [unwired: 11 in, 7 out]
          }
        }
      }
    }
    "CaseNum" <- w996
    "Elapsed Time (s)" <- w994
    "Current Task" <- w995
    "Total Routine Time" <- w994
    "date time rec" <- w993
    "Current Task time" <- w992
    "Next Task" <- w990
    n813 = Wait (ms)(milliseconds to wait=u32 2 ("millisecond timer value")) -> ()  [unwired: 1 out]
    n814 = property on="Current Task time" class="Slide (strict)"("Scale.Minimum"=0.0 ("Scale.Range:Minimum")) -> ()  [unwired: 2 in, 2 out]
  }
  n815 = while {
    tunnel: w108 -> [w1713]
    tunnel: w102 -> [w1712]
    stop <- FALSE stop-if-true
    n816 = Get Queue Status(queue=w1713) -> (queue out=w1715:refnum<queue>, # elements in queue=w1716:i32)  [unwired: 2 in, 6 out]
    "# queue 2" <- w1716
    n817 = Wait (ms)(milliseconds to wait=u32 20) -> ()  [unwired: 1 out]
    n818 = local read "Save"() -> (w1710:bool)
    n819 = case shown="True" w1710 {
      tunnel: w1716 -> [_ w1748]
      tunnel: w1715 -> [_ w1750]
      tunnel: w1712 -> [_ w1747]
      frame False {
      }
      frame True {
        n820 = Multiply(x=w1748, y=w1747) -> (x*y=w1719:dbl)
        n821 = local read "date time rec"() -> (w1740:T2)
        n822 = for {
          N: w1748 -> [_]
          tunnel: [w1820] -> w1749 mode=indexing
          tunnel: [w1818] -> w1746 mode=indexing
          shift-right: [w1816] -> _
          shift-left: w1750 -> [w1822]
          tunnel: [w1812] -> w1721 mode=indexing
          tunnel: [w1811] -> w1720 mode=indexing
          i -> [w1817]
          n823 = Dequeue Element(queue=w1822) -> (queue out=w1816:refnum<queue>, element=w1813:dbl[][])  [unwired: 2 in, 2 out]
          n824 = Index Array(array=w1813, index (row)=2) -> (element=w1812:dbl[])  [unwired: 1 in]
          n825 = Index Array(array=w1813, index (row)=3) -> (element=w1811:dbl[])  [unwired: 1 in]
          n826 = Index Array(array=w1813, index (row)=1) -> (element=w1818:dbl[])  [unwired: 1 in]
          n827 = Index Array(array=w1813, index (row)=0) -> (element=w1820:dbl[])  [unwired: 1 in]
          "IterationNum" <- w1817
        }
        n828 = Unbundle By Name(w1740) -> ("fractional second"=w1733:dbl, "second"=w1734:i32, "minute"=w1735:i32, "hour"=w1736:i32, "day of month"=w1737:i32, "month"=w1738:i32, "year"=w1739:i32)
        n829 = property on="month" class="DigNum (strict)"() -> ("Label.Text"=w1730:string)  [unwired: 2 in, 2 out]
        n830 = property on="year" class="DigNum (strict)"() -> ("Label.Text"=w1731:string)  [unwired: 2 in, 2 out]
        n831 = property on="hour" class="DigNum (strict)"() -> ("Label.Text"=w1728:string)  [unwired: 2 in, 2 out]
        n832 = property on="day" class="DigNum (strict)"() -> ("Label.Text"=w1729:string)  [unwired: 2 in, 2 out]
        n833 = property on="fractionalSecond" class="DigNum (strict)"() -> ("Label.Text"=w1725:string)  [unwired: 2 in, 2 out]
        n834 = property on="second" class="DigNum (strict)"() -> ("Label.Text"=w1726:string)  [unwired: 2 in, 2 out]
        n835 = property on="minute" class="DigNum (strict)"() -> ("Label.Text"=w1727:string)  [unwired: 2 in, 2 out]
        n836 = Format Date/Time String(time format string (%c)="%m%d_%H%M%S") -> (date/time string=w1723:string)  [unwired: 2 in]
        n837 = property on="Routine" class="Ring (strict)"() -> ("RingText.Text"=w1742:string)  [unwired: 2 in, 2 out]
        n838 = Concatenate Strings(w1723, w1742) -> (w1741:string)
        n839 = flat-sequence {
          tunnel: w1741 -> [w1800]
          tunnel: path "E:/NCS/HumanStudyMarch2019/Data" ("base path") -> [w1806]
          tunnel: "Case Number" -> [w1803]
          tunnel: w1744 -> [w1765]
          tunnel: w1743 -> [w1764]
          tunnel: w1739 -> [w1797]
          tunnel: w1738 -> [w1792]
          tunnel: w1737 -> [w1787]
          tunnel: w1736 -> [w1786]
          tunnel: w1735 -> [w1785]
          tunnel: w1734 -> [w1780]
          tunnel: w1733 -> [w1779]
          tunnel: w1731 -> [w1778]
          tunnel: w1730 -> [w1777]
          tunnel: w1729 -> [w1776]
          tunnel: w1728 -> [w1775]
          tunnel: w1727 -> [w1774]
          tunnel: w1726 -> [w1773]
          tunnel: w1725 -> [w1772]
          tunnel: "Comments" -> [w1767]
          tunnel: w1718 -> [w1756]
          tunnel: w1717 -> [w1755]
          frame #0 {
            n840 = Build Path(base path=w1806, name or relative path=w1800) -> (appended path=w1809:path)
            n841 = TDMS Open(6:FALSE ("disable buffering (T)"), 10:T12."open or create" ("operation"), 11:w1809) -> (0:w1804:errorcluster, 3:w1805:refnum<k34>)  [unwired: 4 in]
            n842 = TDMS Set Properties(5:w1803, 7:"CaseNumber" ("property names"), 8:w1804, 11:w1805) -> (0:w1751:errorcluster, 3:w1752:refnum<k34>)  [unwired: 2 in, 2 out]
            n843 = TDMS Set Properties(5:w1767, 7:"Comments" ("property names"), 8:w1751, 11:w1752) -> (0:w1768:errorcluster, 3:w1769:refnum<k34>)  [unwired: 2 in, 2 out]
            n844 = TDMS Set Properties(5:w1797, 7:w1778, 8:w1768, 11:w1769) -> (0:w1796:errorcluster, 3:w1795:refnum<k34>)  [unwired: 2 in, 2 out]
            n845 = TDMS Set Properties(5:w1792, 7:w1777, 8:w1796, 11:w1795) -> (0:w1794:errorcluster, 3:w1793:refnum<k34>)  [unwired: 2 in, 2 out]
            n846 = TDMS Set Properties(5:w1787, 7:w1776, 8:w1794, 11:w1793) -> (0:w1791:errorcluster, 3:w1790:refnum<k34>)  [unwired: 2 in, 2 out]
            n847 = TDMS Set Properties(5:w1786, 7:w1775, 8:w1791, 11:w1790) -> (0:w1789:errorcluster, 3:w1788:refnum<k34>)  [unwired: 2 in, 2 out]
            n848 = TDMS Set Properties(5:w1785, 7:w1774, 8:w1789, 11:w1788) -> (0:w1784:errorcluster, 3:w1783:refnum<k34>)  [unwired: 2 in, 2 out]
            n849 = TDMS Set Properties(5:w1780, 7:w1773, 8:w1784, 11:w1783) -> (0:w1781:errorcluster, 3:w1782:refnum<k34>)  [unwired: 2 in, 2 out]
            n850 = TDMS Set Properties(5:w1779, 7:w1772, 8:w1781, 11:w1782) -> (0:w1770:errorcluster, 3:w1771:refnum<k34>)  [unwired: 2 in, 2 out]
            n851 = TDMS Write(0:w1771, 7:"Tx1Rx1Amp" ("channel name(s) in (Untitled)"), 9:w1764, 11:w1770) -> (4:w1799:refnum<k34>, 15:w1798:errorcluster)  [unwired: 2 in, 2 out]
            n852 = TDMS Write(0:w1799, 7:"Tx2Rx2Amp" ("channel name(s) in (Untitled)"), 9:w1765, 11:w1798) -> (4:w1762:refnum<k34>, 15:w1759:errorcluster)  [unwired: 2 in, 2 out]
            n853 = TDMS Write(0:w1762, 7:"Tx1Rx1Ph" ("channel name(s) in (Untitled)"), 9:w1755, 11:w1759) -> (4:w1761:refnum<k34>, 15:w1758:errorcluster)  [unwired: 2 in, 2 out]
            n854 = TDMS Write(0:w1761, 7:"Tx2Rx2Ph" ("channel name(s) in (Untitled)"), 9:w1756, 11:w1758) -> (4:w1760:refnum<k34>, 15:w1757:errorcluster)  [unwired: 2 in, 2 out]
            n855 = TDMS Close(8:w1757, 11:w1760) -> ()  [unwired: 2 out]
          }
          frame #1 {
            n856 = local write "Save"(FALSE) -> ()
          }
        }
        n857 = Reshape Array(w1720, w1719) -> (w1718:dbl[])
        n858 = Reshape Array(w1721, w1719) -> (w1717:dbl[])
        n859 = Reshape Array(w1746, w1719) -> (w1744:dbl[])
        n860 = Reshape Array(w1749, w1719) -> (w1743:dbl[])
      }
    }
  }
  n861 = local read "DownSamplingRatio"() -> (w117:i32)
  n862 = local read "Waveform Size"() -> (w118:dbl)
  n863 = Divide(x=w118, y=w117) -> (x/y=w105:dbl)
  n864 = Divide(x=w105, y="DownSamplingRatio 2") -> (x/y=w94:dbl)
  n865 = Multiply(x=w96, y=w94) -> (x*y=w112:dbl)
  n866 = Initialize Array(w95, w96, w94) -> (w114:dbl[][])
  n867 = Initialize Array(w95, w96, w94) -> (w113:dbl[][])
  n868 = Initialize Array(w95, w96, w94) -> (w116:dbl[][])
  n869 = Initialize Array(w95, w96, w94) -> (w115:dbl[][])
  n870 = while {
    tunnel: w96 -> [w1894]
    tunnel: w89 -> [w1887]
    shift-right: [w1884] -> _
    shift-left: w116 -> [w1856]
    tunnel: w112 -> [w1845]
    shift-right: [w1875] -> _
    shift-left: w115 -> [w1890]
    shift-right: [w1874] -> _
    shift-left: w114 -> [w1889]
    shift-right: [w1873] -> _
    shift-left: w113 -> [w1888]
    tunnel: "DownSamplingRatio 2" -> [w1826]
    tunnel: w94 -> [w1827]
    tunnel: "DownSamplingRatio 2" -> [w1846]
    stop <- FALSE stop-if-true
    # "Amp2"
    # "Amp1"
    # "Downsampling only for viewing."
    n871 = local read "Sampling Rate"() -> (w1847:dbl)
    n872 = Get Queue Status(queue=w1887) -> (# elements in queue=→"# elements in queue":i32)  [unwired: 2 in, 7 out]
    n873 = Dequeue Element(queue=w1887) -> (element=w1828:dbl[][])  [unwired: 2 in, 3 out]
    n874 = Decrement(x=w1894) -> (x-1=w1843:i32)
    n875 = Divide(x=w1847, y=w1846) -> (x/y=→"Dis Sampling Rate":dbl)
    n876 = Index Array(array=w1828, index (row)=0 ("index")) -> (element=w1854:dbl[])  [unwired: 1 in]
    n877 = Index Array(array=w1828, index (row)=1 ("index")) -> (element=w1853:dbl[])  [unwired: 1 in]
    n878 = Index Array(array=w1828, index (row)=2 ("index")) -> (element=w1834:dbl[])  [unwired: 1 in]
    n879 = Index Array(array=w1828, index (row)=3 ("index")) -> (element=w1833:dbl[])  [unwired: 1 in]
    n880 = Reshape Array(w1853, w1827, w1826) -> (w1850:dbl[][])
    n881 = Reshape Array(w1854, w1827, w1826) -> (w1852:dbl[][])
    n882 = Reshape Array(w1834, w1827, w1826) -> (w1832:dbl[][])
    n883 = Reshape Array(w1833, w1827, w1826) -> (w1831:dbl[][])
    n884 = for {
      tunnel: w1850 -> [w1908] mode=indexing
      tunnel: [w1907] -> w1849 mode=indexing
      n885 = Add Array Elements(numeric array=w1908) -> (sum=w1907:dbl)
    }
    n886 = for {
      tunnel: w1832 -> [w1906] mode=indexing
      tunnel: [w1905] -> w1830 mode=indexing
      n887 = Add Array Elements(numeric array=w1906) -> (sum=w1905:dbl)
    }
    n888 = for {
      tunnel: w1831 -> [w1904] mode=indexing
      tunnel: [w1903] -> w1829 mode=indexing
      n889 = Add Array Elements(numeric array=w1904) -> (sum=w1903:dbl)
    }
    n890 = for {
      tunnel: w1852 -> [w1910] mode=indexing
      tunnel: [w1909] -> w1851 mode=indexing
      n891 = Add Array Elements(numeric array=w1910) -> (sum=w1909:dbl)
    }
    n892 = Array Subset(array=w1889, index (row)=0 ("index"), length (row)=w1843) -> (w1877:dbl[][])  [unwired: 2 in]
    n893 = Array Subset(array=w1888, index (row)=0 ("index"), length (row)=w1843) -> (w1876:dbl[][])  [unwired: 2 in]
    n894 = Array Subset(array=w1890, index (row)=0 ("index"), length (row)=w1843) -> (w1878:dbl[][])  [unwired: 2 in]
    n895 = Array Subset(array=w1856, index (row)=0 ("index"), length (row)=w1843) -> (w1885:dbl[][])  [unwired: 2 in]
    n896 = Divide(x=w1851, y=w1826) -> (x/y=w1837:dbl[])
    n897 = Divide(x=w1849, y=w1826) -> (x/y=w1824:dbl[])
    n898 = Divide(x=w1830, y=w1826) -> (x/y=w1825:dbl[])
    n899 = Divide(x=w1829, y=w1826) -> (x/y=w1823:dbl[])
    n900 = Build Array (concatenate)(w1823, w1876) -> (w1873:dbl[][])
    n901 = Build Array (concatenate)(w1825, w1877) -> (w1874:dbl[][])
    n902 = Build Array (concatenate)(w1824, w1878) -> (w1875:dbl[][])
    n903 = local read "Dis Sampling Rate"() -> (w1844:dbl)
    n904 = Build Array (concatenate)(w1837, w1885) -> (w1884:dbl[][])
    n905 = Reshape Array(w1873, w1845) -> (w1858:dbl[])
    n906 = Reshape Array(w1874, w1845) -> (w1857:dbl[])
    n907 = Reshape Array(w1875, w1845) -> (w1859:dbl[])
    n908 = disable-structure shown="Enabled" {
      disable-tunnel: w1837 -> [w1900 _]
      disable-tunnel: w1825 -> [w1899 _]
      disable-tunnel: w1824 -> [w1902 _]
      disable-tunnel: w1823 -> [w1901 _]
      frame Enabled {
        "Amp2 @500Hz" <- w1902
        "Ph2 @500Hz" <- w1901
        "Amp1 @500Hz" <- w1900
        "Ph1 @500Hz" <- w1899
      }
      frame Disabled {
      }
    }
    n909 = Reshape Array(w1884, w1845) -> (w1860:dbl[])
    n910 = call-poly <vilib>:"Butterworth Filter.vi"("init/cont (init:F)"=TRUE, "order"=3, "filter type"=Filter_Passband_Type."Bandpass", "low cutoff freq: fl"="fl 3", "high cutoff freq: fh"="fh 3", "sampling freq: fs"=w1844, "X"=w1857) -> ("Filtered X"=w1839:dbl[])  [unwired: 1 in, 1 out]
    n911 = call-poly <vilib>:"Butterworth Filter.vi"("init/cont (init:F)"=TRUE, "order"=3, "filter type"=Filter_Passband_Type."Lowpass", "low cutoff freq: fl"="fl 4", "sampling freq: fs"=w1844, "X"=w1858) -> ("Filtered X"=w1838:dbl[])  [unwired: 2 in, 1 out]
    n912 = call-poly <vilib>:"Butterworth Filter.vi"("init/cont (init:F)"=TRUE, "order"=3, "filter type"=Filter_Passband_Type."Lowpass", "low cutoff freq: fl"="fl 2", "sampling freq: fs"=w1844, "X"=w1859) -> ("Filtered X"=w1861:dbl[])  [unwired: 2 in, 1 out]
    n913 = call-poly <vilib>:"Butterworth Filter.vi"("init/cont (init:F)"=TRUE, "order"=3, "filter type"=Filter_Passband_Type."Bandpass", "low cutoff freq: fl"="fl 1", "high cutoff freq: fh"="fh 1", "sampling freq: fs"=w1844, "X"=w1860) -> ("Filtered X"=w1862:dbl[])  [unwired: 1 in, 1 out]
    n914 = Build Array(w1862, w1861, w1839, w1838) -> (→"aapp":dbl[][])
  }
  n915 = while {
    stop <- FALSE stop-if-true
    n916 = local read "aapp"() -> (w1914:dbl[][])
    n917 = Index Array(array=w1914, index (row)=0 ("index")) -> (element=→"Heart Amp":dbl[])  [unwired: 1 in]
    n918 = Index Array(array=w1914, index (row)=1 ("index")) -> (element=→"Resp Amp":dbl[])  [unwired: 1 in]
    n919 = Index Array(array=w1914, index (row)=2 ("index")) -> (element=→"Heart Ph":dbl[])  [unwired: 1 in]
    n920 = Index Array(array=w1914, index (row)=3 ("index")) -> (element=→"Resp Ph":dbl[])  [unwired: 1 in]
    n921 = Wait (ms)(milliseconds to wait=u32 20) -> ()  [unwired: 1 out]
  }
  "error out" <- w76
  "error out 2" <- w75
